vi "BIMS_Collector (2012_01).vi"() -> ()   [LabVIEW 2015]
doc: "This program is currently beta software. It is designed to address the data requirements defined primarily by the DHB Ballistic Test Report.\n\nThe general operation of this program is based on the Ballistics Version 2005 application developed internally by DuPont as a research tool for the Spruance Plant Ballistics Lab in Richmond, VA.\n\nPlease note that the original trigger control logic was modified and no longer depends on a safety interlock system to enable operation of a ballistic test.\n\nDuPont makes no warranties and assumes no liabilities in connection with any use of this program."
uses:
  <vilib>/addons/database/NI_Database_API.lvlib
  <vilib>/addons/database/Connection.llb/Conn Execute.vi
  <vilib>/addons/database/Recordset.llb/Rec Destroy - Connection.vi
  <vilib>/Utility/config.llb/NI_LVConfig.lvlib
  <vilib>/Utility/config.llb/Write Key (I32).vi
  Shot Record.ctl
  BIMS_Collector Globals.vi
  Collector State.ctl
  DataSource.ctl
  <vilib>/registry/registry.llb/Registry RtKey.ctl
  <vilib>/Utility/config.llb/Write Key (String).vi
  <vilib>/addons/database/Connection.llb/DB Tools Open Connec (Path).vi
panel:
  out "Loading":u16(ring)
  in  "runtimeMenusVisible":bool=TRUE
  in  "diagPageVisible":bool
  in  "RESET All":bool
  out "ConfigName":string
  out "TimeNow":string
  in  "EXIT":bool
  in  "mainTabCntrl":enum32{"Setup", "Measure", "History", "System"}(tab)=enum."System"
  in  "SampleEntryTabCntrl":enum32{"Environment", "Sample"}(tab)
  in  "ThreatDetails":u16(ring) caption="Detail"
  in  "ThreatGroups":u16(ring) caption="Group"
  in  "PowderTypes":u16(ring) caption="Type"
  in  "Ballisticians":u16(ring) caption="Ballistician"
  in  "Recorders":u16(ring) caption="Recorder"
  in  "Shooters":u16(ring) caption="Shooter"
  in  "Methods":u16(ring) caption="Method"
  in  "RoomT":sgl caption="Temperature (° F)" format="%.1f"
  in  "RoomHum":sgl caption="Humidity (%)" min=0 max=100 format="%.1f"
  in  "SampleBackings":u16(ring)=3 caption="Type"
  in  "clayCalArray":i16[](array[numeric])=[0, 0, 0, 0, 0] caption="Calibration (mm)" min=0 max=99 format="%02.0f"
  out "clayAverage":sgl caption="Clay Average (mm)" format="%#.1f"
  in  "clayTemp":sgl caption="Clay Temp (° F)" format="%.1f"
  out "threatDetails":T1 caption="Description"
  in  "SampleClamping":u16(ring) caption="Clamping"
  in  "Sample SubTabCntrl":T2(tab)
  in  "SampleID":string caption="Sample ID"
  in  "SampleDimensions":u16(ring) caption="Dimensions"
  in  "ModelMfrs":u16(ring) caption="Manufacturer" items=["DuPont Experimental"]
  in  "SampleTypes":u16(ring) caption="Sample Type"
  in  "Submitters":u16(ring) caption="Submitter"
  in  "ProjectID":string caption="Project ID"
  in  "BackLayers":i32 caption="# of Layers" min=0 max=99 step=5
  in  "FrontLayers":i32 caption="# of Layers" min=0 max=99 step=5
  in  "BackLayer":u16(ring) caption="Back Layer"
  in  "FrontLayer":u16(ring) caption="Front Layer"
  out "totalNumLayers":i32 caption="Total # of Layers" min=0 max=100 step=5
  out "totalBAW":sgl caption="Total BAW (psf)" format="%.2f"
  in  "LayerTabControl":enum32{"1", "2", "3", "4", "5", "6"}(tab) caption="Inner Layers"
  out "fab1_totalWt":sgl caption="Fab1 Wt" min=0 max=99 step=5 format="%.2f"
  out "SampleAttribs_1":T3 caption="fabricAttribs_1"
  in  "Layer_1":T4 caption="Fabric #1" {"plyNum" min=0 max=99 step=5}
  in  "SampleStyle_1":u16(ring)
  in  "Mfr_1":u16(ring) caption="vendor" items=["", "DuPont"]
  in  "layerStitch_1":u16(ring) caption="Stitch" items=["", "1-inch quilt", "2-inch quilt", "Corner Bartack", "Corners", "Custom (Panel)", "Custom (Vest)", "Diamond", "Edge", "n/a", "Normal"]
  out "fab2_totalWt":sgl caption="Fab2 Wt" min=0 max=99 step=5 format="%.2f"
  out "SampleAttribs_2":T3 caption="fabricAttribs_2"
  in  "Layer_2":T4 caption="Fabric #2" {"plyNum" min=0 max=99 step=5}
  in  "SampleStyle_2":u16(ring)
  in  "Mfr_2":u16(ring) caption="vendor" items=["", "DuPont"]
  in  "layerStitch_2":u16(ring) caption="Stitch" items=["", "1-inch quilt", "2-inch quilt", "Corner Bartack", "Corners", "Custom (Panel)", "Custom (Vest)", "Diamond", "Edge", "n/a", "Normal"]
  out "fab3_totalWt":sgl caption="Fab3 Wt" min=0 max=99 step=5 format="%.2f"
  out "SampleAttribs_3":T3 caption="fabricAttribs_3"
  in  "Layer_3":T4 caption="Fabric #3" {"plyNum" min=0 max=99 step=5}
  in  "SampleStyle_3":u16(ring)
  in  "Mfr_3":u16(ring) caption="vendor" items=["", "DuPont"]
  in  "layerStitch_3":u16(ring) caption="Stitch" items=["", "1-inch quilt", "2-inch quilt", "Corner Bartack", "Corners", "Custom (Panel)", "Custom (Vest)", "Diamond", "Edge", "n/a", "Normal"]
  out "fab4_totalWt":sgl caption="Fab4 Wt" min=0 max=99 step=5 format="%.2f"
  out "SampleAttribs_4":T3 caption="fabricAttribs_4"
  in  "Layer_4":T4 caption="Fabric #4" {"plyNum" min=0 max=99 step=5}
  in  "SampleStyle_4":u16(ring)
  in  "Mfr_4":u16(ring) caption="vendor" items=["", "DuPont"]
  in  "layerStitch_4":u16(ring) caption="Stitch" items=["", "1-inch quilt", "2-inch quilt", "Corner Bartack", "Corners", "Custom (Panel)", "Custom (Vest)", "Diamond", "Edge", "n/a", "Normal"]
  out "fab5_totalWt":sgl caption="Fab5 Wt" min=0 max=99 step=5 format="%.2f"
  out "SampleAttribs_5":T3 caption="fabricAttribs_5"
  in  "Layer_5":T4 caption="Fabric #5" {"plyNum" min=0 max=99 step=5}
  in  "SampleStyle_5":u16(ring)
  in  "Mfr_5":u16(ring) caption="vendor" items=["", "DuPont"]
  in  "layerStitch_5":u16(ring) caption="Stitch" items=["", "1-inch quilt", "2-inch quilt", "Corner Bartack", "Corners", "Custom (Panel)", "Custom (Vest)", "Diamond", "Edge", "n/a", "Normal"]
  out "fab6_totalWt":sgl caption="Fab6 Wt" min=0 max=99 step=5 format="%.2f"
  out "SampleAttribs_6":T3 caption="fabricAttribs_6"
  in  "Layer_6":T4 caption="Fabric #6" {"plyNum" min=0 max=99 step=5}
  in  "SampleStyle_6":u16(ring)
  in  "Mfr_6":u16(ring) caption="vendor" items=["", "DuPont"]
  in  "layerStitch_6":u16(ring) caption="Stitch" items=["", "1-inch quilt", "2-inch quilt", "Corner Bartack", "Corners", "Custom (Panel)", "Custom (Vest)", "Diamond", "Edge", "n/a", "Normal"]
  in  "SampleCoverings":u16(ring) caption="Sample Covering" items=["None", "RipStop", "Plastic bag", "Other"]
  in  "Assemblers":u16(ring) caption="Technician"
  in  "Thickness":dbl caption="Thickness (in)" format="%.3f"
  in  "totalSampleWt":sgl caption="Total Weight (lbs)" format="%.3f"
  in  "Comments":string caption="Remarks (optional):"
  in  "TestConditions":u16(ring) caption="Sample Condition"
  in  "shotsTabCntrl":T5(tab)
  in  "Frag Rod":sgl format="%.1f"
  in  "MeasSrc":T6=enum."Screens" caption="Source"
  in  "Drag Corrected":bool=TRUE
  in  "ARM":bool
  in  "readyClock":bool caption="Clock"
  out "Impact/speed":sgl caption="Chronograph 1" min=0 max=10000 step=0.1 format="%.1f"
  out "SHOT STATUS":u16(ring) caption="Penetration" items=["Partial", "Complete"]
  out "residual/speed":sgl caption="Residual" min=0 max=10000 step=0.1 format="%.1f"
  out "SUBMIT DATE/TIME":string
  out "BACKFACE DEPTH":sgl caption="Backface\nDepth" min=0 max=200 step=5
  in  "MeasVelScrnSet1":sgl caption="Set #1" min=0 max=10000 step=0.1 format="%.1f"
  in  "Current/sthotstatus":u16(ring) caption="Penetration" items=["Partial", "Complete"]
  in  "Current/residual/speed":sgl caption="Residual Set" min=0 max=10000 step=0.1 format="%.1f"
  in  "currentDateTime":string caption="Date/Time"
  in  "MeasVelScrnSet2":sgl caption="Set #2" min=0 max=1000000 step=0.1 format="%.1f"
  out "%_Difference":sgl caption="% Vel Diff" format="%.3f"
  in  "backdepth":sgl caption="BF Depth"
  out "Redundant/speed":sgl caption="Chronograph 2" min=0 max=10000 step=0.1 format="%.1f"
  out "Current/avg/speed":sgl caption="Average" min=0 max=1000000 step=0.1 format="%.1f"
  out "Avg/speed":sgl caption="Average" min=0 max=10000 step=0.1 format="%.1f"
  out "SafetyInterlock":cluster{"ARMED":bool}
  out "DC_ factor":sgl=1.0 caption="DC Factor" format="%.4f"
  in  "Barrel Temp":sgl format="%.1f"
  in  "Shot Description":string caption="Description (optional)"
  in  "Powder Loading":sgl caption="Powder Load" min=0 max=100 step=0.1 format="%.3f"
  in  "Shot Angle":u16 max=90 step=1
  out "Projectile Mass":sgl caption="Projectile Mass (grains)" min=0 step=1
  in  "N.I.J":u16(ring) items=["n/a", "PASS", "FAIL"]
  out "Device S/N":string
  in  "addShot":bool caption="RANGE SETUP must be selected before shots can be added."
  in  "loadingUnits":enum32{"grams", "grains"}(radio)
  out "instruct_addShot":string="RANGE SETUP and THREAT must be selected before shots can be added."
  out "Set#1 Separation":sgl=4.0 caption="Outer" format="%.2f"
  out "Set#2 Separation":sgl=4.0 caption="Inner" format="%.2f"
  out "saveReq":string="Number of layers in sample ply specification and number of shots in shots table must be greater than 0 to enable saving."
  in  "VsVr Report":bool caption="Report"
  out "Table of Shots":string[][](table) caption="Shot Table"
  in  "MC Listbox of Shots":i32(listbox)
  in  "saveShots":bool
  in  "clearShots":bool
  out "highPartial":i32 caption="High Partial" min=0 max=10000 step=1
  out "lowComplete":i32 caption="Low Complete" min=0 max=10000 step=1
  out "rangeOfResults":i32 caption="Range of Results" min=0 max=10000 step=1
  out "zmr 2":sgl caption="Low C minus High P" format="%.1f"
  out "computed_V50":sgl caption="V50" format="%.1f"
  out "Pairs":i16 min=0 max=100 step=1
  in  "reportV50":bool caption="Report"
  in  "maxDev":sgl=125.0 caption="Max Deviation" min=0 max=300 step=25
  in  "undoLastShot":bool
  in  "deleteShot":bool
  in  "nextShot":bool
  in  "SHOTS":T7[](array[typedef]) {"Frag Rod" format="%.1f"; "UncorrectedAvgVel_PB" format="%.1f"; "UncorrectedRed_PB" format="%.1f"; "strikeVel_PB" format="%.1f"; "velLoss_PB" format="%.1f"; "avgVel_PB" format="%.1f"; "Redundant_Velocity" format="%.1f"; "Energy Loss (J)" format="%.3e"; "Projectile Mass" min=0 step=1 format="%.4f"; "Corrected residual" format="%.2f"; "Uncorrected Residual" format="%.1f"; "Corrected Impact" format="%.2f"; "Uncorrected Impact" format="%.1f"; "Shot Angle" max=90 step=1; "SHOT STATUS" items=["Partial", "Complete"]; "IMPACT VELOCITY" min=0 max=10000 step=0.1 format="%.1f"; "Barrel Temperature" format="%.1f"; "Powder Loading" format="%.4f"; "RESIDUAL  VELOCITY" min=0 max=10000 step=0.1 format="%.1f"}
  out "velProfile":cluster{dbl, dbl}[](graph) caption="Shot Velocity Measurement Profile"
  out "velCompProf":cluster{"vStrike":dbl, "vA":dbl} caption="Velocity in fps\n(computed)"
  out "velMeasProf":T8 caption="Velocity in fps\n(measured)"
  out "relativeTime":cluster{"ts2":dbl, "ts3":dbl, "ts1":dbl} caption="Relative time\n(microsec)"
  out "displacement":T9={"ds_v2"=6.75, "ds2"=5.0833, "ds_vB"=4.9167, "ds3"=4.75, "ds_vAvg"=6.9167, "ds_v1"=7.0833, "ds1"=8.75, "ds_vA"=8.9167, "ds0"=9.0833} caption="Distance from\ntarget (ft)" {"ds0" format="%_4g"; "ds_vA" format="%_4g"; "ds1" format="%_4g"; "ds_v1" format="%_4g"; "ds_vAvg" format="%_4g"; "ds3" format="%_4g"; "ds_vB" format="%#_4g"; "ds2" format="%#_4g"; "ds_v2" format="%_4g"}
  out "arrIDC":dbl[](array[numeric]) caption="Instantaneous Drag Coefficient"
  in  "rangeSetup":u16(ring)=1 caption="Range Dimensions" items=["Short (small frag)", "Standard (handgun)", "Long (rifle)"]
  out "mid_to_targ_dist":sgl=5.0 caption="Mid To Target (ft)"
  in  "historyTabCntrl":enum32{"Powder Loading", "Panel Search"}(tab)=enum."Panel Search"
  in  "Threat.freeTxt":string caption="Threat"
  in  "Powder.freeTxt":string caption="Powder"
  in  "QueryLoad":bool
  in  "lkupEndDate":timestamp caption="End Date" format="%<%x>T"
  in  "lkupStartDate":timestamp caption="Begin Date" format="%<%x>T"
  out "Vel.vs.Loading":cluster{dbl[], dbl[]}(graph)
  out "v50_table":string[][](table)
  in  "maxRecs":u16=1001 caption="Max # of SHOT Records" min=1 max=10000 step=100
  out "ActualNumRecs":i32=1001 caption="Actual # Returned"
  in  "ThreatSize_0":u16(ring) caption="Threat Size" items=["", "2"]
  in  "panelSearch":bool
  in  "Mfr_0":u16(ring) caption="Manufacturer" items=["", "DuPont"]
  in  "SampleStyle_0":u16(ring) caption="Sample Style"
  in  "srchParams":T10={"maxPanels"=1001, "lkupPanelStartDate"=timestamp(0 s since 1904-01-01), "lkupPanelEndDate"=timestamp(3376658114.0909824 s since 1904-01-01)} {"lkupPanelEndDate" format="%<%x>T"; "lkupPanelStartDate" format="%<%x>T"; "maxPanels" min=1 max=10000 step=100}
  out "actualNumPanels":i32 caption="Actual # Returned"
  out "pastPanels":string[][](table)
  in  "Record #":i32=1 min=0 max=13
  in  "reportV50_History":bool
  out "SampleAttribs_0":T11 caption="fabricAttribs_1"
  in  "Requestors_0":u16(ring) caption="Submitter"
  in  "aboutTabCntrl":enum32{"About ", "Internal Use"}(tab)
  in  "RefreshMetadata":bool
  out "LastShot":i32 caption="Shot"
  out "LastSample":i32 caption="Sample"
  in  "PublishNewRecords":bool
  in  "Folder":string="esvrs11" caption="Publish Folder"
  in  "useBMC":bool caption="Use Message Center?"
  in  "Server":string="esvrs11"
  in  "Site":string="ICE1"
  in  "TestStandards":u16(ring)=2 caption="Standard" items=["n/a", "NIJ 0101.04", "MIL-STD-662F"]
  in  "WeaponTypes":u16(ring) caption="Weapon" items=["", "Universal Receiver", "Other"]
  in  "processShots":bool
  out "DIO":u32=21 format="%.0b"
  in  "line direction map":i32=1792 format="%.0b"
  out "Corrected Average":sgl=1527.9313 format="%.2f"
  out "CorrectedVelScrnSet2":sgl=1551.8816 caption="Corrected Redundant" format="%.2f"
  out "conversion factor":sgl=0.3048037 format="%.5f"
  out "#_completes":i32
  out "#_partials":i32
  in  "percent warning":sgl=1.0 format="%.2f"
  in  "SoftwareVersion":dbl caption="Version" format="%.2f"
  out "impact/ID":u32=83886081 format="%.0x"
  out "residual/ID":u32=83951617 format="%.0x"
  out "Red/ID":u32=84017153 format="%.0x"
  out "correction coefficient":sgl format="%.8f"
  out "Corrected Residual":sgl=751.9905 format="%.2f"
  out "CorrectedVelScrnSet1":sgl=1503.981 format="%.2f"
  out "Barrel to Screen":sgl=7.8333 format="%.2f"
  in  "Set#1_to_Target":sgl=7.083333 format="%.2f"
  out "Residual/Separation":sgl=4.0 format="%.2f"
  in  "Residual/Target Dist":sgl=7.083333 format="%.2f"
  out "Z.M.R.":sgl min=0 step=0.1 format="%.1f"
  in  "old threat":u16
  out "Complete":sgl[](array[numeric]) format="%.2f"
  out "factor array":sgl[](array[numeric]) format="%.4f"
  out "Partial":sgl[](array[numeric]) format="%.2f"
  in  "DAQ Card":i16=1
  in  "Impact Timer":i16 min=0 max=3 step=1
  in  "Redundant Timer":i16=1 min=0 max=3 step=1
  in  "Residual  Timer":i16=2 min=0 max=3 step=1
  out "Impact factor":sgl=1.0 caption="Impact" min=0 max=1 format="%.5f"
  out "Residual factor":sgl=1.0 caption="Residual" min=0 max=1 format="%.5f"
  in  "Areal Density":dbl format="%.2f"
  in  "Areal density text":string
  in  "Fabric Description":string caption="Fabric Desc"
  in  "clayCalib":string="##-##-##-##-##" caption="Calibration"
  in  "lookupRec":bool caption="lookup"
  out "STOP (Shots MC LB)":bool=TRUE
  out "configPath":path=path "P:/Private/My Projects/AFS/BIMS/2008/BIMS_Collector.ini" caption="Configuration Path (INI)"
  in  "minV50":i32=1500 caption="Minimum V50"
  in  "Type of work":string="QC"
  in  "Threat":u16(ring) caption="Threat (long description)"
  out "massUnits":string="GRAMS" caption="Weight Units"
  out "lengthUnits":string="FOOT" caption="Distance Units"
  in  "SampleDescrip":u16(ring) caption="Misc. Sample Description (legacy)"
  in  "serialNum":string caption="Serial #"
  in  "Models":u16(ring) caption="Model #" items=["n/a"]
  in  "InterlockExists":bool=TRUE caption="Safety Interlock Hardware Exist?"
  in  "ScreenSetAvgg":bool caption="Average Screen Sets?"
  in  "Sort by AVG":bool=TRUE caption="Sort shots by average velocity"
  in  "useBallisitican":bool=TRUE caption="Use Ballistician field in Setup?"
  in  "useRecorder":bool caption="Use Recorder field in Setup?"
  in  "useShooter":bool caption="Use Shooter field in Setup?"
  out "SMErr":errorcluster
  out "U/I EvErr":errorcluster
  out "booleanDump":bool
  out "GrainSize":u16 caption="Grain"
  in  "LayerStitchTypes":u16(ring) caption="Stitch" items=["", "Corners"]
  in  "clearErrors":bool
  # "Effectively restarts the application from scratch, as if the user pressed the EXIT button and then restarted the application."
  # "Configured for"
  # "Threat"
  # "*"
  # "*"
  # "Test"
  # "Powder"
  # "*"
  # "Personnel"
  # "Room"
  # "*"
  # "Backing"
  # "*"
  # "*"
  # "*"
  # "Body Side"
  # "Strike Face"
  # "Layer"
  # "Mfr"
  # "Style"
  # "# of Plies"
  # "Lot"
  # "Roll"
  # "Stitch"
  # "Internal ID"
  # "Fiber"
  # "Denier"
  # "Construction"
  # "Weave"
  # "Finish"
  # "Basis weight (oz/yd²)"
  # "Yarn Merge"
  # "Total Weight"
  # "*"
  # "*"
  # "*"
  # "1"
  # "2"
  # "3"
  # "4"
  # "5"
  # "6"
  # "Required"
  # "*"
  # "Timing System"
  # "Shot Parameters"
  # "cm"
  # "deg"
  # "degF"
  # "Velocity Measurements"
  # "Observations"
  # "Screens\nSeparation"
  # "Ft"
  # "Table Functions"
  # "Summary"
  # "Reports"
  # "Test Record"
  # "Edit Shot Records"
  # "Corrected"
  # "Shot #"
  # "t0"
  # "0"
  # "S Strike"
  # "0"
  # "Internal ID#"
  # "Fiber"
  # "Denier"
  # "Pick"
  # "Weave"
  # "Finish"
  # "oz/yd²"
  # "Asset"
  # "DuPont Ballistics Information Management System\n\nBIMS\nEnterprise Edition\n\n\nSample Performance\nData Collector\n\nJanuary 2012"
  # "DuET Measurement System Technologies\nDUCOM 8 695-2330 for technical support\n\nDuPont Company"
  # "Last Assigned\nRecord Numbers"
  # "Deployment Configuration"
  # "Data items support Point Blank requirements:"
  # "Correction Factors"
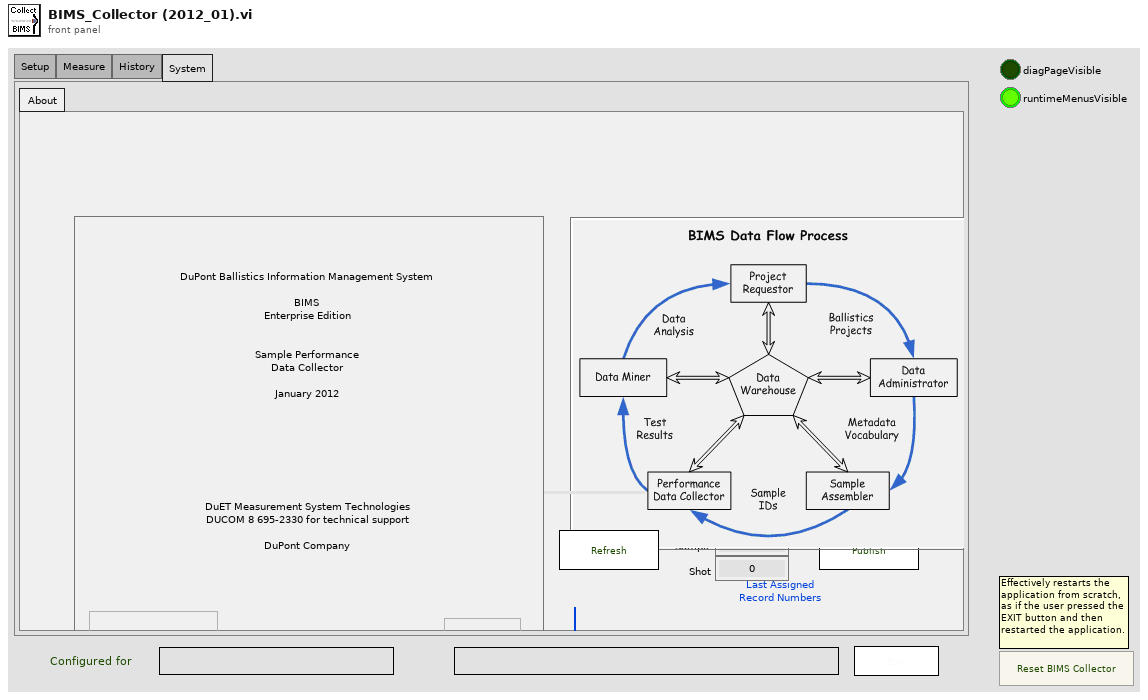
[diagram p1: front panel]
types:
  T1 = cluster{"barrelLength":string, "dragCorrection":string, "detailDescription":string, "barrelCaliber":string, "grainSize":string, "Make":string, "Model":string}
  T2 = enum32{"General Specification", "Ply Specification", "Preparation"}
  T3 = cluster{"Fabric.fiber":string, "Fabric.denier":string, "pick":string, "weave":string, "finish":string, "ozPerYd2":string, "fabricID_DHB":string, "yarnMerge":string}
  T4 = cluster{"plyNum":i32, "LotNum":string, "RollNum":string}
  T5 = enum32{"Ready-Aim-Fire", "Shots Table", "Edit", "Instantaneous DC"}
  T6 = typedef "DataSource.ctl" = enum16{"Simulated", "Radar", "Screens"}
  T7 = typedef "Shot Record.ctl" = cluster{"Uncorrected Impact":sgl, "Uncorrected Residual":sgl, "avgVel_PB":sgl, "IMPACT VELOCITY":sgl, "RESIDUAL  VELOCITY ":sgl, "Shot Description":string, "Powder Loading ":sgl, "Barrel Temperature":sgl, "TIME / DATE":string, "shot order":i32, "SHOT STATUS":u16, "Shot Angle":u16, "Corrected Impact":sgl, "Corrected residual":sgl, "Projectile Mass":sgl, "usedv50":bool, "Energy Loss (J)":sgl, "BackFace\nDepth":sgl, "BackFace\nDiameter":sgl, "Redundant_Velocity":sgl, "velLoss_PB":sgl, "strikeVel_PB":sgl, "UncorrectedRed_PB":sgl, "CorrectedRed_PB":sgl, "UncorrectedAvgVel_PB":sgl, "V50userExcl":bool, "Frag Rod":sgl}
  T8 = cluster{"v2":dbl, "vB":dbl, "vOuter":dbl, "v1":dbl, "vA":dbl, "vInner":dbl}
  T9 = cluster{"ds_v2":dbl, "ds2":dbl, "ds_vB":dbl, "ds3":dbl, "ds_vAvg":dbl, "ds_v1":dbl, "ds1":dbl, "ds_vA":dbl, "ds0":dbl}
  T10 = cluster{"maxPanels":u16, "lkupPanelStartDate":timestamp, "lkupPanelEndDate":timestamp}
  T11 = cluster{"Fabric.fiber":string, "Fabric.denier":string, "pick":string, "weave":string, "finish":string, "ozPerYd2":string, "fabricID_DHB":string, "asset":string}
  T12 = typedef "Collector State.ctl" = enum16{"POLL", "INITIALIZE", "V50 Report or GET Record", "VsVr Report", "SAVE SHOTS", "ADD SHOT", "CLEAR SHOTS", "NEXT SHOT", "DELETE SHOT", "READY CLOCK", "PROC SHOTS", "CHECK DAQ"}
  T13 = typedef "Collector State.ctl" = enum16{"POLL", "INITIALIZE", "V50 Report or GET Record", "VsVr Report", "SAVE SHOTS", "ADD SHOT", "CLEAR SHOTS", "NEXT SHOT", "DELETE SHOT", "PROCESS SHOTS", "READY CLOCK", "CHECK DAQ"}
  T14 = enum8{"Enabled", "Disabled", "Disabled and Grayed Out"}
  T15 = enum32{"Page Enabled", "Page Disabled", "Page Disabled & Grayed"}
  T16 = typedef "Registry RtKey.ctl" = enum32{"HKEY_CLASSES_ROOT", "HKEY_CURRENT_USER", "HKEY_LOCAL_MACHINE", "HKEY_USERS", "HKEY_PERFORMANCE_DATA", "HKEY_CURRENT_CONFIG", "HKEY_DYN_DATA"}
  T17 = cluster{"[0]":string, "[1]":string, "[2]":string, "[3]":string, "[4]":string, "[5]":string, "[6]":string, "[7]":string, "[8]":string, "[9]":string}[]
  T18 = cluster{"[0]":string, "[1]":string, "[2]":string, "[3]":string, "[4]":string, "[5]":string, "[6]":string, "[7]":string, "[8]":string}[]
  T19 = cluster{"Fabric.fiber":string, "Fabric.denier":string, "pick":string, "weave":string, "finish":string, "ozPerYd2":string, "fabricID_DHB":string, "yarnMerge":string}[]
  T20 = cluster{"Uncorrected Impact":bool, "Uncorrected Residual":bool, "avgVel_PB":bool, "IMPACT VELOCITY":bool, "RESIDUAL  VELOCITY ":bool, "Shot Description":bool, "Powder Loading ":bool, "Barrel Temperature":bool, "TIME / DATE":bool, "shot order":bool, "SHOT STATUS":bool, "Shot Angle":bool, "Corrected Impact":bool, "Corrected residual":bool, "Projectile Mass":bool, "usedv50":bool, "Energy Loss (J)":bool, "BackFace\nDepth":bool, "BackFace\nDiameter":bool, "Redundant_Velocity":bool, "velLoss_PB":bool, "strikeVel_PB":bool, "UncorrectedRed_PB":bool, "CorrectedRed_PB":bool, "UncorrectedAvgVel_PB":bool, "V50userExcl":bool, "Frag Rod":bool}
  T21 = cluster{"SampleTypes":refnum<vi>, "SampleDescrip":refnum<vi>}
  T22 = cluster{"max dev":sgl, "residual separation":sgl, "Set#1 Separation":sgl, "Set#2 Separation ":sgl, "impact target dist":sgl, "resid target dist":sgl, "barrel screen dist":sgl, "midpt_to_target_dist":sgl}
  T23 = cluster{"fiber":string, "denier":string, "pick":string, "weave":string, "finish":string, "ozPerYd2":string, "internal_ID":string, "asset":string}[]
  T24 = cluster{"numOfPlies":i32, "LotNum":string, "RollNum":string}[]
  T25 = cluster{string, string, string, string, string, string, string, string, "clayCalib":string, string}
  T26 = cluster{string, string, string, string, string, string, string}
  T27 = cluster{"SampleID":string, "element":string, "Type of work":string, "serialNum":string, "element":string, string, string, string, "element":string, string}
  T28 = cluster{"SampleID":string, "element":string, string, string, string, "element":string}
  T29 = cluster{"[0]":string, "[1]":string, "[2]":string, "[3]":string, "[4]":string, "[5]":string, "[6]":string, "[7]":string, "[8]":string, "[9]":string}
  T30 = cluster{"[0]":string, "[1]":string, "[2]":string, "[3]":string, "[4]":string, "[5]":string, "[6]":string, "[7]":string, "[8]":string}
  T31 = cluster{"element":string, "element":string, "grainSize":string, "element":string, "barrelLength":string, string, "element":string, "element":string, "element":string}
  T32 = cluster{"element":string, "grainSize":string, "element":string, "barrelLength":string, string, "element":string}
  T33 = typedef "NI_Database_API.lvlib/Conn ObjectReference.ctl" = refnum<k1>
  T34 = typedef "NI_Database_API.lvlib/Rec ObjectReference.ctl" = refnum<k1>
  T35 = typedef "NI_LVConfig.lvlib/Config Data RefNum.ctl" = refnum<k1>
  T36 = cluster{"task ID out":u32, "task ID out":u32, "task ID out":u32}
  T37 = enum32{"invalid app kind", "Development System", "Run Time System", "Student Edition", "Embedded LabVIEW", "Evaluation", "Custom"}
  T38 = typedef "LVRowAndColumnTypeDef.ctl" = cluster{"Row":i32, "Column":i32}
  T39 = cluster{"barrelLength":string, "dragCoefficient":string, "detailDescription":string, "barrelCaliber":string, "grainSize":string, "Make":string, "Model":string}
  T40 = cluster{"fiber":string, "denier":string, "construction":string, "weave":string, "finish":string, "ozPerYd2":string, "fabricStyle_DHB":string, "yarnMerge":string}
  T41 = cluster{"plyNum":i32, "LotNum":string, "RollNum":string}[]
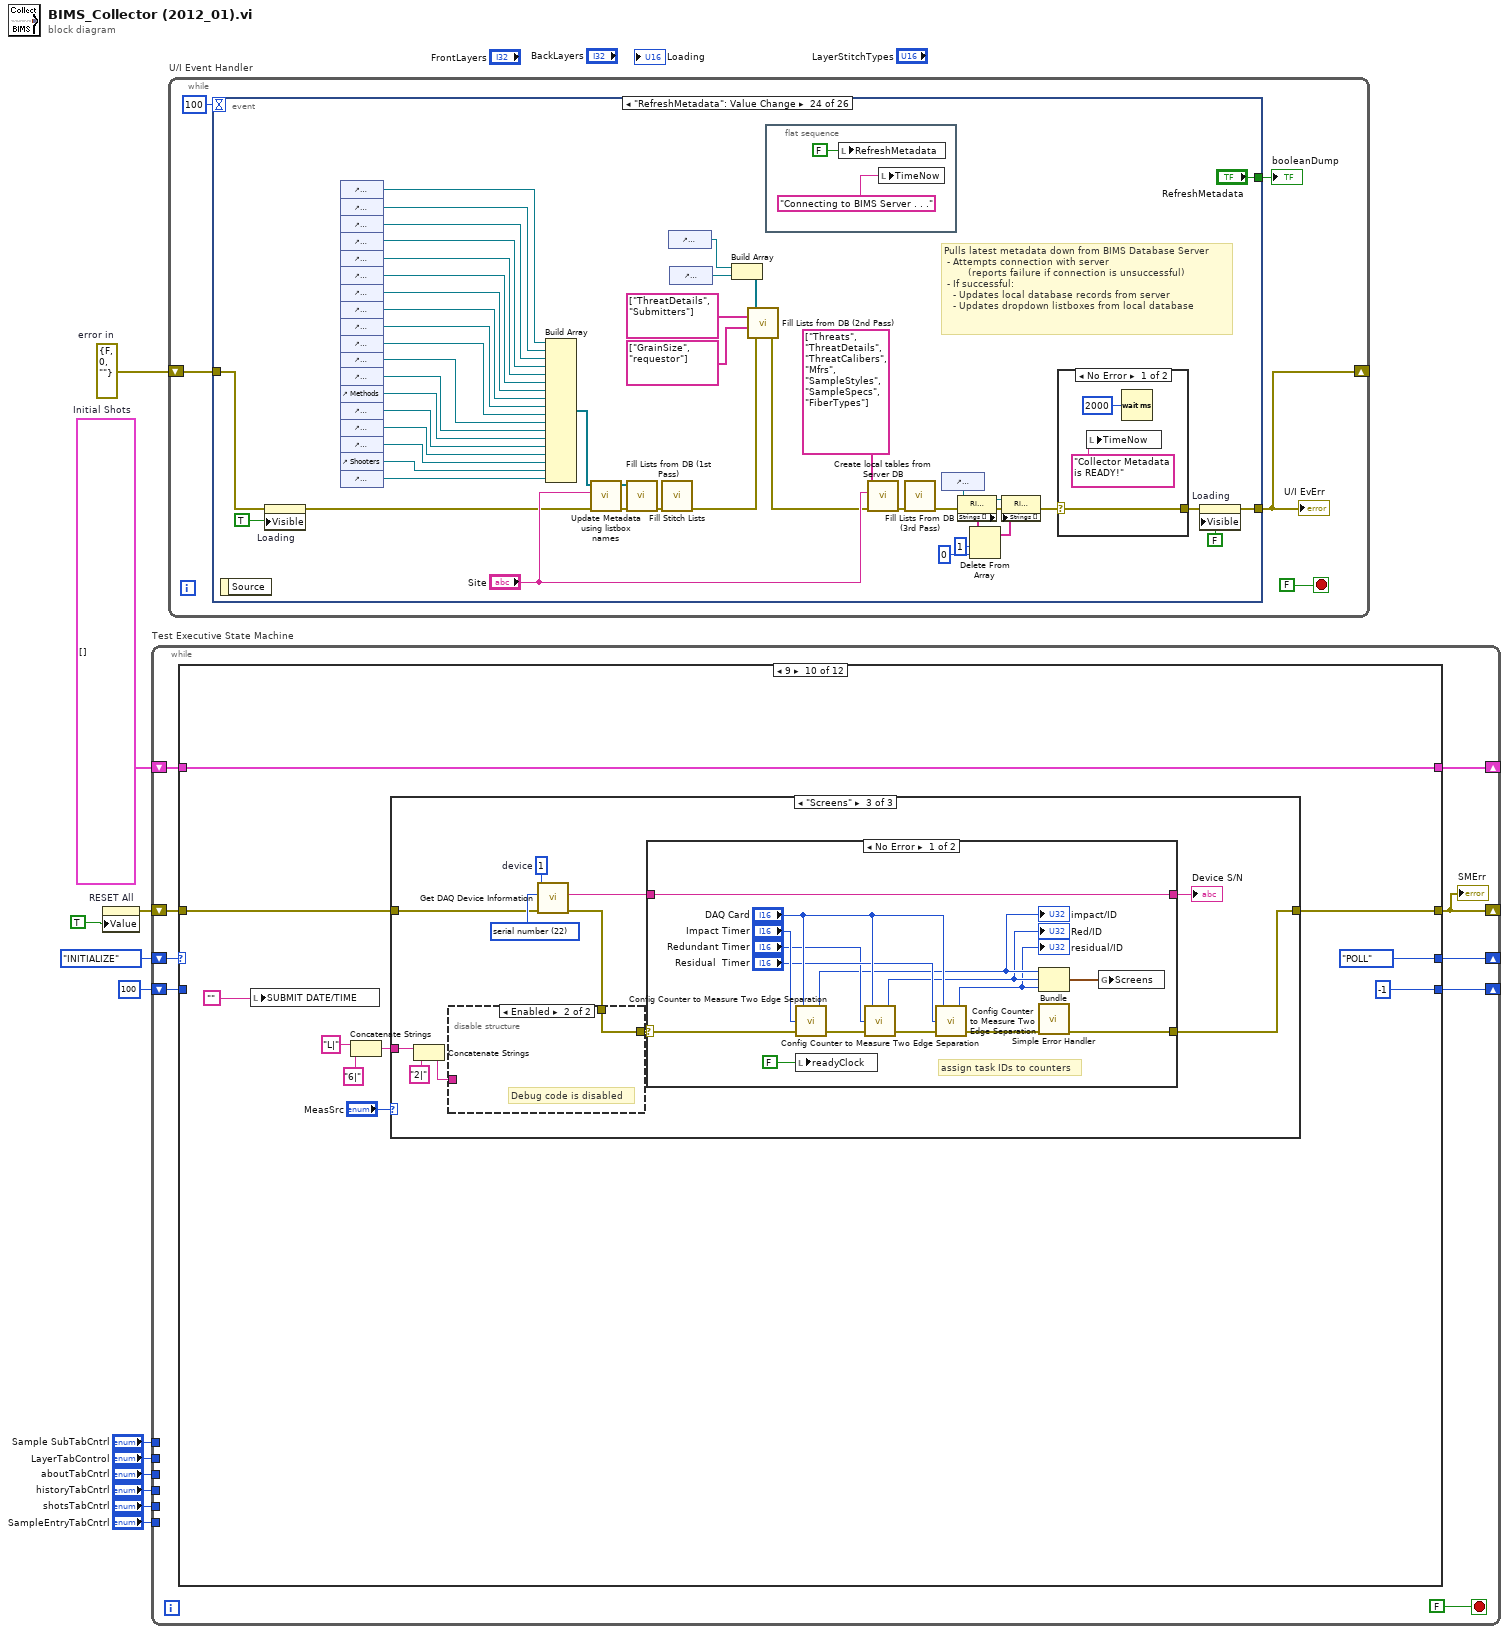
[diagram p0: block diagram]
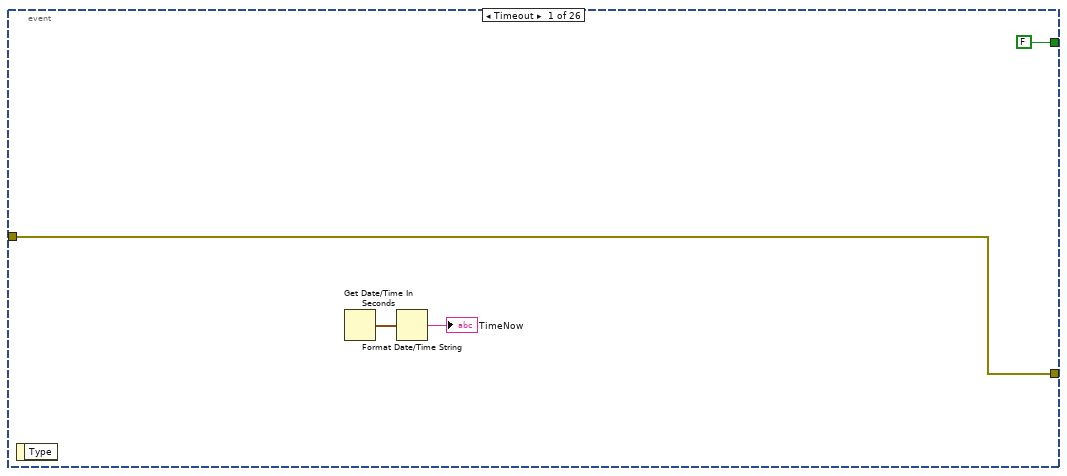
[diagram p2: hidden frame]
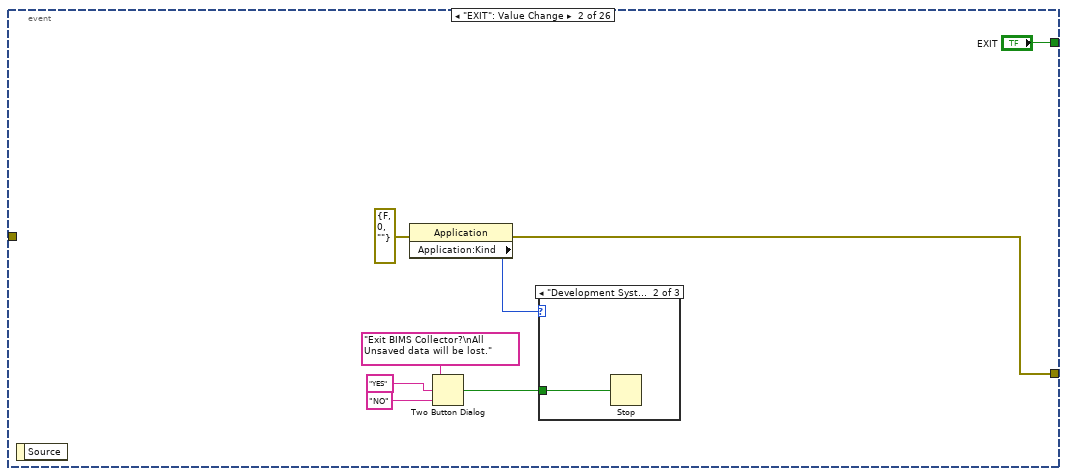
[diagram p3: hidden frame]
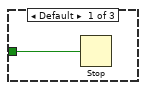
[diagram p4: hidden frame]
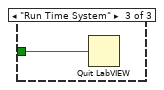
[diagram p5: hidden frame]
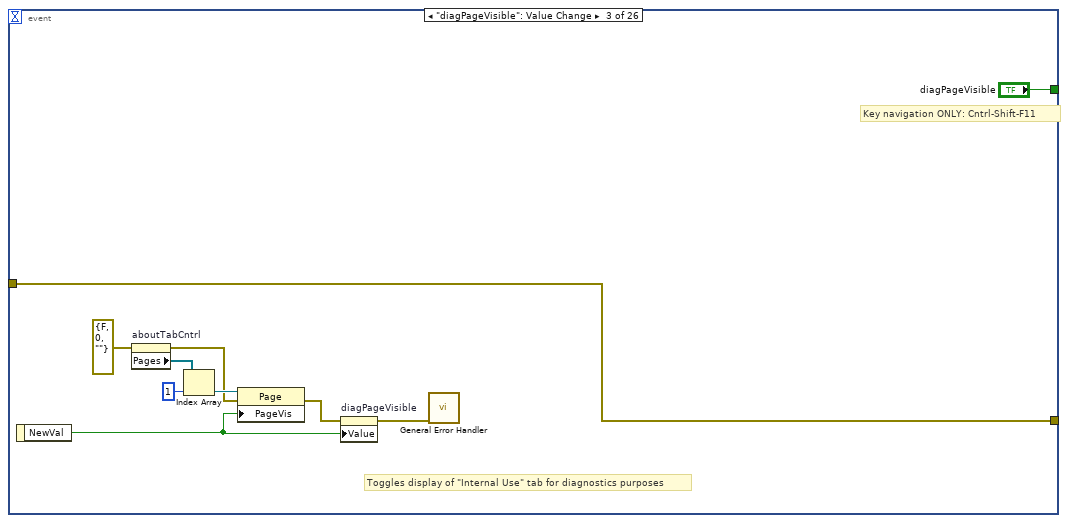
[diagram p6: hidden frame]
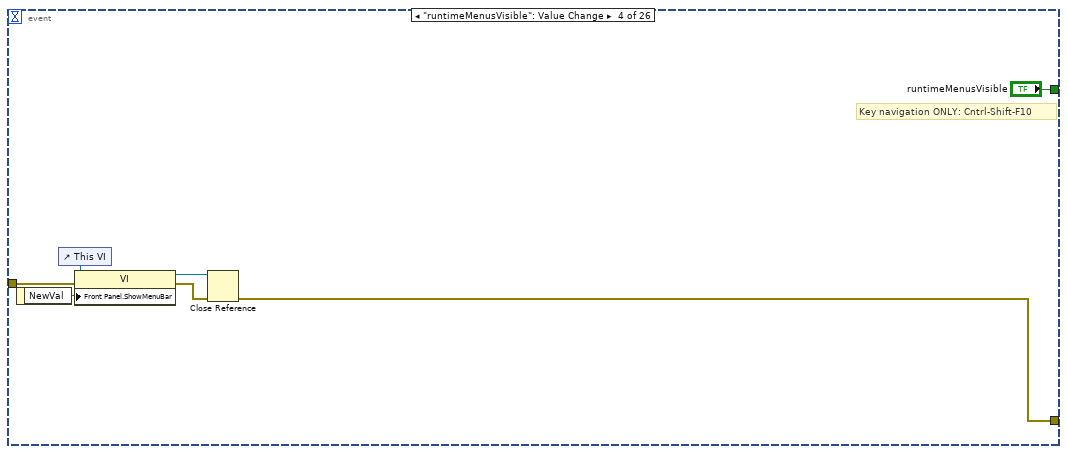
[diagram p7: hidden frame]
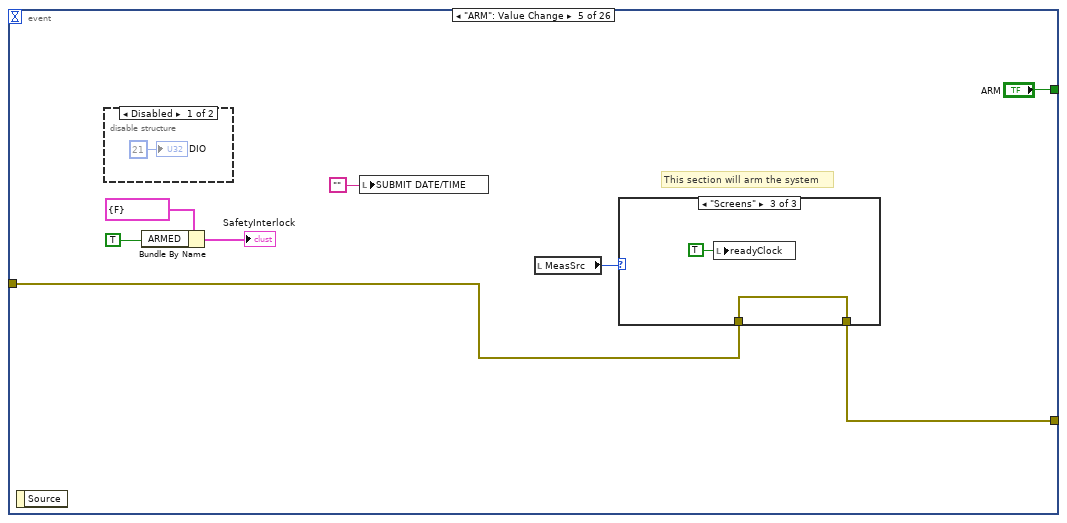
[diagram p8: hidden frame]
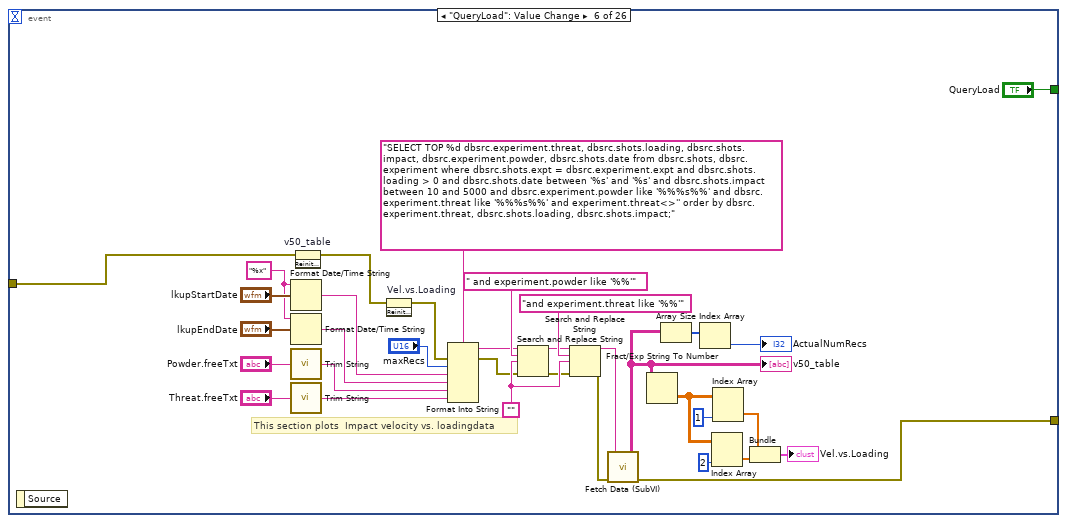
[diagram p12: hidden frame]
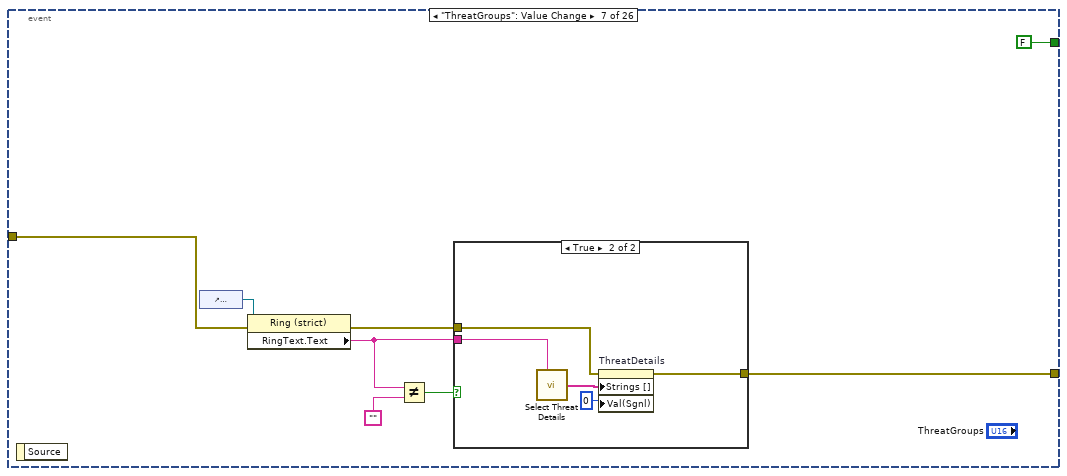
[diagram p13: hidden frame]
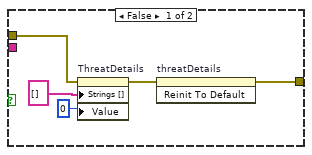
[diagram p14: hidden frame]
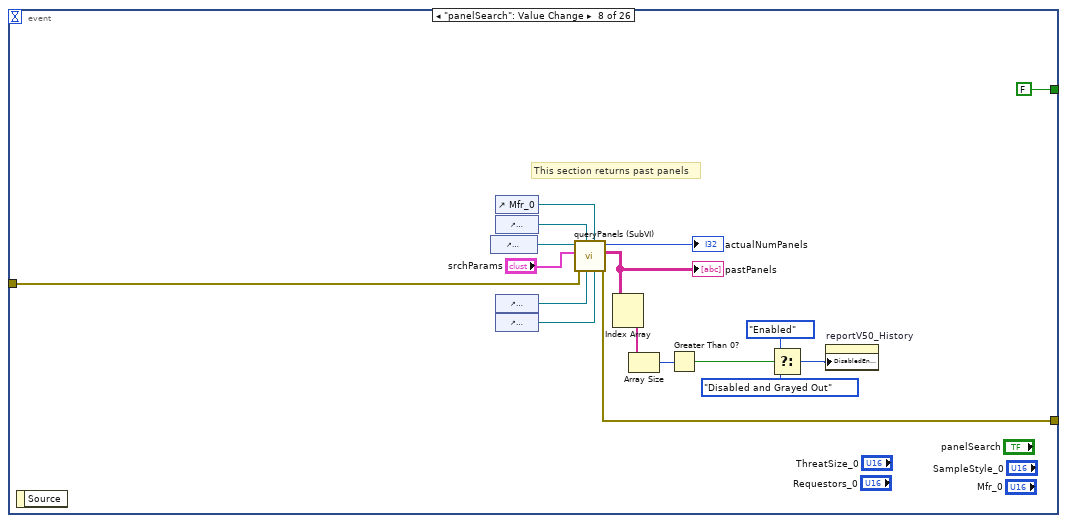
[diagram p15: hidden frame]
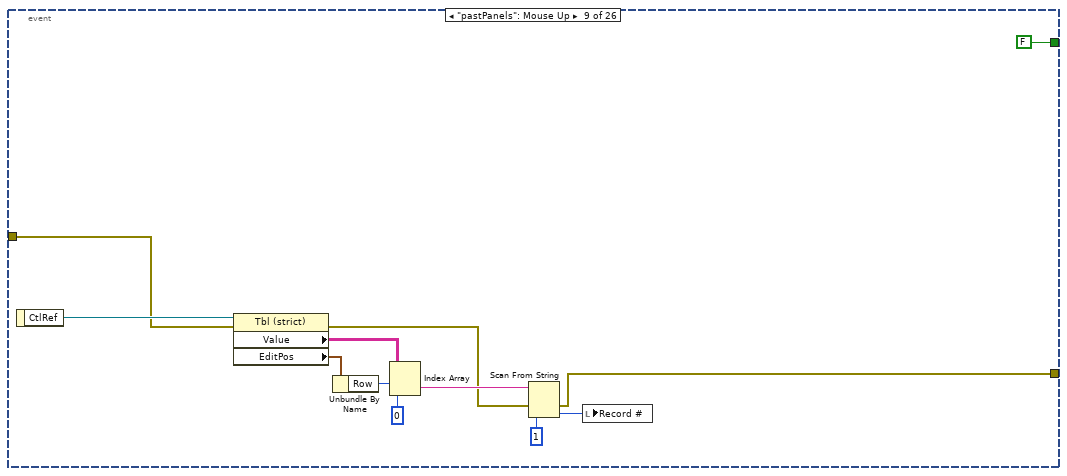
[diagram p16: hidden frame]
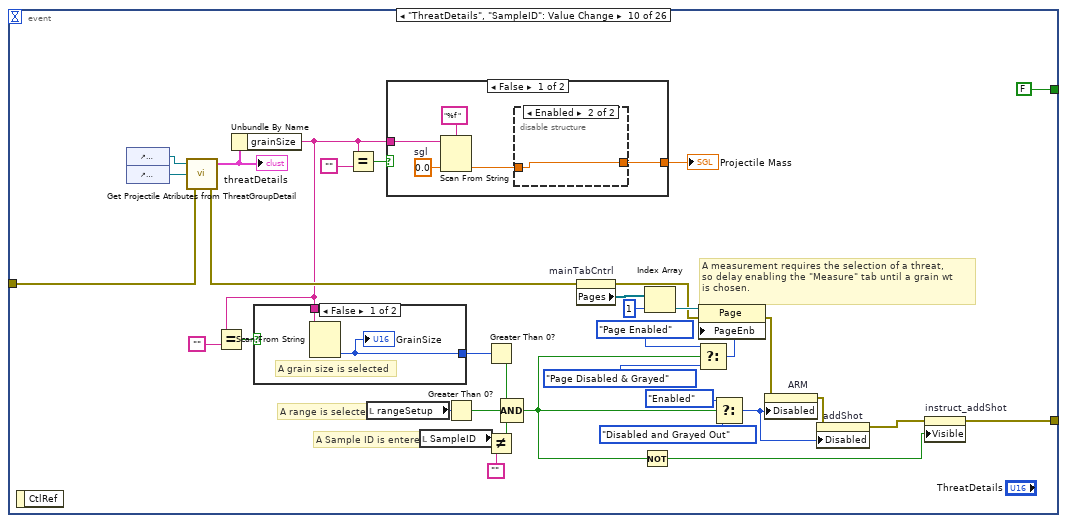
[diagram p17: hidden frame]
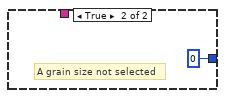
[diagram p18: hidden frame]
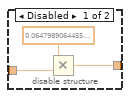
[diagram p19: hidden frame]
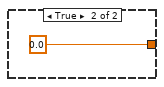
[diagram p20: hidden frame]
diagram:
  w7 = errorcluster {"status"=FALSE, "code"=0, "source"=""}  # error in
  w8 = T7[] []  # Initial Shots
  n1 = property on="RESET All" class="Bool (strict)"("Value"=TRUE ("RESET")) -> (error out=w10:errorcluster)  [unwired: 2 in, 1 out]
  n2 = while "Test Executive State Machine" {
    shift-left: 100 -> [w18]
    shift-right: [w19] -> _
    shift-left: Collector_State."INITIALIZE" ("progState") -> [w15]
    shift-right: [w20] -> _
    shift-right: [w16] -> _
    shift-left: w8 -> [w17]
    shift-right: [w13] -> _
    shift-left: w10 -> [w14]
    tunnel: "LayerTabControl" -> [_]
    tunnel: "aboutTabCntrl" -> [_]
    tunnel: "historyTabCntrl" -> [_]
    tunnel: "SampleEntryTabCntrl" -> [_]
    tunnel: "Sample SubTabCntrl" -> [_]
    tunnel: "shotsTabCntrl" -> [_]
    stop <- FALSE stop-if-true
    n3 = case shown="9" w15 {
      tunnel: [w24 w144 Collector_State."POLL" ("progState") Collector_State."POLL" ("progState") w1089 Collector_State."PROCESS SHOTS" ("progState") Collector_State."POLL" ("progState") Collector_State."PROCESS SHOTS" ("progState") Collector_State."PROCESS SHOTS" ("progState") Collector_State."POLL" ("progState") Collector_State."POLL" ("progState") w1752] -> w20
      tunnel: [-1 -1 ("index of element") -1 ("index of element") -1 ("index of element") w1088 -1 ("index of element") -1 -1 ("index of element") -1 ("index of element") -1 -1 ("index of element") w1751] -> w19
      tunnel: w18 -> [_ w145 _ _ _ _ _ _ _ _ _ _]
      tunnel: w17 -> [w28 w143 w295 w836 w1082 w1345 w1390 w1413 w1419 w1472 w1524 w1755]
      tunnel: [w27 w142 w295 w836 w1081 w1332 w1394 w1412 w1418 w1472 w1528 w1755] -> w16
      tunnel: w14 -> [_ w138 w292 w834 w1084 w1340 w1386 w1402 w1414 w1468 w1523 w1746]
      tunnel: [w36 w139 w291 w833 w1083 w1338 w1386 w1400 w1415 w1467 w1522 w1747] -> w13
      frame 0, Default {
        w29 = Collector_State."POLL"  # progStateType
        w49 = TRUE  # element
        w52 = 4  # SAVE
        # "This section checks for any buttons, maintains routine check of the paramters"
        n4 = case shown="\"Measure\"" "mainTabCntrl" {
          tunnel: w28 -> [_ w108 _ _]
          frame "Setup", Default {
            n5 = control-ref of="layerStitch_1"() -> (w76:refnum<vi>)
            n6 = control-ref of="layerStitch_2"() -> (w75:refnum<vi>)
            n7 = control-ref of="layerStitch_3"() -> (w74:refnum<vi>)
            n8 = control-ref of="layerStitch_4"() -> (w73:refnum<vi>)
            n9 = control-ref of="layerStitch_5"() -> (w72:refnum<vi>)
            n10 = control-ref of="layerStitch_6"() -> (w71:refnum<vi>)
            n11 = control-ref of="SampleStyle_0"() -> (w69:refnum<vi>)
            n12 = control-ref of="SampleStyle_1"() -> (w90:refnum<vi>)
            n13 = control-ref of="SampleStyle_2"() -> (w91:refnum<vi>)
            n14 = control-ref of="SampleStyle_3"() -> (w92:refnum<vi>)
            n15 = control-ref of="SampleStyle_4"() -> (w93:refnum<vi>)
            n16 = control-ref of="SampleStyle_5"() -> (w94:refnum<vi>)
            n17 = control-ref of="SampleStyle_6"() -> (w95:refnum<vi>)
            n18 = Build Array(w69, w90, w91, w92, w93, w94, w95) -> (w88:refnum<vi>[])
            n19 = global write "BIMS_Collector Globals.vi" "SampleStyles"(w88) -> ()
            n20 = Build Array(w76, w75, w74, w73, w72, w71) -> (w77:refnum<vi>[])
            n21 = global write "BIMS_Collector Globals.vi" "LayerStitchTypeRefs"(w77) -> ()
            n22 = local read "SampleAttribs_1"() -> (w82:T3)
            n23 = local read "SampleAttribs_2"() -> (w84:T3)
            n24 = local read "SampleAttribs_3"() -> (w85:T3)
            n25 = local read "SampleAttribs_4"() -> (w86:T3)
            n26 = local read "SampleAttribs_5"() -> (w87:T3)
            n27 = local read "SampleAttribs_6"() -> (w83:T3)
            n28 = Build Array(w82, w84, w85, w86, w87, w83) -> (w81:T19)
            n29 = global write "BIMS_Collector Globals.vi" "SampleAttribs"(w81) -> ()
            n30 = local read "Fabric Description"() -> (w80:string)
            n31 = control-ref of="Mfr_0"() -> (w70:refnum<vi>)
            n32 = control-ref of="Mfr_1"() -> (w101:refnum<vi>)
            n33 = control-ref of="Mfr_2"() -> (w100:refnum<vi>)
            n34 = control-ref of="Mfr_3"() -> (w99:refnum<vi>)
            n35 = control-ref of="Mfr_4"() -> (w98:refnum<vi>)
            n36 = control-ref of="Mfr_5"() -> (w97:refnum<vi>)
            n37 = control-ref of="Mfr_6"() -> (w96:refnum<vi>)
            n38 = String Subset(string=w80, length (rest)=75 ("length (rest)")) -> (substring=w79:string)  [unwired: 1 out]
            n39 = Build Array(w70, w101, w100, w99, w98, w97, w96) -> (w89:refnum<vi>[])
            n40 = local write "Fabric Description"(w79) -> ()
            n41 = global write "BIMS_Collector Globals.vi" "Mfrs"(w89) -> ()
          }
          frame "Measure" {
            # "Disable and gray out the \"Save\" button\nIF the shot table has no shots, \nOR if there are no plies; otherwise, enable it."
            # "Disable and gray out the \"Clear Shots\" button\nIF the shot table has no shots; otherwise, enable it."
            n42 = Array Size(array=w108) -> (size(s)=w115:i32)
            n43 = Equal To 0?(x=w115) -> (x = 0?=w102:bool)
            n44 = property on="saveReq" class="Str"("Visible"=w102) -> ()  [unwired: 2 in, 2 out]
            n45 = Select(t=T14."Disabled and Grayed Out" ("Disabled"), s=w102, f=T14."Enabled" ("Disabled")) -> (s? t:f=w114:T14)
            n46 = Select(t=T14."Disabled and Grayed Out" ("Disabled"), s=w102, f=T14."Enabled" ("Disabled")) -> (s? t:f=w103:T14)
            n47 = property on="reportV50" class="Bool"("Disabled"=w103) -> ()  [unwired: 2 in, 2 out]
            n48 = property on="saveShots" class="Bool"("Disabled"=w103) -> ()  [unwired: 2 in, 2 out]
            n49 = property on="clearShots" class="Bool"("Disabled"=w114) -> ()  [unwired: 2 in, 2 out]
            n50 = local read "Shot Description"() -> (w111:string)
            n51 = String Subset(string=w111, length (rest)=30 ("length (rest)")) -> (substring=w109:string)  [unwired: 1 out]
            n52 = local write "Shot Description"(w109) -> ()
            "SHOT STATUS" <- "Current/sthotstatus"
            "BACKFACE DEPTH" <- "backdepth"
          }
          frame "History" {
          }
          frame "System" {
          }
        }
        n53 = Get Date/Time String(want seconds? (F)=TRUE) -> (date string=w34:string, time string=w35:string)  [unwired: 2 in]
        n54 = call <vilib>:"Space Constant.vi"() -> ("String"=w32:string)
        n55 = Concatenate Strings(w34, w32, w35) -> (w33:string)
        n56 = local write "currentDateTime"(w33) -> ()
        n57 = Or(x="undoLastShot", y="deleteShot") -> (x .or. y?=w47:bool)
        n58 = Or(x="reportV50", y="reportV50_History") -> (x .or. y?=w55:bool)
        n59 = flat-sequence {
          tunnel: [w68] -> w30
          frame #0 {
            n60 = Wait (ms)(milliseconds to wait=u32 200 ("millisecond timer value")) -> ()  [unwired: 1 out]
          }
          frame #1 {
            n61 = local read "SMErr"() -> (w68:errorcluster)
          }
        }
        n62 = Build Array("RESET All", w55, "VsVr Report", "saveShots", "addShot", "clearShots", "nextShot", w47, "processShots", "readyClock") -> (w50:bool[])
        n63 = Search 1D Array(1D array=w50, element=w49) -> (index of element=w60:i32)  [unwired: 1 out]
        n64 = Increment(x=w60) -> (x+1=w61:i32)
        n65 = Equal?(x=w61, y=w52) -> (x = y?=w53:bool)
        n66 = case shown="False" w53 {
          tunnel: w61 -> [w117 w129]
          tunnel: [w118 w134] -> w59
          tunnel: w30 -> [w116 w125]
          tunnel: [w116 w123] -> w36
          frame False {
            w120 = 0  # Not Found
            n67 = Equal?(x=w117, y=w120) -> (x = y?=w119:bool)
            n68 = case shown="True" w119 {
              tunnel: w117 -> [w121 _]
              tunnel: [w121 w122] -> w118
              frame False {
              }
              frame True {
                w122 = 11  # CheckDAQ
                # "USUAL SCENARIO"
              }
            }
          }
          frame True {
            # "Before allowing data record to be saved,\nprompt user to validate."
            n69 = call "Get Last Record (SubVI).vi"("error in"=w125) -> ("error out"=w124:errorcluster, "experiment record"=w126:i32, "shot record"=w127:i32)  [unwired: 2 out]
            n70 = local write "LastShot"(w127) -> ()
            n71 = local write "LastSample"(w126) -> ()
            n72 = To Double Precision Float(number=w126) -> (double precision float=w128:dbl)
            n73 = Two Button Dialog(message="Are ALL Data Valid?", 1:"NO" ("F button name (\"Cancel\")"), 2:"YES" ("T button name (\"OK\")")) -> (T button?=w133:bool)
            n74 = property on="Record #" class="DigNum (strict)"(error in=w124, "Maximum"=w128) -> (error out=w123:errorcluster)  [unwired: 1 in, 1 out]
            n75 = case shown="False" w133 {
              tunnel: [0 ("index of element") w136] -> w134
              tunnel: w129 -> [_ w136]
              frame False {
                # "POLL"
              }
              frame True {
              }
            }
          }
        }
        n76 = local read "SHOTS"() -> (w27:T7[])
        n77 = To Variant(anything=w59) -> (Variant=w58:variant)
        n78 = for {
          tunnel: w28 -> [w65] mode=indexing
          tunnel: w27 -> [w66] mode=indexing
          tunnel: [w62] -> w26 mode=indexing
          n79 = Not Equal?(x=w66, y=w65) -> (x != y?=w64:T20)
          n80 = Cluster To Array(cluster=w64) -> (array=w63:bool[])
          n81 = Or Array Elements(Boolean array=w63) -> (logical OR=w62:bool)
        }
        n82 = Variant To Data(type=w29, Variant=w58) -> (data=w25:T12)  [unwired: 1 in, 1 out]
        n83 = Or Array Elements(Boolean array=w26) -> (logical OR=w22:bool)
        n84 = Select(t=Collector_State."PROCESS SHOTS" ("progStateType"), s=w22, f=w25) -> (s? t:f=w24:u16)
        "STOP (Shots MC LB)" <- TRUE ("STOP (Shots MC LB)")
      }
      frame 1 {
        # "This section reads the ini file"
        n85 = case shown="100" w145 {
          tunnel: [w151 w170] -> w146
          tunnel: [w149 w170] -> w141
          tunnel: w138 -> [w148 w162]
          tunnel: [w147 w162] -> w137
          frame 0, Default {
            n86 = local read "RESET All"() -> (w150:bool)
            n87 = case shown="True" w150 {
              tunnel: [TRUE w158] -> w151
              tunnel: [FALSE w158] -> w149
              tunnel: w148 -> [w152 w155]
              tunnel: [w152 w155] -> w147
              frame False {
                # "Refresh"
              }
              frame True {
                n88 = Two Button Dialog(message="Resetting will remove all unsaved data.\n\nDo you really  want to reset? ", 1:"NO" ("F button name (\"Cancel\")"), 2:"YES" ("T button name (\"OK\")")) -> (T button?=w158:bool)
              }
            }
          }
          frame 100 {
            w170 = TRUE  # Reset ALL
            n89 = property on="Loading" class="Ring (strict)"("Visible"=FALSE) -> ()  [unwired: 2 in, 2 out]
            n90 = control-ref of="Mfr_0"() -> (w160:refnum<vi>)
            n91 = control-ref of="Mfr_1"() -> (w169:refnum<vi>)
            n92 = control-ref of="Mfr_2"() -> (w168:refnum<vi>)
            n93 = control-ref of="Mfr_3"() -> (w167:refnum<vi>)
            n94 = control-ref of="Mfr_4"() -> (w166:refnum<vi>)
            n95 = control-ref of="Mfr_5"() -> (w165:refnum<vi>)
            n96 = control-ref of="Mfr_6"() -> (w164:refnum<vi>)
            n97 = Build Array(w160, w169, w168, w167, w166, w165, w164) -> (w163:refnum<vi>[])
            n98 = global write "BIMS_Collector Globals.vi" "Mfrs"(w163) -> ()
          }
        }
        n99 = case shown="True" w146 {
          tunnel: [Collector_State."POLL" ("progState") w207] -> w144
          tunnel: w143 -> [w173 _]
          tunnel: [w173 "SHOTS"] -> w142
          tunnel: w141 -> [_ w208]
          tunnel: [w171 w187] -> w139
          tunnel: w137 -> [w171 w206]
          frame False {
            n100 = local write "RESET All"(FALSE ("RESET")) -> ()
          }
          frame True {
            n101 = case shown="True" w208 {
              selector: w208 -> [_ w235]
              tunnel: [w218 w235] -> w188
              tunnel: [w217 w250] -> w189
              tunnel: w206 -> [w217 w237]
              tunnel: [w216 w234] -> w186
              frame False {
                w218 = FALSE  # Reset All
                # "Refresh"
                n102 = local read "configPath"() -> (w216:path)
              }
              frame True {
                # "This section resets\nentire program"
                # "Reset ALL"
                n103 = control-ref of="This VI"() -> (w227:refnum<vi>)
                n104 = invoke on="Invoke Node" class="VI" method="Default Vals.Reinit All"(reference=w227, error in=w237) -> (reference out=w226:refnum<vi>, error out=w225:errorcluster)  [unwired: 1 in, 1 out]
                n105 = property class="VI"(reference=w226, error in=w225, "Front Panel.ShowMenuBar"=FALSE ("Front Panel Window:Show Menu Bar")) -> (reference out=w223:refnum<vi>, error out=w221:errorcluster)
                n106 = property on="mainTabCntrl" class="TabCtl (strict)"() -> (error out=w229:errorcluster, "Pages"=w231:refnum<vi>[])  [unwired: 2 in, 1 out]
                n107 = control-ref of="ScreenSetAvgg"() -> (w245:refnum<vi>)
                n108 = control-ref of="InterlockExists"() -> (w246:refnum<vi>)
                n109 = control-ref of="useBallisitican"() -> (w247:refnum<vi>)
                n110 = control-ref of="useRecorder"() -> (w248:refnum<vi>)
                n111 = control-ref of="useShooter"() -> (w249:refnum<vi>)
                n112 = control-ref of="useBMC"() -> (w220:refnum<vi>)
                n113 = Close Reference(reference=w223, error in (no error)=w221) -> (error out=w222:errorcluster)
                n114 = Index Array(array=w231, index=1) -> (element=w233:refnum<vi>)
                n115 = call "RegReadParams.vi"("ScreenSetAveraging_Ref"=w245, "useBMC_Ref"=w220, "InterlockExist_Ref"=w246, "errorIN"=w222, "useShooter_Ref"=w249, "useRecorder_Ref"=w248, "useBallistician_Ref"=w247) -> ("error out"=w244:errorcluster)  [unwired: 4 out]
                n116 = control-ref of="Server"() -> (w236:refnum<vi>)
                n117 = control-ref of="ConfigName"() -> (w240:refnum<vi>)
                n118 = control-ref of="Site"() -> (w238:refnum<vi>)
                n119 = control-ref of="Folder"() -> (w219:refnum<vi>)
                n120 = property on="Property Node" class="Page"(reference=w233, error in=w229, "PageEnb"=T15."Page Disabled & Grayed" ("Page Enabled State")) -> (error out=w228:errorcluster)  [unwired: 1 out]
                n121 = Build Array(w240, w238, w236, w219) -> (w241:refnum<vi>[])
                n122 = call "InitStringValuesFromRegistry(SubVI).vi"("error in"=w244, "String References"=w241, "subkey"="SOFTWARE\\DuPont\\BIMS-08\\Collector", "root key (HKEY_LOCAL_MACHINE)"=Registry_RtKey."HKEY_LOCAL_MACHINE") -> ("error out"=w243:errorcluster)  [unwired: 3 out]
                n123 = property on="minV50" class="DigNum (strict)"(error in=w228, "Visible"=w235) -> ()  [unwired: 1 in, 2 out]
                n124 = Current VI's Path() -> (path=w253:path)
                n125 = call "Initialize (SubVI).vi"("path"=w253, "error IN"=w243) -> ("pathConfigOUT"=w234:path, "lengthUnits"=→"lengthUnits":string, "massUnits"=→"massUnits":string, "error out"=w250:errorcluster)  [unwired: 1 out]
                "configPath" <- w234
              }
            }
            n126 = control-ref of="Threat"() -> (w192:refnum<vi>)
            n127 = control-ref of="SampleTypes"() -> (w194:refnum<vi>)
            n128 = control-ref of="SampleDescrip"() -> (w201:refnum<vi>)
            n129 = call "Get Threats (SubVI).vi"("pathConfigIN"=w186, "refThreat"=w192, "error in"=w189) -> ("pathConfigOUT"=w196:path, "factorOut"=→"factor array":sgl[], "error out"=w199:errorcluster)  [unwired: 4 out]
            n130 = Bundle("SampleTypes"=w194, "SampleDescrip"=w201) -> (w200:T21)  [unwired: 1 out]
            n131 = call "Fill Lists from INI (SubVI).vi"("clusterListboxes"=w200, "error in"=w199, "pathConfigIN"=w196) -> ("error out"=w198:errorcluster, "pathConfigOUT"=w197:path)  [unwired: 4 out]
            n132 = call "Read Parameters.vi"("error in (no error)"=w198, "appended path"=w197) -> ("error out"=w191:errorcluster, "rangeParams"=w193:T22)  [unwired: 4 out]
            n133 = Unbundle(w193) -> ("max dev"=w175:sgl, "residual separation"=→"Residual/Separation":sgl, "Set#1 Separation"=→"Set#1 Separation":sgl, "Set#2 Separation"=→"Set#2 Separation":sgl, "impact target dist"=w179:sgl, "resid target dist"=w180:sgl, "barrel screen dist"=→"Barrel to Screen":sgl, "midpt_to_target_dist"=→"mid_to_targ_dist":sgl)
            n134 = property on="Ballisticians" class="Ring (strict)"("Visible"="useBallisitican") -> ()  [unwired: 2 in, 2 out]
            n135 = property on="Shooters" class="Ring (strict)"("Visible"="useShooter") -> ()  [unwired: 2 in, 2 out]
            n136 = property on="Recorders" class="Ring (strict)"("Visible"="useRecorder") -> ()  [unwired: 2 in, 2 out]
            n137 = property on="RefreshMetadata" class="Bool (strict)"(error in=w191, "Val(Sgnl)"=TRUE) -> (error out=w183:errorcluster)  [unwired: 1 in, 1 out]
            n138 = local write "Residual/Target Dist"(w180) -> ()
            n139 = local write "maxDev"(w175) -> ()
            n140 = local write "Set#1_to_Target"(w179) -> ()
            n141 = case shown="True" w188 {
              tunnel: [Collector_State."POLL" ("progState") w279] -> w207
              tunnel: [w254 w264] -> w205
              tunnel: w183 -> [w254 w273]
              tunnel: w186 -> [_ w263]
              tunnel: "useBMC" -> [_ w262]
              frame False {
                # "Refresh"
              }
              frame True {
                w256 = T14."Disabled and Grayed Out" ("Disabled")
                # "Reset ALL"
                n142 = global read "BIMS_Collector Globals.vi" "SampleStyles"() -> (w266:refnum<vi>[])
                n143 = case shown="False" w262 {
                  tunnel: w263 -> [_ w281]
                  frame False {
                  }
                  frame True {
                    n144 = Path To String(path=w281) -> (string=w282:string)
                    n145 = call "Ballistics Message Center.vi"("INI File Name"=w282) -> ()
                  }
                }
                n146 = call "Get Last Record (SubVI).vi"("error in"=w273) -> ("error out"=w265:errorcluster, "experiment record"=w271:i32, "shot record"=→"LastShot":i32)  [unwired: 2 out]
                "LastSample" <- w271
                n147 = local read "MeasSrc"() -> (w280:T6)
                n148 = local read "InterlockExists"() -> (w278:bool)
                n149 = control-ref of="ThreatDetails"() -> (w261:refnum<vi>)
                n150 = control-ref of="SampleStyle_0"() -> (w268:refnum<vi>)
                n151 = control-ref of="ThreatGroups"() -> (w267:refnum<vi>)
                n152 = local read "SafetyInterlock"() -> (w276:cluster{"ARMED":bool})
                n153 = Bundle By Name(cluster=w276, "ARMED"=FALSE) -> (w275:cluster{"ARMED":bool})
                n154 = To Double Precision Float(number=w271) -> (double precision float=w270:dbl)
                n155 = property on="Record #" class="DigNum (strict)"(error in=w265, "Maximum"=w270) -> (error out=w264:errorcluster)  [unwired: 1 in, 1 out]
                n156 = case shown="\"Simulated\", Default" w280 {
                  tunnel: [Collector_State."POLL" ("progState") Collector_State."POLL" ("progState") Collector_State."READY CLOCK" ("progState")] -> w279
                  frame "Simulated", Default {
                  }
                  frame "Radar" {
                  }
                  frame "Screens" {
                    # "check for PCI 6602"
                  }
                }
                n157 = Build Array (concatenate)(w261, w268, w267, w266) -> (w269:refnum<vi>[])
                n158 = local write "SafetyInterlock"(w275) -> ()
                n159 = Select(t=T14."Enabled" ("Disabled"), s=w278, f=T14."Disabled and Grayed Out" ("Disabled")) -> (s? t:f=w277:T14)
                n160 = for {
                  tunnel: w269 -> [w283] mode=indexing
                  n161 = property on="Property Node" class="Ring (strict)"(reference=w283, "Strings []"=string[] []) -> ()  [unwired: 1 in, 2 out]
                }
                n162 = property on="addShot" class="Bool"("Disabled"=T14."Enabled") -> ()  [unwired: 2 in, 2 out]
                n163 = property on="undoLastShot" class="Bool"("Disabled"=w256) -> ()  [unwired: 2 in, 2 out]
                n164 = property on="saveShots" class="Bool"("Disabled"=w256) -> ()  [unwired: 2 in, 2 out]
                n165 = property on="clearShots" class="Bool"("Disabled"=w256) -> ()  [unwired: 2 in, 2 out]
                n166 = property on="ARM" class="Bool"("Disabled"=w277) -> ()  [unwired: 2 in, 2 out]
                n167 = property on="SafetyInterlock" class="Clust (strict)"("Disabled"=w277) -> ()  [unwired: 2 in, 2 out]
                n168 = property on="saveReq" class="Str"("Visible"=TRUE) -> ()  [unwired: 2 in, 2 out]
              }
            }
            n169 = call <vilib>:"General Error Handler.vi"("error in (no error)"=w205) -> ("error out"=w187:errorcluster)  [unwired: 2 in, 12 out]
            n170 = flat-sequence {
              tunnel: w187 -> [w210]
              frame #0 {
                n171 = local read "ConfigName"() -> (w211:string)
                n172 = case shown="No Error" w210 {
                  tunnel: [w214 "NOT READY!" ("ConfigName")] -> w212
                  tunnel: w211 -> [w214 _]
                  frame No Error {
                    n173 = Wait (ms)(milliseconds to wait=u32 1000) -> ()  [unwired: 1 out]
                  }
                  frame Error {
                  }
                }
                "ConfigName" <- w212
              }
            }
            "saveReq" <- "Number of layers in sample ply specification and number of shots in shots table must be greater than 0 to enable saving." ("saveReq")
          }
        }
      }
      frame 2 {
        # "The custom Excel template file is \nexpected in the C:\\Ballistics folder."
        n174 = case shown="False" "lookupRec" {
          selector: "lookupRec" -> [_ w815]
          tunnel: [w338 w805] -> w319
          tunnel: [w337 w791] -> w318
          tunnel: [w336 w808] -> w317
          tunnel: [w335 w748] -> w316
          tunnel: [w334 w806] -> w315
          tunnel: [w333 w768] -> w314
          tunnel: [w332 w755] -> w301
          tunnel: [w331 w757] -> w300
          tunnel: [w330 w758] -> w299
          tunnel: [w329 "Record #"] -> w298
          tunnel: [w328 w807] -> w297
          tunnel: [w327 w757] -> w290
          tunnel: w295 -> [w326 _]
          tunnel: [w325 w780] -> w293
          tunnel: w292 -> [w325 w781]
          tunnel: [w324 w753] -> w288
          frame False {
            n175 = stacked-sequence {
              tunnel: [_ _ _ _ _ w668] -> w333
              tunnel: [_ w407 _ _ _ _] -> w337
              tunnel: [_ _ _ _ w512 _] -> w334
              tunnel: [_ _ _ w458 _ _] -> w335
              tunnel: [_ _ w429 _ _ _] -> w336
              tunnel: [w350 _ _ _ _ _] -> w338
              tunnel: [_ _ _ _ _ w674] -> w332
              tunnel: [_ _ _ _ _ w670] -> w331
              tunnel: [_ _ _ _ _ w669] -> w330
              tunnel: [_ _ _ _ _ w673] -> w329
              tunnel: [_ _ _ _ _ w672] -> w328
              tunnel: [_ _ _ _ _ w671] -> w327
              tunnel: w326 -> [_ _ w428 _ w511 _]
              frame #0 {
                # "Need to remove first element\nsince it's associated with the \nhistory page."
                # "FABRIC"
                n176 = local read "fab1_totalWt"() -> (w353:sgl)
                n177 = local read "fab3_totalWt"() -> (w355:sgl)
                n178 = local read "fab5_totalWt"() -> (w357:sgl)
                n179 = global read "BIMS_Collector Globals.vi" "SampleStyles"() -> (w341:refnum<vi>[])
                n180 = global read "BIMS_Collector Globals.vi" "Mfrs"() -> (w346:refnum<vi>[])
                n181 = local read "fab2_totalWt"() -> (w354:sgl)
                n182 = local read "fab4_totalWt"() -> (w356:sgl)
                n183 = local read "fab6_totalWt"() -> (w358:sgl)
                n184 = global read "BIMS_Collector Globals.vi" "LayerStitchTypeRefs"() -> (w348:refnum<vi>[])
                n185 = global read "BIMS_Collector Globals.vi" "SampleAttribs"() -> (w339:T23)
                n186 = global read "BIMS_Collector Globals.vi" "LayerSpecs"() -> (w349:T24)
                n187 = Delete From Array(array=w341, length=1, index=0) -> (array with subset deleted=w340:refnum<vi>[])  [unwired: 1 out]
                n188 = Delete From Array(array=w346, length=1, index=0) -> (array with subset deleted=w347:refnum<vi>[])  [unwired: 1 out]
                n189 = Build Array(w353, w354, w355, w356, w357, w358) -> (w352:sgl[])
                n190 = for {
                  tunnel: w352 -> [w362] mode=indexing
                  tunnel: [w370] -> w351 mode=indexing
                  tunnel: w339 -> [w369] mode=indexing
                  tunnel: w349 -> [w368] mode=indexing
                  tunnel: w347 -> [w367] mode=indexing
                  tunnel: w340 -> [w366] mode=indexing
                  tunnel: w348 -> [w365] mode=indexing
                  n191 = call "Dropdown Selection (SubVI).vi"("reference"=w367) -> ("element"=w360:string)
                  n192 = call "Dropdown Selection (SubVI).vi"("reference"=w366) -> ("element"=w364:string)
                  n193 = Equal?(x="", y=w360) -> (x = y?=w359:bool)
                  n194 = call "Dropdown Selection (SubVI).vi"("reference"=w365) -> ("element"=w363:string)
                  n195 = case shown="False" w359 {
                    tunnel: [w389 w391] -> w370
                    tunnel: w369 -> [w388 _]
                    tunnel: w368 -> [w387 _]
                    tunnel: w364 -> [w381 _]
                    tunnel: w363 -> [w376 _]
                    tunnel: w362 -> [w374 _]
                    tunnel: w360 -> [w373 _]
                    frame False {
                      n196 = Unbundle By Name(w387) -> ("numOfPlies"=w375:i32, "LotNum"=w384:string, "RollNum"=w385:string)
                      n197 = Unbundle By Name(w388) -> ("internal_ID"=w379:string, "fiber"=w380:string, "denier"=w383:string, "pick"=w382:string, "weave"=w377:string, "finish"=w378:string, "ozPerYd2"=w386:string)
                      n198 = Format Into String(w375) -> (resulting string=w372:string)  [unwired: 3 in, 1 out]
                      n199 = Format Into String(w374) -> (resulting string=w371:string)  [unwired: 3 in, 1 out]
                      n200 = Build Array(w372, w373, w381, w379, w380, w383, w382, w377, w378, w384, w385, w386, w371, w376) -> (w389:string[])
                    }
                    frame True {
                      n201 = Initialize Array("", 14 ("dimension size")) -> (w391:string[])
                    }
                  }
                }
                n202 = Transpose 2D Array(2D array=w351) -> (transposed array=w350:string[][])
              }
              frame #1 {
                w393 = "%.1f" ("format string")
                # "muzzel / midpoint"
                # "muzzle / scr#1"
                # "muzzle / target"
                # "scr#2 / target"
                # "RANGE"
                n203 = local read "Set#1 Separation"() -> (w400:sgl)
                n204 = local read "mid_to_targ_dist"() -> (w397:sgl)
                n205 = local read "Barrel to Screen"() -> (w394:sgl)
                n206 = local read "clayAverage"() -> (w415:sgl)
                n207 = Divide(x=w400, y=sgl 2.0) -> (x/y=w395:sgl)
                n208 = local read "RoomHum"() -> (w410:sgl)
                n209 = local read "clayTemp"() -> (w413:sgl)
                n210 = local read "clayCalib"() -> (w416:string)
                n211 = local read "RoomT"() -> (w411:sgl)
                n212 = Add(x=w394, y=w397) -> (x+y=w401:sgl)
                n213 = Subtract(x=w394, y=w395) -> (x-y=w396:sgl)
                n214 = Subtract(x=w397, y=w395) -> (x-y=w398:sgl)
                n215 = Format Into String(w401) -> (resulting string=w402:string)  [unwired: 3 in, 1 out]
                n216 = Format Into String(w396) -> (resulting string=w403:string)  [unwired: 3 in, 1 out]
                n217 = Format Into String(w400) -> (resulting string=w404:string)  [unwired: 3 in, 1 out]
                n218 = Format Into String(w398) -> (resulting string=w405:string)  [unwired: 3 in, 1 out]
                n219 = Format Into String(w397) -> (resulting string=w406:string)  [unwired: 3 in, 1 out]
                n220 = Format Into String(w410) -> (resulting string=w408:string)  [unwired: 3 in, 1 out]
                n221 = Format Into String(format string=w393, w411) -> (resulting string=w409:string)  [unwired: 2 in, 1 out]
                n222 = Format Into String(format string=w393, w413) -> (resulting string=w412:string)  [unwired: 2 in, 1 out]
                n223 = Format Into String(format string=w393, w415) -> (resulting string=w414:string)  [unwired: 2 in, 1 out]
                n224 = Bundle(w402, w403, w404, w405, w406, w408, w409, w412, "clayCalib"=w416, w414) -> (w417:T25)  [unwired: 1 out]
                n225 = Cluster To Array(cluster=w417) -> (array=w407:string[])
              }
              frame #2 {
                # "RESULTS"
                n226 = control-ref of="Methods"() -> (w418:refnum<vi>)
                n227 = call "Dropdown Selection (SubVI).vi"("reference"=w418) -> ("element"=w419:string)
                n228 = for {
                  tunnel: w428 -> [w456] mode=indexing
                  tunnel: [w455] -> w427 mode=indexing
                  tunnel: [w454] -> w426
                  i -> [w454]
                  n229 = Unbundle By Name(w456) -> ("BackFace\nDepth"=w455:sgl)
                }
                n230 = Increment(x=w426) -> (x+1=w424:i32)
                n231 = Add Array Elements(numeric array=w427) -> (sum=w425:sgl)
                n232 = To Single Precision Float(number=w424) -> (single precision float=w423:sgl)
                n233 = Divide(x=w425, y=w423) -> (x/y=w422:sgl)
                n234 = Format Into String(format string="%1.1f", w422) -> (resulting string=w421:string)  [unwired: 2 in, 1 out]
                n235 = case shown="\"V50\"" w419 {
                  tunnel: [w444 w453] -> w431
                  tunnel: w421 -> [w432 w452]
                  frame "V50" {
                    w438 = "%1d" ("format string")
                    n236 = local read "Z.M.R."() -> (w436:sgl)
                    n237 = Less Than 0?(x=w436) -> (x < 0?=w437:bool)
                    n238 = local read "rangeOfResults"() -> (w440:i32)
                    n239 = local read "computed_V50"() -> (w443:sgl)
                    n240 = local read "lowComplete"() -> (w441:i32)
                    n241 = local read "highPartial"() -> (w442:i32)
                    n242 = case shown="True" w437 {
                      tunnel: w436 -> [w449 _]
                      tunnel: [w449 sgl 0.0 ("Z.M.R.")] -> w435
                      frame False {
                      }
                      frame True {
                      }
                    }
                    n243 = Format Into String(format string="%1.1f", w443) -> (resulting string=w447:string)  [unwired: 2 in, 1 out]
                    n244 = Format Into String(format string=w438, w442) -> (resulting string=w446:string)  [unwired: 2 in, 1 out]
                    n245 = Format Into String(format string=w438, w441) -> (resulting string=w445:string)  [unwired: 2 in, 1 out]
                    n246 = Format Into String(format string=w438, w440) -> (resulting string=w448:string)  [unwired: 2 in, 1 out]
                    n247 = Format Into String(format string="%1.1f", w435) -> (resulting string=w434:string)  [unwired: 2 in, 1 out]
                    n248 = Bundle(w447, w446, w445, w448, w434, w432, w432) -> (w444:T26)  [unwired: 1 out]
                  }
                  frame Default {
                    w451 = "" ("Empty String Constant")
                    n249 = Bundle(w451, w451, w451, w451, w451, w452, w452) -> (w453:T26)  [unwired: 1 out]
                  }
                }
                n250 = Cluster To Array(cluster=w431) -> (array=w430:string[])
                n251 = Build Array(w430) -> (w429:string[][])
              }
              frame #3 {
                # "SAMPLE"
                n252 = local read "Site"() -> (w457:string)
                n253 = case shown="\"SPR1\"" w457 {
                  tunnel: [w460 w484 w497] -> w458
                  frame "ICE1", Default {
                    # "PB Req"
                    n254 = control-ref of="Methods"() -> (w461:refnum<vi>)
                    n255 = call "Dropdown Selection (SubVI).vi"("reference"=w461) -> ("element"=w463:string)
                    n256 = Equal?(x=w463, y="V50") -> (x = y?=w462:bool)
                    n257 = local read "totalSampleWt"() -> (w473:sgl)
                    n258 = case shown="True" w462 {
                      tunnel: ["n/a" w483] -> w467
                      frame False {
                      }
                      frame True {
                        n259 = local read "minV50"() -> (w482:i32)
                        n260 = Format Into String(w482) -> (resulting string=w483:string)  [unwired: 3 in, 1 out]
                      }
                    }
                    n261 = control-ref of="SampleDimensions"() -> (w479:refnum<vi>)
                    n262 = control-ref of="SampleCoverings"() -> (w480:refnum<vi>)
                    n263 = control-ref of="Models"() -> (w466:refnum<vi>)
                    n264 = local read "serialNum"() -> (w475:string)
                    n265 = local read "SampleID"() -> (w477:string)
                    n266 = local read "Thickness"() -> (w470:dbl)
                    n267 = local read "totalBAW"() -> (w469:sgl)
                    n268 = call "Dropdown Selection (SubVI).vi"("reference"=w479) -> ("element"=w476:string)
                    n269 = call "Dropdown Selection (SubVI).vi"("reference"=w466) -> ("element"=w465:string)
                    n270 = call "Dropdown Selection (SubVI).vi"("reference"=w480) -> ("element"=w474:string)
                    n271 = Format Into String(w473) -> (resulting string=w472:string)  [unwired: 3 in, 1 out]
                    n272 = Format Into String(w470) -> (resulting string=w471:string)  [unwired: 3 in, 1 out]
                    n273 = Format Into String(w469) -> (resulting string=w468:string)  [unwired: 3 in, 1 out]
                    n274 = Bundle("SampleID"=w477, "element"=w476, "Type of work"="Type of work", "serialNum"=w475, "element"=w465, w472, w471, w468, "element"=w474, w467) -> (w478:T27)  [unwired: 1 out]
                    n275 = Cluster To Array(cluster=w478) -> (array=w460:string[])
                  }
                  frame "SPR0" {
                    n276 = local read "totalSampleWt"() -> (w490:sgl)
                    n277 = control-ref of="SampleDimensions"() -> (w495:refnum<vi>)
                    n278 = control-ref of="SampleCoverings"() -> (w496:refnum<vi>)
                    n279 = local read "SampleID"() -> (w493:string)
                    n280 = local read "Thickness"() -> (w487:dbl)
                    n281 = local read "totalBAW"() -> (w486:sgl)
                    n282 = call "Dropdown Selection (SubVI).vi"("reference"=w495) -> ("element"=w492:string)
                    n283 = call "Dropdown Selection (SubVI).vi"("reference"=w496) -> ("element"=w491:string)
                    n284 = Format Into String(w490) -> (resulting string=w489:string)  [unwired: 3 in, 1 out]
                    n285 = Format Into String(w487) -> (resulting string=w488:string)  [unwired: 3 in, 1 out]
                    n286 = Format Into String(w486) -> (resulting string=w485:string)  [unwired: 3 in, 1 out]
                    n287 = Bundle("SampleID"=w493, "element"=w492, w489, w488, w485, "element"=w491) -> (w494:T28)  [unwired: 1 out]
                    n288 = Cluster To Array(cluster=w494) -> (array=w484:string[])
                  }
                  frame "SPR1" {
                    n289 = local read "totalSampleWt"() -> (w503:sgl)
                    n290 = control-ref of="SampleDimensions"() -> (w508:refnum<vi>)
                    n291 = control-ref of="SampleCoverings"() -> (w509:refnum<vi>)
                    n292 = local read "SampleID"() -> (w506:string)
                    n293 = local read "Thickness"() -> (w500:dbl)
                    n294 = local read "totalBAW"() -> (w499:sgl)
                    n295 = call "Dropdown Selection (SubVI).vi"("reference"=w508) -> ("element"=w505:string)
                    n296 = call "Dropdown Selection (SubVI).vi"("reference"=w509) -> ("element"=w504:string)
                    n297 = Format Into String(w503) -> (resulting string=w502:string)  [unwired: 3 in, 1 out]
                    n298 = Format Into String(w500) -> (resulting string=w501:string)  [unwired: 3 in, 1 out]
                    n299 = Format Into String(w499) -> (resulting string=w498:string)  [unwired: 3 in, 1 out]
                    n300 = Bundle("SampleID"=w506, "element"=w505, w502, w501, w498, "element"=w504) -> (w507:T28)  [unwired: 1 out]
                    n301 = Cluster To Array(cluster=w507) -> (array=w497:string[])
                  }
                }
              }
              frame #4 {
                n302 = local read "Site"() -> (w510:string)
                n303 = case shown="\"SPR1\"" w510 {
                  tunnel: [w522 w572 w624] -> w512
                  tunnel: w511 -> [w515 w565 w617]
                  frame "ICE1", Default {
                    # "SHOT TABLE"
                    n304 = control-ref of="Methods"() -> (w514:refnum<vi>)
                    n305 = call "Dropdown Selection (SubVI).vi"("reference"=w514) -> ("element"=w513:string)
                    n306 = for {
                      tunnel: w515 -> [w554] mode=indexing
                      shift-right: [w531] -> _
                      shift-left: T17 [] -> [w533]
                      tunnel: [w531] -> w518
                      tunnel: w513 -> [w527]
                      n307 = Unbundle By Name(w554) -> ("shot order"=w553:i32, "Powder Loading"=w552:sgl, "Uncorrected Impact"=w551:sgl, "UncorrectedRed_PB"=w550:sgl, "UncorrectedAvgVel_PB"=w549:sgl, "velLoss_PB"=w548:sgl, "strikeVel_PB"=w547:sgl, "SHOT STATUS"=w536:u16, "usedv50"=w546:bool, "Shot Angle"=w528:u16, "BackFace\nDepth"=w529:sgl)
                      n308 = case shown="\"V50\"" w527 {
                        tunnel: w546 -> [w556 _]
                        tunnel: [w555 w560] -> w545
                        tunnel: w528 -> [_ w559]
                        frame "V50" {
                          n309 = case shown="True" w556 {
                            tunnel: ["" ("Empty String Constant") "*"] -> w555
                            frame False {
                            }
                            frame True {
                            }
                          }
                        }
                        frame Default {
                          n310 = Format Into String(w559) -> (resulting string=w560:string)  [unwired: 3 in, 1 out]
                        }
                      }
                      n311 = case shown="1" w536 {
                        tunnel: ["P" "C"] -> w535
                        frame 0, Default {
                        }
                        frame 1 {
                        }
                      }
                      n312 = Format Into String(format string="%2d", w553) -> (resulting string=w538:string)  [unwired: 2 in, 1 out]
                      n313 = Format Into String(w552) -> (resulting string=w539:string)  [unwired: 3 in, 1 out]
                      n314 = Format Into String(w551) -> (resulting string=w540:string)  [unwired: 3 in, 1 out]
                      n315 = Format Into String(w550) -> (resulting string=w541:string)  [unwired: 3 in, 1 out]
                      n316 = Format Into String(w549) -> (resulting string=w542:string)  [unwired: 3 in, 1 out]
                      n317 = Format Into String(w548) -> (resulting string=w543:string)  [unwired: 3 in, 1 out]
                      n318 = Format Into String(w547) -> (resulting string=w544:string)  [unwired: 3 in, 1 out]
                      n319 = Format Into String(w529) -> (resulting string=w537:string)  [unwired: 3 in, 1 out]
                      n320 = Build Array(w538, w539, w540, w541, w542, w543, w544, w535, w545, w537) -> (w532:string[])
                      n321 = Array To Cluster(array=w532) -> (cluster=w534:T29)
                      n322 = Build Array (concatenate)(w533, w534) -> (w531:T17)
                    }
                    n323 = Array Size(array=w518) -> (size(s)=w520:i32)
                    n324 = Equal To 0?(x=w520) -> (x = 0?=w516:bool)
                    n325 = case shown="True" w516 {
                      tunnel: [w523 T17 [{"[0]"="", "[1]"="", "[2]"="", "[3]"="", "[4]"="", "[5]"="", "[6]"="", "[7]"="", "[8]"="", "[9]"=""}]] -> w517
                      tunnel: w518 -> [w523 _]
                      frame False {
                      }
                      frame True {
                      }
                    }
                    n326 = Sort 1D Array(array=w517) -> (sorted array=w519:T17)
                    n327 = for {
                      tunnel: w519 -> [w526] mode=indexing
                      tunnel: [w525] -> w522 mode=indexing
                      n328 = Cluster To Array(cluster=w526) -> (array=w525:string[])
                    }
                  }
                  frame "SPR0" {
                    # "SHOT TABLE"
                    n329 = control-ref of="Methods"() -> (w564:refnum<vi>)
                    n330 = call "Dropdown Selection (SubVI).vi"("reference"=w564) -> ("element"=w563:string)
                    n331 = for {
                      tunnel: w565 -> [w602] mode=indexing
                      shift-right: [w583] -> _
                      shift-left: T18 [] -> [w585]
                      tunnel: [w583] -> w568
                      tunnel: w563 -> [w579]
                      n332 = Unbundle By Name(w602) -> ("shot order"=w601:i32, "Powder Loading"=w600:sgl, "Uncorrected Impact"=w599:sgl, "UncorrectedRed_PB"=w598:sgl, "strikeVel_PB"=w597:sgl, "SHOT STATUS"=w588:u16, "usedv50"=w596:bool, "Shot Angle"=w580:u16, "BackFace\nDepth"=w581:sgl, "V50userExcl"=w578:bool, "Shot Description"=w577:string)
                      n333 = case shown="\"V50\"" w579 {
                        tunnel: w596 -> [w605 _]
                        tunnel: [w604 w612] -> w595
                        tunnel: w580 -> [_ w611]
                        tunnel: w578 -> [w603 _]
                        frame "V50" {
                          n334 = case shown="True" w603 {
                            tunnel: w605 -> [w607 _]
                            tunnel: [w606 "!"] -> w604
                            frame False {
                              n335 = case shown="False" w607 {
                                tunnel: ["" ("Empty String Constant") "*"] -> w606
                                frame False {
                                }
                                frame True {
                                }
                              }
                            }
                            frame True {
                            }
                          }
                        }
                        frame Default {
                          n336 = Format Into String(w611) -> (resulting string=w612:string)  [unwired: 3 in, 1 out]
                        }
                      }
                      n337 = case shown="1" w588 {
                        tunnel: ["P" "C"] -> w587
                        frame 0, Default {
                        }
                        frame 1 {
                        }
                      }
                      n338 = Format Into String(format string="%2d", w601) -> (resulting string=w590:string)  [unwired: 2 in, 1 out]
                      n339 = Format Into String(w600) -> (resulting string=w591:string)  [unwired: 3 in, 1 out]
                      n340 = Format Into String(w599) -> (resulting string=w592:string)  [unwired: 3 in, 1 out]
                      n341 = Format Into String(w598) -> (resulting string=w593:string)  [unwired: 3 in, 1 out]
                      n342 = Format Into String(w597) -> (resulting string=w594:string)  [unwired: 3 in, 1 out]
                      n343 = Format Into String(w581) -> (resulting string=w589:string)  [unwired: 3 in, 1 out]
                      n344 = Build Array(w590, w591, w592, w593, w594, w587, w595, w589, w577) -> (w584:string[])
                      n345 = Array To Cluster(array=w584) -> (cluster=w586:T30)
                      n346 = Build Array (concatenate)(w585, w586) -> (w583:T18)
                    }
                    n347 = Array Size(array=w568) -> (size(s)=w570:i32)
                    n348 = Equal To 0?(x=w570) -> (x = 0?=w566:bool)
                    n349 = case shown="True" w566 {
                      tunnel: [w573 T18 [{"[0]"="", "[1]"="", "[2]"="", "[3]"="", "[4]"="", "[5]"="", "[6]"="", "[7]"="", "[8]"=""}]] -> w567
                      tunnel: w568 -> [w573 _]
                      frame False {
                      }
                      frame True {
                      }
                    }
                    n350 = Sort 1D Array(array=w567) -> (sorted array=w569:T18)
                    n351 = for {
                      tunnel: w569 -> [w576] mode=indexing
                      tunnel: [w575] -> w572 mode=indexing
                      n352 = Cluster To Array(cluster=w576) -> (array=w575:string[])
                    }
                  }
                  frame "SPR1" {
                    # "SHOT TABLE"
                    n353 = control-ref of="Methods"() -> (w616:refnum<vi>)
                    n354 = call "Dropdown Selection (SubVI).vi"("reference"=w616) -> ("element"=w615:string)
                    n355 = for {
                      tunnel: w617 -> [w654] mode=indexing
                      shift-right: [w635] -> _
                      shift-left: T18 [] -> [w637]
                      tunnel: [w635] -> w620
                      tunnel: w615 -> [w631]
                      n356 = Unbundle By Name(w654) -> ("shot order"=w653:i32, "Powder Loading"=w652:sgl, "Uncorrected Impact"=w651:sgl, "UncorrectedRed_PB"=w650:sgl, "strikeVel_PB"=w649:sgl, "SHOT STATUS"=w640:u16, "usedv50"=w648:bool, "Shot Angle"=w632:u16, "BackFace\nDepth"=w633:sgl, "V50userExcl"=w630:bool, "Shot Description"=w629:string)
                      n357 = case shown="\"V50\"" w631 {
                        tunnel: w648 -> [w657 _]
                        tunnel: [w656 w664] -> w647
                        tunnel: w632 -> [_ w663]
                        tunnel: w630 -> [w655 _]
                        frame "V50" {
                          n358 = case shown="True" w655 {
                            tunnel: w657 -> [w659 _]
                            tunnel: [w658 "!"] -> w656
                            frame False {
                              n359 = case shown="False" w659 {
                                tunnel: ["" ("Empty String Constant") "*"] -> w658
                                frame False {
                                }
                                frame True {
                                }
                              }
                            }
                            frame True {
                            }
                          }
                        }
                        frame Default {
                          n360 = Format Into String(w663) -> (resulting string=w664:string)  [unwired: 3 in, 1 out]
                        }
                      }
                      n361 = case shown="1" w640 {
                        tunnel: ["P" "C"] -> w639
                        frame 0, Default {
                        }
                        frame 1 {
                        }
                      }
                      n362 = Format Into String(format string="%2d", w653) -> (resulting string=w642:string)  [unwired: 2 in, 1 out]
                      n363 = Format Into String(w652) -> (resulting string=w643:string)  [unwired: 3 in, 1 out]
                      n364 = Format Into String(w651) -> (resulting string=w644:string)  [unwired: 3 in, 1 out]
                      n365 = Format Into String(w650) -> (resulting string=w645:string)  [unwired: 3 in, 1 out]
                      n366 = Format Into String(w649) -> (resulting string=w646:string)  [unwired: 3 in, 1 out]
                      n367 = Format Into String(w633) -> (resulting string=w641:string)  [unwired: 3 in, 1 out]
                      n368 = Build Array(w642, w643, w644, w645, w646, w639, w647, w641, w629) -> (w636:string[])
                      n369 = Array To Cluster(array=w636) -> (cluster=w638:T30)
                      n370 = Build Array (concatenate)(w637, w638) -> (w635:T18)
                    }
                    n371 = Array Size(array=w620) -> (size(s)=w622:i32)
                    n372 = Equal To 0?(x=w622) -> (x = 0?=w618:bool)
                    n373 = case shown="True" w618 {
                      tunnel: [w625 T18 [{"[0]"="", "[1]"="", "[2]"="", "[3]"="", "[4]"="", "[5]"="", "[6]"="", "[7]"="", "[8]"=""}]] -> w619
                      tunnel: w620 -> [w625 _]
                      frame False {
                      }
                      frame True {
                      }
                    }
                    n374 = Sort 1D Array(array=w619) -> (sorted array=w621:T18)
                    n375 = for {
                      tunnel: w621 -> [w628] mode=indexing
                      tunnel: [w627] -> w624 mode=indexing
                      n376 = Cluster To Array(cluster=w628) -> (array=w627:string[])
                    }
                  }
                }
              }
              frame #5 {
                n377 = local read "Site"() -> (w667:string)
                n378 = case shown="\"ICE1\", Default" w667 {
                  tunnel: [w698 w719 w739] -> w674
                  tunnel: [w697 w718 w738] -> w673
                  tunnel: [w696 w717 w737] -> w672
                  tunnel: [w695 w702 w722] -> w671
                  tunnel: ["" ("projNum") w702 w722] -> w670
                  tunnel: [w693 w716 w736] -> w669
                  tunnel: [w677 w705 w725] -> w668
                  frame "ICE1", Default {
                    # "THREAT"
                    # "Range # (supports a PB reporting requirement)"
                    # "Project Name goes here.\nSupports a PB reporting requirement."
                    # "GENERAL"
                    n379 = local read "threatDetails"() -> (w676:T1)
                    n380 = Unbundle By Name(w676) -> ("barrelLength"=w680:string)
                    n381 = Unbundle By Name(w676) -> ("grainSize"=w675:string)
                    n382 = local read "Shot Angle"() -> (w681:u16)
                    n383 = control-ref of="WeaponTypes"() -> (w690:refnum<vi>)
                    n384 = control-ref of="ThreatGroups"() -> (w689:refnum<vi>)
                    n385 = control-ref of="PowderTypes"() -> (w688:refnum<vi>)
                    n386 = control-ref of="Recorders"() -> (w691:refnum<vi>)
                    n387 = control-ref of="Shooters"() -> (w692:refnum<vi>)
                    n388 = Format Into String(w681) -> (resulting string=w682:string)  [unwired: 3 in, 1 out]
                    n389 = call "Dropdown Selection (SubVI).vi"("reference"=w690) -> ("element"=w686:string)
                    n390 = call "Dropdown Selection (SubVI).vi"("reference"=w689) -> ("element"=w685:string)
                    n391 = call "Dropdown Selection (SubVI).vi"("reference"=w688) -> ("element"=w684:string)
                    n392 = call "Dropdown Selection (SubVI).vi"("reference"=w691) -> ("element"=w683:string)
                    n393 = call "Dropdown Selection (SubVI).vi"("reference"=w692) -> ("element"=w679:string)
                    n394 = local read "Comments"() -> (w696:string)
                    n395 = local read "ProjectID"() -> (w693:string)
                    n396 = local read "LastSample"() -> (w701:i32)
                    n397 = Bundle("element"=w686, "element"=w685, "grainSize"=w675, "element"=w684, "barrelLength"=w680, w682, "element"="1", "element"=w679, "element"=w683) -> (w687:T31)  [unwired: 1 out]
                    n398 = control-ref of="TestStandards"() -> (w700:refnum<vi>)
                    n399 = control-ref of="Methods"() -> (w699:refnum<vi>)
                    n400 = Cluster To Array(cluster=w687) -> (array=w677:string[])
                    n401 = call "Dropdown Selection (SubVI).vi"("reference"=w700) -> ("element"=w695:string)
                    n402 = call "Dropdown Selection (SubVI).vi"("reference"=w699) -> ("element"=w698:string)
                    n403 = Increment(x=w701) -> (x+1=w697:i32)
                  }
                  frame "SPR0" {
                    w702 = "" ("projNum")
                    # "THREAT"
                    # "Project Name goes here.\nSupports a PB reporting requirement."
                    # "GENERAL"
                    n404 = local read "threatDetails"() -> (w704:T1)
                    n405 = Unbundle By Name(w704) -> ("barrelLength"=w707:string)
                    n406 = Unbundle By Name(w704) -> ("grainSize"=w703:string)
                    n407 = local read "Shot Angle"() -> (w708:u16)
                    n408 = control-ref of="ThreatGroups"() -> (w714:refnum<vi>)
                    n409 = control-ref of="PowderTypes"() -> (w713:refnum<vi>)
                    n410 = control-ref of="Ballisticians"() -> (w715:refnum<vi>)
                    n411 = Format Into String(w708) -> (resulting string=w709:string)  [unwired: 3 in, 1 out]
                    n412 = call "Dropdown Selection (SubVI).vi"("reference"=w714) -> ("element"=w711:string)
                    n413 = call "Dropdown Selection (SubVI).vi"("reference"=w713) -> ("element"=w710:string)
                    n414 = call "Dropdown Selection (SubVI).vi"("reference"=w715) -> ("element"=w706:string)
                    n415 = local read "Comments"() -> (w717:string)
                    n416 = local read "ProjectID"() -> (w716:string)
                    n417 = local read "LastSample"() -> (w721:i32)
                    n418 = Bundle("element"=w711, "grainSize"=w703, "element"=w710, "barrelLength"=w707, w709, "element"=w706) -> (w712:T32)  [unwired: 1 out]
                    n419 = control-ref of="Methods"() -> (w720:refnum<vi>)
                    n420 = Cluster To Array(cluster=w712) -> (array=w705:string[])
                    n421 = call "Dropdown Selection (SubVI).vi"("reference"=w720) -> ("element"=w719:string)
                    n422 = Increment(x=w721) -> (x+1=w718:i32)
                  }
                  frame "SPR1" {
                    w722 = "" ("projNum")
                    # "THREAT"
                    # "Project Name goes here.\nSupports a PB reporting requirement."
                    # "GENERAL"
                    n423 = local read "threatDetails"() -> (w724:T1)
                    n424 = Unbundle By Name(w724) -> ("barrelLength"=w727:string)
                    n425 = Unbundle By Name(w724) -> ("grainSize"=w723:string)
                    n426 = local read "Shot Angle"() -> (w728:u16)
                    n427 = control-ref of="Ballisticians"() -> (w735:refnum<vi>)
                    n428 = control-ref of="ThreatGroups"() -> (w734:refnum<vi>)
                    n429 = control-ref of="PowderTypes"() -> (w733:refnum<vi>)
                    n430 = call "Dropdown Selection (SubVI).vi"("reference"=w735) -> ("element"=w726:string)
                    n431 = call "Dropdown Selection (SubVI).vi"("reference"=w734) -> ("element"=w731:string)
                    n432 = call "Dropdown Selection (SubVI).vi"("reference"=w733) -> ("element"=w730:string)
                    n433 = Format Into String(w728) -> (resulting string=w729:string)  [unwired: 3 in, 1 out]
                    n434 = control-ref of="Methods"() -> (w740:refnum<vi>)
                    n435 = local read "LastSample"() -> (w741:i32)
                    n436 = local read "Comments"() -> (w737:string)
                    n437 = local read "ProjectID"() -> (w736:string)
                    n438 = Bundle("element"=w731, "grainSize"=w723, "element"=w730, "barrelLength"=w727, w729, "element"=w726) -> (w732:T32)  [unwired: 1 out]
                    n439 = call "Dropdown Selection (SubVI).vi"("reference"=w740) -> ("element"=w739:string)
                    n440 = Cluster To Array(cluster=w732) -> (array=w725:string[])
                    n441 = Increment(x=w741) -> (x+1=w738:i32)
                  }
                }
              }
            }
            n442 = Get Date/Time String() -> (date string=w324:string)  [unwired: 3 in, 1 out]
          }
          frame True {
            w757 = ""
            w749 = 16  # dimensions
            w752 = 5  # SampleID
            # "date"
            # "method"
            # "general"
            # "remark"
            # "threat"
            # "shots"
            # "sample"
            # "results"
            # "range"
            # "fabric"
            # "query db with the entered record number and use result to populate the xlt"
            n443 = Not(x=w815) -> (.not. x?=w814:bool)
            n444 = local write "lookupRec"(w814) -> ()
            n445 = Format Into String(format string="SELECT * FROM Experiments\nWHERE expt=%d;" ("query string"), error in=w781, "Record #") -> (resulting string=w811:string, error out=w782:errorcluster)  [unwired: 1 in]
            n446 = call "Fetch Data (SubVI).vi"("error IN"=w782, "query string"=w811) -> ("error OUT"=w780:errorcluster, "recordset data"=w813:string[][])  [unwired: 4 out]
            n447 = Index Array(array=w813) -> (element=w751:string[])  [unwired: 2 in]
            n448 = Index Array(array=w751, index=111) -> (element=w784:string)
            n449 = local read "Set#1 Separation"() -> (w798:sgl)
            n450 = call "Load Shots (SubVI).vi"("Record #"="Record #", "Method"=w784) -> ("Shot Array"=w806:string[][], "AvgDef"=w789:dbl)  [unwired: 1 in]
            n451 = local read "mid_to_targ_dist"() -> (w801:sgl)
            n452 = local read "Barrel to Screen"() -> (w804:sgl)
            n453 = Format Into String(w789) -> (resulting string=w787:string)  [unwired: 3 in, 1 out]
            n454 = Match Pattern(string=w784, regular expression="N.I.J.") -> (offset past match=w786:i32)  [unwired: 4 out]
            n455 = Greater Or Equal To 0?(x=w786) -> (x >= 0?=w783:bool)
            n456 = case shown="False" w783 {
              tunnel: [w826 w827] -> w788
              tunnel: w787 -> [w823 w829]
              tunnel: w751 -> [w825 _]
              frame False {
                n457 = Index Array(array=w825, index #1=124 ("index"), index #2=149 ("index"), index #5=145 ("index")) -> (element #1=w824:string, element #2=w822:string, element #3=w821:string, element #4=w817:string, element #5=w818:string)  [unwired: 2 in]
                n458 = Build Array(w824, w822, w821, w817, w818, w823) -> (w826:string[])
              }
              frame True {
                w828 = "" ("Empty String Constant")
                n459 = Build Array(w828, w828, w828, w828, w828, w829, w829) -> (w827:string[])
              }
            }
            n460 = Divide(x=w798, y=sgl 2.0) -> (x/y=w803:sgl)
            n461 = Add(x=w804, y=w801) -> (x+y=w797:sgl)
            n462 = Subtract(x=w804, y=w803) -> (x-y=w802:sgl)
            n463 = Subtract(x=w801, y=w803) -> (x-y=w800:sgl)
            n464 = Index Array(array=w751, index #1=120 ("index"), index #2=119 ("index"), index #3=127 ("index"), index #4=12 ("index"), index #5=7 ("index")) -> (element #1=w769:string, element #2=w767:string, element #3=w766:string, element #4=w763:string, element #5=w762:string)
            n465 = Index Array(array=w751, index #1=113 ("index"), index #2=112 ("index"), index #3=103 ("index")) -> (element #1=w778:string, element #2=w777:string, element #3=w776:string, element #4=w775:string, element #5=w771:string)  [unwired: 2 in]
            n466 = Format Into String(w797) -> (resulting string=w796:string)  [unwired: 3 in, 1 out]
            n467 = Format Into String(w802) -> (resulting string=w795:string)  [unwired: 3 in, 1 out]
            n468 = Format Into String(w798) -> (resulting string=w794:string)  [unwired: 3 in, 1 out]
            n469 = Format Into String(w800) -> (resulting string=w793:string)  [unwired: 3 in, 1 out]
            n470 = Format Into String(w801) -> (resulting string=w792:string)  [unwired: 3 in, 1 out]
            n471 = Index Array(array=w751, index #1=w752, index #2=w749, index #3=147 ("index"), index #5=148 ("index")) -> (element #1=w750:string, element #2=w747:string, element #3=w746:string, element #5=w743:string)  [unwired: 1 in, 1 out]
            n472 = Build Array(w769, w767, w766, "", w763, w762) -> (w768:string[])
            n473 = Build Array(w796, w795, w794, w793, w792, w778, w777, w776, w775, w771) -> (w791:string[])
            n474 = Index Array(array=w751, index #1=4 ("index"), index #2=111 ("index")) -> (element #1=w758:string, element #2=w755:string)
            n475 = Index Array(array=w751, index=107) -> (element=w807:string)
            n476 = Build Array(w750, w747, w746, "", w743) -> (w748:string[])
            n477 = Index Array(array=w751, index=2) -> (element=w753:string)
            n478 = call "Get Model Construction.vi"("panel record"=w751) -> ("Fabric Array"=w805:string[][])
            n479 = Build Array(w788) -> (w808:string[][])
          }
        }
        n480 = To Variant(anything=w319) -> (Variant=w313:variant)
        n481 = To Variant(anything=w318) -> (Variant=w312:variant)
        n482 = To Variant(anything=w317) -> (Variant=w311:variant)
        n483 = To Variant(anything=w316) -> (Variant=w310:variant)
        n484 = To Variant(anything=w315) -> (Variant=w309:variant)
        n485 = To Variant(anything=w314) -> (Variant=w308:variant)
        n486 = To Variant(anything=w301) -> (Variant=w307:variant)
        n487 = To Variant(anything=w300) -> (Variant=w306:variant)
        n488 = To Variant(anything=w299) -> (Variant=w305:variant)
        n489 = To Variant(anything=w298) -> (Variant=w302:variant)
        n490 = To Variant(anything=w297) -> (Variant=w303:variant)
        n491 = To Variant(anything=w290) -> (Variant=w304:variant)
        n492 = To Variant(anything=w288) -> (Variant=w289:variant)
        n493 = call "TestReport_XL.vi"("Enable"=TRUE, "blockFabric"=w313, "blockRange"=w312, "blockResults"=w311, "blockSample"=w310, "blockShotTbl"=w309, "error in (no error)"=w293, "blockThreat"=w308, "testDate"=w289, "method"=w307, "projName"=w306, "projNum"=w305, "recNum"=w302, "remark"=w303, "standard"=w304) -> ("error out"=w320:errorcluster)  [unwired: 4 in, 8 out]
        n494 = call <vilib>:"Simple Error Handler.vi"("error in (no error)"=w320) -> ("error out"=w322:errorcluster)  [unwired: 1 in, 7 out]
        n495 = case shown="No Error" w322 {
          selector: w322 -> [w830 w832]
          tunnel: [w830 w832] -> w291
          frame No Error {
            n496 = One Button Dialog(message=" V50 Ballistic Test Report is ready") -> ()  [unwired: 2 out]
          }
          frame Error {
          }
        }
      }
      frame 3 {
        w862 = TRUE  # Enable
        # "The custom Excel template file is \nexpected in the C:\\Ballistics folder."
        n497 = stacked-sequence {
          tunnel: [_ _ _ _ _ w1053] -> w855
          tunnel: [_ w926 _ _ _ _] -> w859
          tunnel: [_ _ _ _ w1010 _] -> w856
          tunnel: [_ _ _ w977 _ _] -> w857
          tunnel: [_ _ w948 _ _ _] -> w858
          tunnel: [w870 _ _ _ _ _] -> w860
          tunnel: [_ _ _ _ _ w1074] -> w842
          tunnel: [_ _ _ _ _ "" ("projNum")] -> w841
          tunnel: [_ _ _ _ _ w1069] -> w840
          tunnel: [_ _ _ _ _ w1073] -> w839
          tunnel: [_ _ _ _ _ w1072] -> w838
          tunnel: [_ _ _ _ _ w1071] -> w837
          tunnel: w836 -> [_ _ w947 _ w1003 _]
          frame #0 {
            # "FABRIC"
            n498 = local read "fab1_totalWt"() -> (w873:sgl)
            n499 = local read "fab3_totalWt"() -> (w875:sgl)
            n500 = local read "fab5_totalWt"() -> (w877:sgl)
            n501 = global read "BIMS_Collector Globals.vi" "LayerStitchTypeRefs"() -> (w865:refnum<vi>[])
            n502 = global read "BIMS_Collector Globals.vi" "SampleAttribs"() -> (w866:T23)
            n503 = global read "BIMS_Collector Globals.vi" "SampleStyles"() -> (w868:refnum<vi>[])
            n504 = local read "fab2_totalWt"() -> (w874:sgl)
            n505 = local read "fab4_totalWt"() -> (w876:sgl)
            n506 = local read "fab6_totalWt"() -> (w878:sgl)
            n507 = global read "BIMS_Collector Globals.vi" "LayerSpecs"() -> (w867:T24)
            n508 = global read "BIMS_Collector Globals.vi" "Mfrs"() -> (w869:refnum<vi>[])
            n509 = Build Array(w873, w874, w875, w876, w877, w878) -> (w872:sgl[])
            n510 = for {
              tunnel: w872 -> [w880] mode=indexing
              tunnel: [w886] -> w871 mode=indexing
              tunnel: w866 -> [w884] mode=indexing
              tunnel: w867 -> [w883] mode=indexing
              tunnel: w869 -> [w882] mode=indexing
              tunnel: w868 -> [w881] mode=indexing
              tunnel: w865 -> [w879] mode=indexing
              n511 = Less Or Equal To 0?(x=w880) -> (x <= 0?=w885:bool)
              n512 = case shown="False" w885 {
                tunnel: [w908 w910] -> w886
                tunnel: w884 -> [w907 _]
                tunnel: w883 -> [w892 _]
                tunnel: w882 -> [w901 _]
                tunnel: w881 -> [w898 _]
                tunnel: w880 -> [w891 _]
                tunnel: w879 -> [w887 _]
                frame False {
                  n513 = Unbundle By Name(w892) -> ("numOfPlies"=w890:i32, "LotNum"=w904:string, "RollNum"=w905:string)
                  n514 = Unbundle By Name(w907) -> ("internal_ID"=w895:string, "fiber"=w896:string, "denier"=w903:string, "pick"=w902:string, "weave"=w893:string, "finish"=w894:string, "ozPerYd2"=w906:string)
                  n515 = Format Into String(w890) -> (resulting string=w900:string)  [unwired: 3 in, 1 out]
                  n516 = call "Dropdown Selection (SubVI).vi"("reference"=w901) -> ("element"=w899:string)
                  n517 = call "Dropdown Selection (SubVI).vi"("reference"=w898) -> ("element"=w897:string)
                  n518 = call "Dropdown Selection (SubVI).vi"("reference"=w887) -> ("element"=w888:string)
                  n519 = Format Into String(w891) -> (resulting string=w889:string)  [unwired: 3 in, 1 out]
                  n520 = Build Array(w900, w899, w897, w895, w896, w903, w902, w893, w894, w904, w905, w906, w889, w888) -> (w908:string[])
                }
                frame True {
                  n521 = call <vilib>:"Space Constant.vi"() -> ("String"=w911:string)
                  n522 = Initialize Array(w911, 12 ("dimension size")) -> (w910:string[])
                }
              }
            }
            n523 = Transpose 2D Array(2D array=w871) -> (transposed array=w870:string[][])
          }
          frame #1 {
            w912 = "%.1f" ("format string")
            # "muzzel / midpoint"
            # "muzzle / scr#1"
            # "muzzle / target"
            # "scr#2 / target"
            # "RANGE"
            n524 = local read "Set#1 Separation"() -> (w919:sgl)
            n525 = local read "mid_to_targ_dist"() -> (w916:sgl)
            n526 = local read "Barrel to Screen"() -> (w913:sgl)
            n527 = local read "clayAverage"() -> (w934:sgl)
            n528 = Divide(x=w919, y=sgl 2.0) -> (x/y=w914:sgl)
            n529 = local read "RoomHum"() -> (w929:sgl)
            n530 = local read "clayTemp"() -> (w932:sgl)
            n531 = local read "clayCalib"() -> (w935:string)
            n532 = local read "RoomT"() -> (w930:sgl)
            n533 = Add(x=w913, y=w916) -> (x+y=w920:sgl)
            n534 = Subtract(x=w913, y=w914) -> (x-y=w915:sgl)
            n535 = Subtract(x=w916, y=w914) -> (x-y=w917:sgl)
            n536 = Format Into String(w920) -> (resulting string=w921:string)  [unwired: 3 in, 1 out]
            n537 = Format Into String(w915) -> (resulting string=w922:string)  [unwired: 3 in, 1 out]
            n538 = Format Into String(w919) -> (resulting string=w923:string)  [unwired: 3 in, 1 out]
            n539 = Format Into String(w917) -> (resulting string=w924:string)  [unwired: 3 in, 1 out]
            n540 = Format Into String(w916) -> (resulting string=w925:string)  [unwired: 3 in, 1 out]
            n541 = Format Into String(w929) -> (resulting string=w927:string)  [unwired: 3 in, 1 out]
            n542 = Format Into String(format string=w912, w930) -> (resulting string=w928:string)  [unwired: 2 in, 1 out]
            n543 = Format Into String(format string=w912, w932) -> (resulting string=w931:string)  [unwired: 2 in, 1 out]
            n544 = Format Into String(format string=w912, w934) -> (resulting string=w933:string)  [unwired: 2 in, 1 out]
            n545 = Bundle(w921, w922, w923, w924, w925, w927, w928, w931, "clayCalib"=w935, w933) -> (w936:T25)  [unwired: 1 out]
            n546 = Cluster To Array(cluster=w936) -> (array=w926:string[])
          }
          frame #2 {
            # "RESULTS"
            n547 = control-ref of="Methods"() -> (w937:refnum<vi>)
            n548 = call "Dropdown Selection (SubVI).vi"("reference"=w937) -> ("element"=w938:string)
            n549 = for {
              tunnel: w947 -> [w975] mode=indexing
              tunnel: [w974] -> w946 mode=indexing
              tunnel: [w973] -> w945
              i -> [w973]
              n550 = Unbundle By Name(w975) -> ("BackFace\nDepth"=w974:sgl)
            }
            n551 = Increment(x=w945) -> (x+1=w943:i32)
            n552 = Add Array Elements(numeric array=w946) -> (sum=w944:sgl)
            n553 = To Single Precision Float(number=w943) -> (single precision float=w942:sgl)
            n554 = Divide(x=w944, y=w942) -> (x/y=w941:sgl)
            n555 = Format Into String(format string="%1.1f", w941) -> (resulting string=w940:string)  [unwired: 2 in, 1 out]
            n556 = case shown="\"V50\"" w938 {
              tunnel: [w963 w972] -> w950
              tunnel: w940 -> [w951 w971]
              frame "V50" {
                w957 = "%1d" ("format string")
                n557 = local read "Z.M.R."() -> (w955:sgl)
                n558 = Less Than 0?(x=w955) -> (x < 0?=w956:bool)
                n559 = local read "rangeOfResults"() -> (w959:i32)
                n560 = local read "computed_V50"() -> (w962:sgl)
                n561 = local read "lowComplete"() -> (w960:i32)
                n562 = local read "highPartial"() -> (w961:i32)
                n563 = case shown="True" w956 {
                  tunnel: w955 -> [w968 _]
                  tunnel: [w968 sgl 0.0 ("Z.M.R.")] -> w954
                  frame False {
                  }
                  frame True {
                  }
                }
                n564 = Format Into String(format string="%1.1f", w962) -> (resulting string=w966:string)  [unwired: 2 in, 1 out]
                n565 = Format Into String(format string=w957, w961) -> (resulting string=w965:string)  [unwired: 2 in, 1 out]
                n566 = Format Into String(format string=w957, w960) -> (resulting string=w964:string)  [unwired: 2 in, 1 out]
                n567 = Format Into String(format string=w957, w959) -> (resulting string=w967:string)  [unwired: 2 in, 1 out]
                n568 = Format Into String(format string="%1.1f", w954) -> (resulting string=w953:string)  [unwired: 2 in, 1 out]
                n569 = Bundle(w966, w965, w964, w967, w953, w951, w951) -> (w963:T26)  [unwired: 1 out]
              }
              frame Default {
                w970 = "" ("Empty String Constant")
                n570 = Bundle(w970, w970, w970, w970, w970, w971, w971) -> (w972:T26)  [unwired: 1 out]
              }
            }
            n571 = Cluster To Array(cluster=w950) -> (array=w949:string[])
            n572 = Build Array(w949) -> (w948:string[][])
          }
          frame #3 {
            # "PB Req"
            # "SAMPLE"
            n573 = control-ref of="Methods"() -> (w978:refnum<vi>)
            n574 = call "Dropdown Selection (SubVI).vi"("reference"=w978) -> ("element"=w980:string)
            n575 = Equal?(x=w980, y="V50") -> (x = y?=w979:bool)
            n576 = local read "totalSampleWt"() -> (w990:sgl)
            n577 = case shown="True" w979 {
              tunnel: ["n/a" w1000] -> w984
              frame False {
              }
              frame True {
                n578 = local read "minV50"() -> (w999:i32)
                n579 = Format Into String(w999) -> (resulting string=w1000:string)  [unwired: 3 in, 1 out]
              }
            }
            n580 = local read "Type of work"() -> (w976:string)
            n581 = control-ref of="SampleDimensions"() -> (w996:refnum<vi>)
            n582 = control-ref of="SampleCoverings"() -> (w997:refnum<vi>)
            n583 = control-ref of="Models"() -> (w983:refnum<vi>)
            n584 = local read "serialNum"() -> (w992:string)
            n585 = local read "SampleID"() -> (w994:string)
            n586 = local read "Thickness"() -> (w987:dbl)
            n587 = local read "totalBAW"() -> (w986:sgl)
            n588 = call "Dropdown Selection (SubVI).vi"("reference"=w996) -> ("element"=w993:string)
            n589 = call "Dropdown Selection (SubVI).vi"("reference"=w983) -> ("element"=w982:string)
            n590 = call "Dropdown Selection (SubVI).vi"("reference"=w997) -> ("element"=w991:string)
            n591 = Format Into String(w990) -> (resulting string=w989:string)  [unwired: 3 in, 1 out]
            n592 = Format Into String(w987) -> (resulting string=w988:string)  [unwired: 3 in, 1 out]
            n593 = Format Into String(w986) -> (resulting string=w985:string)  [unwired: 3 in, 1 out]
            n594 = Bundle("SampleID"=w994, "element"=w993, "Type of work"=w976, "serialNum"=w992, "element"=w982, w989, w988, w985, "element"=w991, w984) -> (w995:T27)  [unwired: 1 out]
            n595 = Cluster To Array(cluster=w995) -> (array=w977:string[])
          }
          frame #4 {
            # "SHOT TABLE"
            n596 = control-ref of="Methods"() -> (w1002:refnum<vi>)
            n597 = call "Dropdown Selection (SubVI).vi"("reference"=w1002) -> ("element"=w1001:string)
            n598 = for {
              tunnel: w1003 -> [w1042] mode=indexing
              shift-right: [w1019] -> _
              shift-left: T17 [] -> [w1021]
              tunnel: [w1019] -> w1006
              tunnel: w1001 -> [w1015]
              n599 = Unbundle By Name(w1042) -> ("shot order"=w1041:i32, "Powder Loading"=w1040:sgl, "Uncorrected Impact"=w1039:sgl, "UncorrectedRed_PB"=w1038:sgl, "UncorrectedAvgVel_PB"=w1037:sgl, "velLoss_PB"=w1036:sgl, "strikeVel_PB"=w1035:sgl, "SHOT STATUS"=w1024:u16, "usedv50"=w1034:bool, "Shot Angle"=w1016:u16, "BackFace\nDepth"=w1017:sgl)
              n600 = case shown="\"V50\"" w1015 {
                tunnel: w1034 -> [w1044 _]
                tunnel: [w1043 w1048] -> w1033
                tunnel: w1016 -> [_ w1047]
                frame "V50" {
                  n601 = case shown="True" w1044 {
                    tunnel: ["" ("Empty String Constant") "*"] -> w1043
                    frame False {
                    }
                    frame True {
                    }
                  }
                }
                frame Default {
                  n602 = Format Into String(w1047) -> (resulting string=w1048:string)  [unwired: 3 in, 1 out]
                }
              }
              n603 = case shown="1" w1024 {
                tunnel: ["P" "C"] -> w1023
                frame 0, Default {
                }
                frame 1 {
                }
              }
              n604 = Format Into String(format string="%2d", w1041) -> (resulting string=w1026:string)  [unwired: 2 in, 1 out]
              n605 = Format Into String(w1040) -> (resulting string=w1027:string)  [unwired: 3 in, 1 out]
              n606 = Format Into String(w1039) -> (resulting string=w1028:string)  [unwired: 3 in, 1 out]
              n607 = Format Into String(w1038) -> (resulting string=w1029:string)  [unwired: 3 in, 1 out]
              n608 = Format Into String(w1037) -> (resulting string=w1030:string)  [unwired: 3 in, 1 out]
              n609 = Format Into String(w1036) -> (resulting string=w1031:string)  [unwired: 3 in, 1 out]
              n610 = Format Into String(w1035) -> (resulting string=w1032:string)  [unwired: 3 in, 1 out]
              n611 = Format Into String(w1017) -> (resulting string=w1025:string)  [unwired: 3 in, 1 out]
              n612 = Build Array(w1026, w1027, w1028, w1029, w1030, w1031, w1032, w1023, w1033, w1025) -> (w1020:string[])
              n613 = Array To Cluster(array=w1020) -> (cluster=w1022:T29)
              n614 = Build Array (concatenate)(w1021, w1022) -> (w1019:T17)
            }
            n615 = Array Size(array=w1006) -> (size(s)=w1008:i32)
            n616 = Equal To 0?(x=w1008) -> (x = 0?=w1004:bool)
            n617 = case shown="True" w1004 {
              tunnel: [w1011 T17 [{"[0]"="", "[1]"="", "[2]"="", "[3]"="", "[4]"="", "[5]"="", "[6]"="", "[7]"="", "[8]"="", "[9]"=""}]] -> w1005
              tunnel: w1006 -> [w1011 _]
              frame False {
              }
              frame True {
              }
            }
            n618 = Sort 1D Array(array=w1005) -> (sorted array=w1007:T17)
            n619 = for {
              tunnel: w1007 -> [w1014] mode=indexing
              tunnel: [w1013] -> w1010 mode=indexing
              n620 = Cluster To Array(cluster=w1014) -> (array=w1013:string[])
            }
          }
          frame #5 {
            # "THREAT"
            # "Range # (supports a PB reporting requirement)"
            # "Project Name goes here.\nSupports a PB reporting requirement."
            # "GENERAL"
            n621 = local read "threatDetails"() -> (w1052:T1)
            n622 = Unbundle By Name(w1052) -> ("barrelLength"=w1056:string)
            n623 = Unbundle By Name(w1052) -> ("grainSize"=w1051:string)
            n624 = local read "Shot Angle"() -> (w1057:u16)
            n625 = control-ref of="WeaponTypes"() -> (w1066:refnum<vi>)
            n626 = control-ref of="ThreatGroups"() -> (w1065:refnum<vi>)
            n627 = control-ref of="PowderTypes"() -> (w1064:refnum<vi>)
            n628 = control-ref of="Recorders"() -> (w1067:refnum<vi>)
            n629 = control-ref of="Shooters"() -> (w1068:refnum<vi>)
            n630 = Format Into String(w1057) -> (resulting string=w1058:string)  [unwired: 3 in, 1 out]
            n631 = call "Dropdown Selection (SubVI).vi"("reference"=w1066) -> ("element"=w1062:string)
            n632 = call "Dropdown Selection (SubVI).vi"("reference"=w1065) -> ("element"=w1061:string)
            n633 = call "Dropdown Selection (SubVI).vi"("reference"=w1064) -> ("element"=w1060:string)
            n634 = call "Dropdown Selection (SubVI).vi"("reference"=w1067) -> ("element"=w1059:string)
            n635 = call "Dropdown Selection (SubVI).vi"("reference"=w1068) -> ("element"=w1055:string)
            n636 = Bundle("element"=w1062, "element"=w1061, "grainSize"=w1051, "element"=w1060, "barrelLength"=w1056, w1058, "element"="1", "element"=w1055, "element"=w1059) -> (w1063:T31)  [unwired: 1 out]
            n637 = Cluster To Array(cluster=w1063) -> (array=w1053:string[])
            n638 = local read "Comments"() -> (w1072:string)
            n639 = local read "ProjectID"() -> (w1069:string)
            n640 = local read "LastSample"() -> (w1077:i32)
            n641 = control-ref of="TestStandards"() -> (w1076:refnum<vi>)
            n642 = control-ref of="Methods"() -> (w1075:refnum<vi>)
            n643 = call "Dropdown Selection (SubVI).vi"("reference"=w1076) -> ("element"=w1071:string)
            n644 = call "Dropdown Selection (SubVI).vi"("reference"=w1075) -> ("element"=w1074:string)
            n645 = Increment(x=w1077) -> (x+1=w1073:i32)
          }
        }
        n646 = To Variant(anything=w860) -> (Variant=w854:variant)
        n647 = To Variant(anything=w859) -> (Variant=w853:variant)
        n648 = To Variant(anything=w858) -> (Variant=w852:variant)
        n649 = To Variant(anything=w857) -> (Variant=w851:variant)
        n650 = To Variant(anything=w856) -> (Variant=w850:variant)
        n651 = To Variant(anything=w855) -> (Variant=w849:variant)
        n652 = To Variant(anything=w842) -> (Variant=w848:variant)
        n653 = To Variant(anything=w841) -> (Variant=w847:variant)
        n654 = To Variant(anything=w840) -> (Variant=w846:variant)
        n655 = To Variant(anything=w839) -> (Variant=w843:variant)
        n656 = To Variant(anything=w838) -> (Variant=w844:variant)
        n657 = To Variant(anything=w837) -> (Variant=w845:variant)
        n658 = call "TestReport_XL.vi"("Enable"=w862, "blockFabric"=w854, "blockRange"=w853, "blockResults"=w852, "blockSample"=w851, "blockShotTbl"=w850, "error in (no error)"=w834, "blockThreat"=w849, "method"=w848, "projName"=w847, "projNum"=w846, "recNum"=w843, "remark"=w844, "standard"=w845) -> ("error out"=w861:errorcluster)  [unwired: 5 in, 8 out]
        n659 = call <vilib>:"Simple Error Handler.vi"("error in (no error)"=w861) -> ("error out"=w863:errorcluster)  [unwired: 1 in, 7 out]
        n660 = case shown="No Error" w863 {
          selector: w863 -> [w1078 w1080]
          tunnel: [w1078 w1080] -> w833
          frame No Error {
            n661 = One Button Dialog(message=" VsVr Ballistic Test Report is ready") -> ()  [unwired: 2 out]
          }
          frame Error {
          }
        }
      }
      frame 4 {
        # "This section saves the shots to the data base"
        n662 = stacked-sequence {
          seq-local: [w1146 _ _] -> [_ w1232 _]
          seq-local: [w1148 _ _] -> [_ w1229 _]
          seq-local: [_ w1217 _] -> [_ _ w1246]
          seq-local: [_ w1219 _] -> [_ _ w1245]
          seq-local: [w1144 _ _] -> [_ _ w1238]
          seq-local: [w1118 _ _] -> [_ w1175 _]
          tunnel: [_ _ w1240] -> w1086
          tunnel: [_ _ w1243] -> w1087
          tunnel: w1082 -> [_ w1184 w1237]
          tunnel: w1084 -> [w1120 _ _]
          tunnel: ["SampleDescrip" _ _] -> _
          tunnel: ["Areal Density" _ _] -> _
          tunnel: ["Areal density text" _ _] -> _
          tunnel: ["SoftwareVersion" _ _] -> _
          tunnel: ["Fabric Description" _ _] -> _
          tunnel: ["Threat" _ _] -> _
          tunnel: ["old threat" _ _] -> _
          tunnel: ["line direction map" _ _] -> _
          tunnel: ["Methods" _ _] -> _
          tunnel: ["SampleCoverings" _ _] -> _
          tunnel: ["Ballisticians" _ _] -> _
          tunnel: ["Submitters" _ _] -> _
          tunnel: ["SampleDimensions" _ _] -> _
          tunnel: ["PowderTypes" _ _] -> _
          tunnel: ["SampleTypes" _ _] -> _
          tunnel: ["TestConditions" _ _] -> _
          tunnel: ["ModelMfrs" _ _] -> _
          tunnel: ["Assemblers" _ _] -> _
          tunnel: ["N.I.J" _ _] -> _
          tunnel: ["SampleClamping" _ _] -> _
          tunnel: ["FrontLayer" _ _] -> _
          tunnel: ["BackLayer" _ _] -> _
          frame #0 {
            # "Legacy requirements:"
            # "Shared requirements:"
            n663 = local read "fab1_totalWt"() -> (w1156:sgl)
            n664 = local read "fab2_totalWt"() -> (w1155:sgl)
            n665 = local read "fab3_totalWt"() -> (w1154:sgl)
            n666 = local read "fab4_totalWt"() -> (w1153:sgl)
            n667 = local read "fab5_totalWt"() -> (w1152:sgl)
            n668 = local read "fab6_totalWt"() -> (w1151:sgl)
            n669 = flat-sequence {
              tunnel: ["TestStandards"] -> _
              tunnel: ["Shooters"] -> _
              tunnel: ["Recorders"] -> _
              tunnel: ["WeaponTypes"] -> _
              tunnel: ["Models"] -> _
              tunnel: ["serialNum"] -> _
              tunnel: ["layerStitch_1"] -> _
              tunnel: ["layerStitch_2"] -> _
              tunnel: ["layerStitch_3"] -> _
              tunnel: ["layerStitch_4"] -> _
              tunnel: ["layerStitch_5"] -> _
              tunnel: ["layerStitch_6"] -> _
              tunnel: ["minV50"] -> _
              frame #0 {
                # "PB-only requirements:"
              }
            }
            n670 = Build Array(w1156, w1155, w1154, w1153, w1152, w1151) -> (w1150:sgl[])
            n671 = call "SQL Statement for Sample Descritpion.vi"("error IN"=w1120, "Layer Weight Array"=w1150, "VALUES clause IN"=" VALUES (%d " ("SQL statement IN"), "INSERT clause IN"="INSERT INTO Experiments " ("SQL statement IN")) -> ("error OUT"=w1119:errorcluster, "VALUES clause OUT"=w1149:string, "INSERT clause OUT"=w1147:string)  [unwired: 1 out]
            n672 = local read "LastSample"() -> (w1145:i32)
            n673 = Increment(x=w1145) -> (x+1=w1144:i32)
            n674 = local read "rangeOfResults"() -> (w1122:i32)
            n675 = local read "lowComplete"() -> (w1123:i32)
            n676 = local read "clayAverage"() -> (w1125:sgl)
            n677 = local read "highPartial"() -> (w1124:i32)
            n678 = control-ref of="SampleClamping"() -> (w1117:refnum<vi>)
            n679 = control-ref of="BackLayer"() -> (w1093:refnum<vi>)
            n680 = control-ref of="FrontLayer"() -> (w1092:refnum<vi>)
            n681 = control-ref of="Ballisticians"() -> (w1139:refnum<vi>)
            n682 = control-ref of="Shooters"() -> (w1135:refnum<vi>)
            n683 = control-ref of="Recorders"() -> (w1134:refnum<vi>)
            n684 = control-ref of="Submitters"() -> (w1138:refnum<vi>)
            n685 = control-ref of="SampleCoverings"() -> (w1131:refnum<vi>)
            n686 = control-ref of="ThreatGroups"() -> (w1130:refnum<vi>)
            n687 = call "Dropdown Selection (SubVI).vi"("reference"=w1139) -> ("element"=w1137:string)
            n688 = call "Dropdown Selection (SubVI).vi"("reference"=w1135) -> ("element"=w1133:string)
            n689 = call "Dropdown Selection (SubVI).vi"("reference"=w1134) -> ("element"=w1132:string)
            n690 = call "Dropdown Selection (SubVI).vi"("reference"=w1138) -> ("element"=w1136:string)
            n691 = call "Dropdown Selection (SubVI).vi"("reference"=w1131) -> ("element"=w1129:string)
            n692 = call "Dropdown Selection (SubVI).vi"("reference"=w1130) -> ("element"=w1128:string)
            n693 = call "Dropdown Selection (SubVI).vi"("reference"=w1117) -> ("element"=w1116:string)
            n694 = call "Dropdown Selection (SubVI).vi"("reference"=w1093) -> ("element"=w1091:string)
            n695 = call "Dropdown Selection (SubVI).vi"("reference"=w1092) -> ("element"=w1090:string)
            n696 = Concatenate Strings(w1147, ", expt, [date], Ballistician1, Ballistician2, Ballistician3, Submitter1, SampleCovering, ProjectileType, ClayTemp, ClayCalibration, ClayAvgThickness, highPartial, lowComplete, rangeOfResults, clamping, FrontPly, BackPly," ("Substring")) -> (w1146:string)
            n697 = Format Into String(format string=", %d, #%s#, '%s', '%s', '%s', '%s', '%s', '%s', %.1f, '%s', %.1f, %d, %d, %d, '%s', '%s', '%s'" ("Format String"), initial string=w1149, error in=w1119, w1144, "currentDateTime", w1137, w1133, w1132, w1136, w1129, w1128, "clayTemp", "clayCalib", w1125, w1124, w1123, w1122, w1116, w1091, w1090) -> (resulting string=w1148:string, error out=w1118:errorcluster)
          }
          frame #1 {
            w1231 = " Angle, Conditions, SampleType, ThreatGrain, ThreatDetail, V50dc, V50, maker, thickness, powder, numshots, backing, totalnumberplys, testcomments, NIJ1, method, temperature, humidity, Dimensions, zmr, ProjectID, SampleID, panelmaker, panelWeight, totalBAW)"  # INSERT clause continued
            # "Although shot angle is defined for the overall\nexperiment, it is also recorded for each shot."
            n698 = local read "computed_V50"() -> (w1227:sgl)
            n699 = local read "Drag Corrected"() -> (w1222:bool)
            n700 = local read "Impact factor"() -> (w1224:sgl)
            n701 = Array Size(array=w1184) -> (size(s)=w1215:i32)
            n702 = Select(t=w1224, s=w1222, f=sgl 1.0) -> (s? t:f=w1223:sgl)
            n703 = Divide(x=w1227, y=w1223) -> (x/y=w1226:sgl)
            n704 = control-ref of="ModelMfrs"() -> (w1210:refnum<vi>)
            n705 = control-ref of="PowderTypes"() -> (w1208:refnum<vi>)
            n706 = call "Dropdown Selection (SubVI).vi"("reference"=w1210) -> ("element"=w1209:string)
            n707 = call "Dropdown Selection (SubVI).vi"("reference"=w1208) -> ("element"=w1192:string)
            n708 = local read "GrainSize"() -> (w1173:u16)
            n709 = local read "Z.M.R."() -> (w1198:sgl)
            n710 = local read "Shot Angle"() -> (w1186:u16)
            n711 = Less Than 0?(x=w1198) -> (x < 0?=w1197:bool)
            n712 = local read "totalNumLayers"() -> (w1214:i32)
            n713 = control-ref of="ThreatDetails"() -> (w1170:refnum<vi>)
            n714 = control-ref of="SampleTypes"() -> (w1180:refnum<vi>)
            n715 = control-ref of="TestConditions"() -> (w1199:refnum<vi>)
            n716 = control-ref of="SampleBackings"() -> (w1207:refnum<vi>)
            n717 = Format Into String(w1173) -> (resulting string=w1172:string)  [unwired: 3 in, 1 out]
            n718 = local read "totalBAW"() -> (w1200:sgl)
            n719 = case shown="True" w1197 {
              tunnel: w1198 -> [w1235 _]
              tunnel: [w1235 sgl 0.0 ("Z.M.R.")] -> w1196
              frame False {
              }
              frame True {
              }
            }
            n720 = control-ref of="SampleDimensions"() -> (w1203:refnum<vi>)
            n721 = control-ref of="N.I.J"() -> (w1205:refnum<vi>)
            n722 = control-ref of="Methods"() -> (w1190:refnum<vi>)
            n723 = control-ref of="Assemblers"() -> (w1201:refnum<vi>)
            n724 = call "Dropdown Selection (SubVI).vi"("reference"=w1170) -> ("element"=w1171:string)
            n725 = call "Dropdown Selection (SubVI).vi"("reference"=w1180) -> ("element"=w1179:string)
            n726 = call "Dropdown Selection (SubVI).vi"("reference"=w1199) -> ("element"=w1185:string)
            n727 = call "Dropdown Selection (SubVI).vi"("reference"=w1207) -> ("element"=w1206:string)
            n728 = Equal?(x=w1172, y="") -> (x = y?=w1194:bool)
            n729 = call "Dropdown Selection (SubVI).vi"("reference"=w1205) -> ("element"=w1204:string)
            n730 = call "Dropdown Selection (SubVI).vi"("reference"=w1190) -> ("element"=w1189:string)
            n731 = call "Dropdown Selection (SubVI).vi"("reference"=w1203) -> ("element"=w1202:string)
            n732 = call "Dropdown Selection (SubVI).vi"("reference"=w1201) -> ("element"=w1191:string)
            n733 = case shown="False" w1194 {
              tunnel: [w1233 "0" ("element")] -> w1193
              tunnel: w1172 -> [w1233 _]
              frame False {
              }
              frame True {
              }
            }
            n734 = call "Prepare DB Connect Path (SubVI).vi"("connectString"=path "BIMS_Collector.udl", "error in"=w1175) -> ("appended path"=w1174:path, "error out"=w1176:errorcluster)  [unwired: 1 out]
            n735 = Format Into String(format string=", %d, '%s', '%s', '%s', '%s', %.4f, %.1f, '%s', %.4f, '%s', %d, '%s', %d, '%s', '%s', '%s', %.1f, %.1f, '%s', %.1f, '%s', '%s', '%s', %.1f, %.1f);" ("Format String"), initial string=w1229, error in=w1176, w1186, w1185, w1179, w1193, w1171, w1227, w1226, w1209, "Thickness", w1192, w1215, w1206, w1214, "Comments", w1204, w1189, "RoomT", "RoomHum", w1202, w1196, "ProjectID", "SampleID", w1191, "totalSampleWt", w1200) -> (resulting string=w1228:string, error out=w1178:errorcluster)
            n736 = call-poly <vilib>:"DB Tools Open Connection.vi"("error in (no error)"=w1178, "connection information"=w1174) -> ("error out"=w1187:errorcluster, "connection reference"=w1188:T33)  [unwired: 3 in, 3 out]
            n737 = Concatenate Strings(w1232, w1231, w1228) -> (w1221:string)
            n738 = call-poly <vilib>:"DB Tools Execute Query.vi"("error in (no error)"=w1187, "SQL query"=w1221, "connection reference"=w1188) -> ("error out"=w1220:errorcluster, "recordset reference"=w1218:T34)  [unwired: 1 in, 4 out]
            n739 = call-poly <vilib>:"DB Tools Free Object.vi"("error in (no error)"=w1220, "recordset reference"=w1218) -> ("error out"=w1219:errorcluster, "connection reference"=w1217:T33)  [unwired: 8 out]
          }
          frame #2 {
            # "Experiment.expt"
            n740 = local read "LastShot"() -> (w1244:i32)
            n741 = Increment(x=w1244) -> (x+1=w1242:i32)
            n742 = for {
              tunnel: w1237 -> [w1290] mode=indexing
              tunnel: w1246 -> [w1265]
              tunnel: w1245 -> [w1249]
              tunnel: [w1263] -> w1239
              tunnel: [w1264] -> w1241
              tunnel: w1242 -> [w1270]
              tunnel: [w1262] -> w1243
              tunnel: w1238 -> [w1258]
              i -> [w1262]
              w1250 = sgl 1.0 ("f")
              # "Shot.id"
              n743 = Add(x=w1270, y=w1262) -> (x+y=w1269:i32)
              n744 = Unbundle By Name(w1290) -> ("IMPACT VELOCITY"=w1276:sgl, "Redundant_Velocity"=w1255:sgl, "RESIDUAL  VELOCITY"=w1254:sgl, "Shot Description"=w1256:string, "Powder Loading"=w1280:sgl, "Barrel Temperature"=w1281:sgl, "TIME / DATE"=w1282:string, "shot order"=w1283:i32, "Shot Angle"=w1284:u16, "BackFace\nDepth"=w1285:sgl, "BackFace\nDiameter"=w1286:sgl, "SHOT STATUS"=w1288:u16, "Projectile Mass"=w1279:sgl, "usedv50"=w1278:bool, "Energy Loss (J)"=w1277:sgl, "avgVel_PB"=w1261:sgl, "velLoss_PB"=w1260:sgl, "strikeVel_PB"=w1259:sgl, "Frag Rod"=w1247:sgl)
              n745 = local read "Drag Corrected"() -> (w1252:bool)
              n746 = local read "Residual factor"() -> (w1274:sgl)
              n747 = local read "Impact factor"() -> (w1251:sgl)
              n748 = Greater Than 0?(x=w1288) -> (x > 0?=w1287:bool)
              n749 = Select(t=w1251, s=w1252, f=w1250) -> (s? t:f=w1272:sgl)
              n750 = Select(t=w1251, s=w1252, f=w1250) -> (s? t:f=w1257:sgl)
              n751 = Select(t=w1274, s=w1252, f=w1250) -> (s? t:f=w1273:sgl)
              n752 = Divide(x=w1276, y=w1272) -> (x/y=w1271:sgl)
              n753 = Divide(x=w1255, y=w1257) -> (x/y=w1253:sgl)
              n754 = Divide(x=w1254, y=w1273) -> (x/y=w1275:sgl)
              n755 = Format Into String(format string="INSERT INTO shots (impactdc, redundantdc, residualdc,  comment, loading, barreltemp, [date], [order], shotangle, bfdepth, bfdiameter, [complete], expt, id, weight,usedv50, loss, residual, impact, redundant, avgVel_PB, velLoss_PB, strikeVel_PB, fragRod)  VALUES (%.1f, %.1f, %.1f, '%s', %.4f, %.1f, #%s#, %d, %d, %.3f, %.3f, %d, %d, %d, %.4f, %d, %.4f, %.1f, %.1f, %.1f, %.1f, %.1f, %.1f, %.1f)" ("Substring"), error in=w1249, w1276, w1255, w1254, w1256, w1280, w1281, w1282, w1283, w1284, w1285, w1286, w1287, w1258, w1269, w1279, w1278, w1277, w1275, w1271, w1253, w1261, w1260, w1259, w1247) -> (resulting string=w1266:string, error out=w1248:errorcluster)  [unwired: 1 in]
              n756 = call-poly <vilib>:"DB Tools Execute Query.vi"("error in (no error)"=w1248, "SQL query"=w1266, "connection reference"=w1265) -> ("error out"=w1268:errorcluster, "recordset reference"=w1267:T34)  [unwired: 1 in, 4 out]
              n757 = call-poly <vilib>:"DB Tools Free Object.vi"("error in (no error)"=w1268, "recordset reference"=w1267) -> ("error out"=w1263:errorcluster, "connection reference"=w1264:T33)  [unwired: 8 out]
            }
            n758 = call <vilib>:"DB Tools Close Connection.vi"("error in (no error)"=w1239, "connection reference"=w1241) -> ("error out"=w1240:errorcluster)  [unwired: 5 out]
          }
        }
        n759 = local read "configPath"() -> (w1085:path)
        n760 = case shown="No Error" w1086 {
          selector: w1086 -> [w1302 w1329]
          tunnel: [-1 -1] -> w1088
          tunnel: [Collector_State."POLL" ("progState") Collector_State."POLL" ("progState")] -> w1089
          tunnel: w1087 -> [w1313 _]
          tunnel: w1085 -> [w1297 _]
          tunnel: [w1296 w1327] -> w1083
          tunnel: w1082 -> [w1294 w1326]
          tunnel: [w1292 w1326] -> w1081
          frame No Error {
            w1303 = "Data Base Parameters" ("section")
            n761 = local read "LastShot"() -> (w1314:i32)
            n762 = Array Size(array=w1294) -> (size(s)=w1293:i32)
            n763 = flat-sequence {
              tunnel: w1296 -> [_]
              tunnel: w1291 -> [w1324]
              tunnel: [w1324] -> w1292
              frame #0 {
                w1317 = T14."Disabled and Grayed Out" ("Disabled")
                n764 = property on="saveReq" class="Str"("Visible"=TRUE) -> ()  [unwired: 2 in, 2 out]
                n765 = local write "SampleID"("") -> ()
                n766 = property on="clearShots" class="Bool"("Disabled"=T14."Enabled") -> ()  [unwired: 2 in, 2 out]
                n767 = property on="addShot" class="Bool"("Disabled"=w1317) -> ()  [unwired: 2 in, 2 out]
                n768 = property on="undoLastShot" class="Bool"("Disabled"=w1317) -> ()  [unwired: 2 in, 2 out]
                n769 = property on="saveShots" class="Bool"("Disabled"=w1317) -> ()  [unwired: 2 in, 2 out]
                n770 = One Button Dialog(message="Data Saved. Enter new Sample ID.") -> ()  [unwired: 1 in, 1 out]
                n771 = property on="mainTabCntrl" class="TabCtl (strict)"("Value"=enum32{"Setup", "Measure", "History", "System"}."Setup" ("mainTabCntrl")) -> ()  [unwired: 2 in, 2 out]
                n772 = property on="SampleEntryTabCntrl" class="TabCtl (strict)"("Value"=enum32{"Environment", "Sample"}."Sample" ("SampleEntryTabCntrl")) -> ()  [unwired: 2 in, 2 out]
                n773 = property on="Sample SubTabCntrl" class="TabCtl (strict)"("Value"=T2."General Specification" ("Sample SubTabCntrl")) -> ()  [unwired: 2 in, 2 out]
              }
            }
            n774 = Increment(x=w1314) -> (x+1=w1308:i32)
            n775 = call <vilib>:"Open Config Data (compatibility).vi"("error in (no error)"=w1302, "configuration file path"=w1297) -> ("error out"=w1307:errorcluster, "refnum"=w1306:T35)  [unwired: 7 in, 1 out]
            n776 = Add(x=w1308, y=w1313) -> (x+y=w1309:i32)
            n777 = local read "LastSample"() -> (w1310:i32)
            n778 = for {
              N: w1293 -> [_]
              shift-right: [w1315] -> w1291
              shift-left: w1294 -> [w1316]
              n779 = Delete From Array(array=w1316) -> (array with subset deleted=w1315:T7[])  [unwired: 2 in, 1 out]
            }
            n780 = local write "LastShot"(w1309) -> ()
            n781 = call-poly <vilib>:"Write Key.vi"("section"=w1303, "error in (no error)"=w1307, "value"=w1309, "key"="Last Shot Saved ", "refnum"=w1306) -> ("error out"=w1305:errorcluster, "refnum out"=w1304:T35)  [unwired: 5 out]
            n782 = Increment(x=w1310) -> (x+1=w1298:i32)
            n783 = local write "LastSample"(w1298) -> ()
            n784 = call-poly <vilib>:"Write Key.vi"("section"=w1303, "error in (no error)"=w1305, "value"=w1298, "key"="Last Panel Saved ", "refnum"=w1304) -> ("error out"=w1295:errorcluster)  [unwired: 6 out]
            n785 = To Double Precision Float(number=w1298) -> (double precision float=w1301:dbl)
            n786 = call <vilib>:"Close Config Data.vi"("error in (no error)"=w1295, "refnum"=w1304) -> ("error out"=w1296:errorcluster)  [unwired: 1 in, 8 out]
            n787 = property on="Record #" class="DigNum (strict)"("Maximum"=w1301) -> ()  [unwired: 2 in, 2 out]
            n788 = property on="SHOTS" class="Arr (strict)"("Val(Sgnl)"=w1291) -> ()  [unwired: 2 in, 2 out]
          }
          frame Error {
            n789 = One Button Dialog(message="Error saving Data. ") -> ()  [unwired: 2 out]
            n790 = call <vilib>:"General Error Handler.vi"("error in (no error)"=w1329) -> ("error out"=w1327:errorcluster)  [unwired: 2 in, 12 out]
          }
        }
      }
      frame 5 {
        # "Shot Order"
        # "This section accepts new data to the shot table."
        n791 = property on="undoLastShot" class="Bool"(error in=w1340, "Disabled"=u8 0) -> (error out=w1339:errorcluster)  [unwired: 1 in, 1 out]
        n792 = local read "residual/speed"() -> (w1365:sgl)
        n793 = local read "Impact/speed"() -> (w1369:sgl)
        n794 = Array Size(array=w1345) -> (size(s)=w1350:i32)
        n795 = Increment(x=w1350) -> (x+1=w1370:i32)
        n796 = case shown="\"grains\"" "loadingUnits" {
          tunnel: [w1377 w1378] -> w1335
          tunnel: "Powder Loading" -> [w1377 w1379]
          frame "grams", Default {
            # "Always save in grams."
          }
          frame "grains" {
            # "Always save in grams."
            n797 = Multiply(x=w1379, y=sgl 0.06479891) -> (x*y=w1378:sgl)
          }
        }
        n798 = local read "Current/residual/speed"() -> (w1353:sgl)
        n799 = local read "CorrectedVelScrnSet2"() -> (w1374:sgl)
        n800 = local read "MeasVelScrnSet2"() -> (w1371:sgl)
        n801 = local read "CorrectedVelScrnSet1"() -> (w1354:sgl)
        n802 = local read "MeasVelScrnSet1"() -> (w1372:sgl)
        n803 = local read "Current/avg/speed"() -> (w1376:sgl)
        n804 = local read "Corrected Residual"() -> (w1352:sgl)
        n805 = local read "BACKFACE DEPTH"() -> (w1356:sgl)
        n806 = local read "Redundant/speed"() -> (w1373:sgl)
        n807 = local read "conversion factor"() -> (w1363:sgl)
        n808 = local read "Projectile Mass"() -> (w1342:sgl)
        n809 = local read "SHOT STATUS"() -> (w1349:u16)
        n810 = local read "Avg/speed"() -> (w1375:sgl)
        n811 = Multiply(x=w1369, y=w1363) -> (x*y=w1361:sgl)
        n812 = Multiply(x=w1363, y=w1365) -> (x*y=w1362:sgl)
        n813 = Multiply(x=w1361, y=w1361) -> (x*y=w1357:sgl)
        n814 = Multiply(x=w1362, y=w1362) -> (x*y=w1358:sgl)
        n815 = Subtract(x=w1357, y=w1358) -> (x-y=w1359:sgl)
        n816 = Format Date/Time String(time format string (%c)="%x   %H:%M:%S") -> (date/time string=w1366:string)  [unwired: 2 out]
        "SUBMIT DATE/TIME" <- w1366
        n817 = Compound Arithmetic op=MULTIPLY(w1342, w1359, sgl 0.0005 ("Input")) -> (w1364:sgl)
        n818 = Index Array(array=w1345) -> (element=w1348:T7)  [unwired: 1 in]
        n819 = Bundle By Name(cluster=w1348, "TIME / DATE"=w1366, "shot order"=w1370, "IMPACT VELOCITY"=w1369, "RESIDUAL  VELOCITY"=w1365, "Shot Description"="Shot Description", "Powder Loading"=w1335, "Barrel Temperature"="Barrel Temp", "SHOT STATUS"=w1349, "BackFace\nDepth"=w1356, "Shot Angle"="Shot Angle", "Uncorrected Impact"=w1372, "Corrected Impact"=w1354, "Uncorrected Residual"=w1353, "Corrected residual"=w1352, "Projectile Mass"=w1342, "Energy Loss (J)"=w1364, "UncorrectedRed_PB"=w1371, "Redundant_Velocity"=w1373, "CorrectedRed_PB"=w1374, "UncorrectedAvgVel_PB"=w1376, "avgVel_PB"=w1375, "Frag Rod"="Frag Rod", "V50userExcl"=FALSE) -> (w1351:T7)
        n820 = Build Array (concatenate)(w1345, w1351) -> (w1341:T7[])
        n821 = stacked-sequence {
          tunnel: w1341 -> [w1384]
          tunnel: [w1384] -> w1332
          tunnel: w1339 -> [w1383]
          tunnel: [w1382] -> w1338
          frame #0 {
            n822 = property on="shotsTabCntrl" class="TabCtl (strict)"(error in=w1383, "Value"=T5."Shots Table" ("shotsTabCntrl")) -> (error out=w1382:errorcluster)  [unwired: 1 in, 1 out]
            n823 = local write "backdepth"(sgl 0.0 ("BACKFACE DEPTH")) -> ()
          }
        }
      }
      frame 6 {
        # "This section will clear the shot table and re-enable the \"ADD SHOT\" button to get ready for a new test panel."
        n824 = Two Button Dialog(message="Shot table cleared even if not saved. Are you sure?", 1:"NO" ("F button name (\"Cancel\")"), 2:"YES" ("T button name (\"OK\")")) -> (T button?=w1389:bool)
        n825 = case shown="True" w1389 {
          tunnel: [w1395 T7[] [] ("SHOTS")] -> w1394
          tunnel: w1390 -> [w1395 _]
          frame False {
          }
          frame True {
            w1396 = T14."Disabled and Grayed Out" ("Disabled")
            n826 = invoke on="Table of Shots" class="Tbl (strict)" method="Reinit To Default"() -> ()  [unwired: 3 in, 3 out]
            n827 = property on="addShot" class="Bool"("Disabled"=T14."Enabled") -> ()  [unwired: 2 in, 2 out]
            n828 = invoke on="SHOTS" class="Arr (strict)" method="Reinit To Default"() -> ()  [unwired: 3 in, 3 out]
            n829 = property on="saveReq" class="Str"("Visible"=TRUE) -> ()  [unwired: 2 in, 2 out]
            n830 = property on="clearShots" class="Bool"("Disabled"=w1396) -> ()  [unwired: 2 in, 2 out]
            n831 = property on="undoLastShot" class="Bool"("Disabled"=w1396) -> ()  [unwired: 2 in, 2 out]
            n832 = property on="saveShots" class="Bool"("Disabled"=w1396) -> ()  [unwired: 2 in, 2 out]
          }
        }
      }
      frame 7 {
        n833 = property on="SHOTS" class="Arr (strict)"(error in=w1402) -> (error out=w1401:errorcluster, "Index Values"=w1406:u32[])  [unwired: 1 in, 1 out]
        n834 = Array Size(array=w1413) -> (size(s)=w1409:i32)
        n835 = Index Array "Index Array"(array=w1406) -> (element=w1411:u32)  [unwired: 1 in]
        n836 = To Unsigned Long Integer(number=w1409) -> (unsigned 32bit integer=w1405:u32)
        n837 = Increment(x=w1411) -> (x+1=w1410:u32)
        n838 = Quotient & Remainder(x=w1410, y=w1405) -> (x-y*floor(x/y)=w1408:u32)  [unwired: 1 out]
        n839 = Replace Array Subset "Replace Array Subset"(array=w1406, new element=w1408) -> (w1407:u32[])  [unwired: 1 in]
        n840 = property on="SHOTS" class="Arr (strict)"(error in=w1401, "Index Values"=w1407) -> (error out=w1400:errorcluster, "Value"=w1412:T7[])  [unwired: 1 in, 1 out]
      }
      frame 8 {
        # "This section undoes new shot data OR deletes the currently accessed previous shot"
        n841 = local read "deleteShot"() -> (w1420:bool)
        n842 = case shown="True" w1420 {
          tunnel: w1419 -> [w1423 w1436]
          tunnel: [w1424 w1437] -> w1418
          frame False {
            n843 = Array Size(array=w1423) -> (size(s)=w1421:i32)
            n844 = while {
              tunnel: [w1427] -> w1422
              tunnel: w1421 -> [w1429]
              tunnel: w1423 -> [w1431] mode=indexing
              i -> [w1427]
              stop <- w1430 stop-if-true
              n845 = Unbundle By Name(w1431) -> ("shot order"=w1428:i32)
              n846 = Equal?(x=w1428, y=w1429) -> (x = y?=w1430:bool)
            }
            n847 = Delete From Array "Delete From Array"(array=w1423, index=w1422) -> (array with subset deleted=w1424:T7[])  [unwired: 1 in, 1 out]
            n848 = local write "SUBMIT DATE/TIME"("" ("Empty String Constant")) -> ()
            n849 = property on="undoLastShot" class="Bool"("Disabled"=u8 2) -> ()  [unwired: 2 in, 2 out]
          }
          frame True {
            n850 = property on="SHOTS" class="Arr (strict)"() -> ("Index Values"=w1445:u32[])  [unwired: 2 in, 2 out]
            n851 = local write "deleteShot"(FALSE) -> ()
            n852 = Index Array(array=w1445, index=0 ("Index")) -> (element=w1435:u32)
            n853 = To Long Integer(number=w1435) -> (32bit integer=w1432:i32)
            n854 = Index Array(array=w1436, index=w1432) -> (element=w1434:T7)
            n855 = Unbundle By Name(w1434) -> ("shot order"=w1433:i32)
            n856 = Format Into String(format string="The currently displayed Shot, #%d", w1433) -> (resulting string=w1442:string)  [unwired: 2 in, 1 out]
            n857 = Concatenate Strings(w1442, ", will be deleted.  IT CANNOT RECOVERED!  Do you want to DELETE the shot?" ("message")) -> (w1441:string)
            n858 = Two Button Dialog(message=w1441, 1:"NO I do NOT want to delete.  Cancel Request" ("F button name (\"Cancel\")"), 2:"YES I want to delete the shot" ("T button name (\"OK\")")) -> (T button?=w1448:bool)
            n859 = case shown="True" w1448 {
              tunnel: w1436 -> [w1461 w1464]
              tunnel: [w1461 w1466] -> w1439
              tunnel: w1432 -> [_ w1463]
              tunnel: [10000 ("shot order") w1465] -> w1438
              frame False {
              }
              frame True {
                n860 = Index Array(array=w1464, index=w1463) -> (element=w1462:T7)
                n861 = Unbundle By Name(w1462) -> ("shot order"=w1465:i32)
                n862 = Delete From Array(array=w1464, index=w1463) -> (array with subset deleted=w1466:T7[])  [unwired: 1 in, 1 out]
              }
            }
            n863 = for {
              tunnel: [w1455] -> w1437 mode=indexing
              tunnel: w1439 -> [w1450] mode=indexing
              tunnel: w1438 -> [w1454]
              n864 = Unbundle By Name(w1450) -> ("shot order"=w1452:i32)
              n865 = Decrement(x=w1452) -> (x-1=w1451:i32)
              n866 = Greater?(x=w1452, y=w1454) -> (0:w1453:bool)
              n867 = case shown="True" w1453 {
                tunnel: w1451 -> [_ w1458]
                tunnel: w1450 -> [w1456 w1459]
                tunnel: [w1456 w1457] -> w1455
                frame False {
                }
                frame True {
                  n868 = Bundle By Name(cluster=w1459, "shot order"=w1458) -> (w1457:T7)
                }
              }
            }
          }
        }
        n869 = property on="SHOTS" class="Arr (strict)"(error in=w1414, "Val(Sgnl)"=w1418) -> (error out=w1415:errorcluster)  [unwired: 1 in, 1 out]
      }
      frame 9 {
        n870 = local write "SUBMIT DATE/TIME"("" ("Empty String Constant")) -> ()
        n871 = Concatenate Strings("L|", "6|") -> (w1473:string)
        n872 = case shown="\"Screens\"" "MeasSrc" {
          tunnel: w1473 -> [_ _ w1489]
          tunnel: w1468 -> [w1479 w1484 w1488]
          tunnel: [w1477 w1484 w1485] -> w1467
          frame "Simulated", Default {
            n873 = flat-sequence {
              tunnel: w1479 -> [w1480]
              tunnel: [w1480] -> w1478
              tunnel: [w1482] -> w1477
              tunnel: w1478 -> [w1482]
              frame #0 {
                n874 = local write "readyClock"(FALSE ("RANGE RESET")) -> ()
              }
              frame #1 {
                n875 = Wait (ms)(milliseconds to wait=u32 100) -> ()  [unwired: 1 out]
              }
            }
          }
          frame "Radar" {
          }
          frame "Screens" {
            w1495 = u32 22 items=["NI-DAQ version", "device name", "base address", "data transfer mode for analog input", "data transfer mode for analog output group 1", "data transfer mode for analog output group 2", "data transfer mode for GPCTR 0", "data transfer mode for GPCTR 1", "data transfer mode for digital I/O group 1", "data transfer mode for digital I/O group 2", "device type code", "DMA A level", "DMA B level", "DMA C level", "interrupt A level", "interrupt B level", "reserved", "lpt device mode", "DAQCard-700 counter 1 source", "interrupt generation mode", "device state during suspend mode", "computer name", "serial number", "counter type", "Scarab A Memory Size", "Scarab B Memory Size"] ("information type")
            w1494 = u32 1  # device
            n876 = Concatenate Strings(w1489, "2|") -> (w1490:string)
            n877 = call <vilib>:"Get DAQ Device Information.vi"("error in (no error)"=w1488, "information type"=w1495, "task ID or device"=w1494) -> ("error out"=w1487:errorcluster, "information string"=w1493:string)  [unwired: 7 out]
            n878 = disable-structure "Diagram Disable Structure" shown="Enabled" {
              disable-tunnel: w1490 -> [w1500 _]
              disable-tunnel: w1487 -> [w1497 w1502]
              disable-tunnel: [w1496 w1502] -> w1486
              frame Disabled {
                n879 = Current VI's Path() -> (path=w1501:path)
                n880 = call "Where Am I (SubVI).vi"("TL Calling Location"=w1500, "Call VI path"=w1501) -> ("I'm here"=w1499:string)
                n881 = call "Error Check (SubVI).vi"("calling VI"=w1499, "tag #"=0, "error IN"=w1497) -> ("error OUT"=w1496:errorcluster)  [unwired: 2 in]
              }
              frame Enabled {
                # "Debug code is disabled"
              }
            }
            n882 = case shown="No Error" w1486 {
              selector: w1486 -> [w1503 _]
              tunnel: w1493 -> [w1513 _]
              tunnel: [w1513 "DEVICE NOT READY!" ("information string")] -> w1492
              tunnel: [w1504 errorcluster {"status"=FALSE, "code"=0, "source"=""} ("error out")] -> w1485
              frame No Error {
                # "assign task IDs to counters"
                n883 = call "Config Counter to Measure Two Edge Separation.vi"("error IN"=w1503, "Counter"="Impact Timer", "device"="DAQ Card") -> ("error out"=w1515:errorcluster, "task ID out"=w1509:u32)  [unwired: 1 in]
                "impact/ID" <- w1509
                n884 = local write "readyClock"(FALSE ("RANGE RESET")) -> ()
                n885 = call "Config Counter to Measure Two Edge Separation.vi"("error IN"=w1515, "Counter"="Residual  Timer", "device"="DAQ Card") -> ("error out"=w1517:errorcluster, "task ID out"=w1507:u32)  [unwired: 1 in]
                "residual/ID" <- w1507
                n886 = call "Config Counter to Measure Two Edge Separation.vi"("error IN"=w1517, "Counter"="Redundant Timer", "device"="DAQ Card") -> ("error out"=w1516:errorcluster, "task ID out"=w1508:u32)  [unwired: 1 in]
                "Red/ID" <- w1508
                n887 = Bundle("task ID out"=w1509, "task ID out"=w1508, "task ID out"=w1507) -> (w1505:T36)  [unwired: 1 out]
                n888 = call <vilib>:"Simple Error Handler.vi"("error in (no error)"=w1516) -> ("error out"=w1504:errorcluster)  [unwired: 1 in, 7 out]
                n889 = global write "BIMS_Collector Globals.vi" "Screens"(w1505) -> ()
              }
              frame Error {
                n890 = One Button Dialog(message="Error initializing Timer board.  Switching to simulation") -> ()  [unwired: 2 out]
                n891 = local write "MeasSrc"(DataSource."Simulated" ("MeasSrc")) -> ()
              }
            }
            "Device S/N" <- w1492
          }
        }
      }
      frame 9 {
        n892 = local write "processShots"(FALSE ("ProcessShots")) -> ()
        n893 = local read "Drag Corrected"() -> (w1527:bool)
        n894 = stacked-sequence {
          seq-local: [_ w1585 _ _] -> [_ _ w1614 w1664]
          seq-local: [w1549 _ _ _] -> [_ w1581 _ _]
          seq-local: [w1547 _ _ _] -> [_ w1582 _ _]
          seq-local: [w1548 _ _ _] -> [_ w1583 _ _]
          tunnel: [_ _ _ w1657] -> w1528
          tunnel: w1527 -> [w1551 w1584 _ _]
          tunnel: w1524 -> [_ w1580 _ _]
          tunnel: w1523 -> [w1546 _ _ _]
          tunnel: [w1546 _ _ _] -> w1522
          frame #0 {
            n895 = disable-structure "Diagram Disable Structure" shown="Enabled" {
              disable-tunnel: [w1568 w1575] -> w1556
              frame Disabled {
                n896 = local read "factor array"() -> (w1570:sgl[])
                n897 = local read "Threat"() -> (w1567:u16)
                n898 = To Long Integer(number=w1567) -> (32bit integer=w1569:i32)
                n899 = Index Array(array=w1570, index=w1569) -> (element=w1568:sgl)
              }
              frame Enabled {
                n900 = local read "threatDetails"() -> (w1574:T1)
                n901 = Unbundle By Name(w1574) -> ("dragCorrection"=w1572:string)
                n902 = Not Equal?(x=w1572, y="") -> (x != y?=w1573:bool)
                n903 = case shown="True" w1573 {
                  tunnel: [sgl 1.0 ("default value 1") w1578] -> w1575
                  tunnel: w1572 -> [_ w1577]
                  frame False {
                  }
                  frame True {
                    n904 = Scan From String(input string=w1577, default 1=sgl 0.0 ("default value 1")) -> (output 1=w1578:sgl)  [unwired: 3 in, 3 out]
                  }
                }
              }
            }
            "correction coefficient" <- w1556
            n905 = local read "Current/avg/speed"() -> (w1552:sgl)
            n906 = local read "mid_to_targ_dist"() -> (w1553:sgl)
            n907 = local read "lengthUnits"() -> (w1550:string)
            n908 = call "Compute Strike Velocity.vi"("drag coefficient"=w1556, "decay distance"=w1553, "raw velocity"=w1552, "distance units"=w1550) -> ("correction factor"=w1549:sgl, "strike velocity"=w1554:sgl)  [unwired: 1 out]
            "DC_ factor" <- w1549
            "Corrected Average" <- w1554
            n909 = call "Velocity Correction.vi"("raw impact"="MeasVelScrnSet1", "distance units"=w1550, "raw redundant"="MeasVelScrnSet2", "raw residual"="Current/residual/speed", "screen set midpt to target"="Set#1_to_Target", "residual screen to target"="Residual/Target Dist", "correction coefficient"=w1556) -> ("corrected impact"=w1561:sgl, "corrected redundant"=w1557:sgl, "corrected residual"=w1559:sgl, "impact factor"=w1547:sgl, "conversion factor"=→"conversion factor":sgl, "residual factor"=w1548:sgl)  [unwired: 3 out]
            "Residual factor" <- w1548
            "Impact factor" <- w1547
            "CorrectedVelScrnSet1" <- w1561
            "Corrected Residual" <- w1559
            "CorrectedVelScrnSet2" <- w1557
            n910 = Select(t=w1557, s=w1551, f="MeasVelScrnSet2") -> (s? t:f=→"Redundant/speed":sgl)
            n911 = Select(t=w1554, s=w1551, f=w1552) -> (s? t:f=→"Avg/speed":sgl)
            n912 = Select(t=w1561, s=w1551, f="MeasVelScrnSet1") -> (s? t:f=→"Impact/speed":sgl)
            n913 = Select(t=w1559, s=w1551, f="Current/residual/speed") -> (s? t:f=→"residual/speed":sgl)
            n914 = Add(x="MeasVelScrnSet2", y="MeasVelScrnSet1") -> (x+y=w1533:sgl)
            n915 = Subtract(x="MeasVelScrnSet2", y="MeasVelScrnSet1") -> (x-y=w1532:sgl)
            n916 = Divide(x=w1533, y=sgl 200.0) -> (x/y=w1534:sgl)
            n917 = Divide(x=w1532, y=w1534) -> (x/y=w1538:sgl)
            "%_Difference" <- w1538
            n918 = Absolute Value(x=w1538) -> (abs(x)=w1540:sgl)
            n919 = Less?(x=w1540, y="percent warning") -> (x < y?=w1545:bool)
            n920 = Select(t=u32 65343, s=w1545, f=u32 15668992) -> (s? t:f=w1541:u32)
            n921 = Select(t=u32 0, s=w1545, f=u32 16777226) -> (s? t:f=w1544:u32)
            n922 = property on="%_Difference" class="DigNum (strict)"("Numeric Text.Text Colors:BG Color"=w1541, "NumText.TextColor"=w1544) -> ()  [unwired: 2 in, 2 out]
          }
          frame #1 {
            # "<-- DC_factor (for Average of impact and redundant)"
            # "IF drag corrected THEN apply factors"
            # "Residual factor"
            # "Impact factor\n(also applies to\nredundant velocity)"
            n923 = for {
              tunnel: w1580 -> [w1593] mode=indexing
              tunnel: w1583 -> [w1602]
              tunnel: w1582 -> [w1597]
              tunnel: w1584 -> [w1591]
              tunnel: [w1604] -> w1585 mode=indexing
              tunnel: w1581 -> [w1586]
              n924 = Unbundle By Name(w1593) -> ("UncorrectedAvgVel_PB"=w1592:sgl)
              n925 = Unbundle By Name(w1593) -> ("Uncorrected Impact"=w1596:sgl)
              n926 = Unbundle By Name(w1593) -> ("Uncorrected Residual"=w1601:sgl)
              n927 = Unbundle By Name(w1593) -> ("UncorrectedRed_PB"=w1599:sgl)
              n928 = Multiply(x=w1586, y=w1592) -> (x*y=w1589:sgl)
              n929 = Multiply(x=w1597, y=w1599) -> (x*y=w1598:sgl)
              n930 = Multiply(x=w1597, y=w1596) -> (x*y=w1587:sgl)
              n931 = Multiply(x=w1602, y=w1601) -> (x*y=w1594:sgl)
              n932 = Select(t=w1589, s=w1591, f=w1592) -> (s? t:f=w1590:sgl)
              n933 = Select(t=w1598, s=w1591, f=w1599) -> (s? t:f=w1600:sgl)
              n934 = Select(t=w1594, s=w1591, f=w1601) -> (s? t:f=w1603:sgl)
              n935 = Select(t=w1587, s=w1591, f=w1596) -> (s? t:f=w1595:sgl)
              n936 = Subtract(x=w1590, y=w1589) -> (x-y=w1588:sgl)
              n937 = Bundle By Name(cluster=w1593, "velLoss_PB"=w1588, "strikeVel_PB"=w1589, "avgVel_PB"=w1590, "CorrectedRed_PB"=w1598, "Redundant_Velocity"=w1600, "Corrected Impact"=w1587, "IMPACT VELOCITY"=w1595, "Corrected residual"=w1594, "RESIDUAL  VELOCITY"=w1603) -> (w1604:T7)
            }
          }
          frame #2 {
            w1615 = sgl[] [] ("Partial")
            # "This section calculates the V50"
            n938 = for {
              shift-right: [w1639] -> w1617
              shift-left: w1615 -> [w1640]
              shift-right: [w1637] -> w1616
              shift-left: w1615 -> [w1638]
              tunnel: w1614 -> [w1631] mode=indexing
              n939 = Unbundle By Name(w1631) -> ("SHOT STATUS"=w1636:u16)
              n940 = Unbundle By Name(w1631) -> ("V50userExcl"=w1630:bool)
              n941 = Unbundle By Name(w1631) -> ("IMPACT VELOCITY"=w1635:sgl)
              n942 = Unbundle By Name(w1631) -> ("strikeVel_PB"=w1634:sgl)
              n943 = Select(t=w1634, s="ScreenSetAvgg", f=w1635) -> (s? t:f=w1633:sgl)
              n944 = case shown="False" w1630 {
                tunnel: w1640 -> [w1646 w1656]
                tunnel: [w1645 w1656] -> w1639
                tunnel: w1638 -> [w1644 w1655]
                tunnel: [w1643 w1655] -> w1637
                tunnel: w1636 -> [w1642 _]
                tunnel: w1633 -> [w1641 _]
                frame False {
                  n945 = case shown="1" w1642 {
                    tunnel: w1641 -> [w1647 w1651]
                    tunnel: [w1650 w1652] -> w1645
                    tunnel: w1646 -> [w1649 w1652]
                    tunnel: w1644 -> [w1648 w1654]
                    tunnel: [w1648 w1653] -> w1643
                    frame 0, Default {
                      n946 = Build Array (concatenate)(w1649, w1647) -> (w1650:sgl[])
                    }
                    frame 1 {
                      n947 = Build Array (concatenate)(w1654, w1651) -> (w1653:sgl[])
                    }
                  }
                }
                frame True {
                }
              }
            }
            n948 = Sort 1D Array(array=w1617) -> (sorted array=w1629:sgl[])
            n949 = Sort 1D Array(array=w1616) -> (sorted array=w1622:sgl[])
            "Complete" <- w1622
            n950 = Reverse 1D Array(array=w1629) -> (reversed array=w1620:sgl[])
            "Partial" <- w1620
            n951 = Array Size(array=w1622) -> (size(s)=→"#_completes":i32)
            n952 = Array Size(array=w1620) -> (size(s)=→"#_partials":i32)
            n953 = Array Max & Min(array=w1620) -> (max value=w1626:sgl)  [unwired: 3 out]
            n954 = Array Max & Min(array=w1622) -> (min value=w1624:sgl)  [unwired: 3 out]
            n955 = call "Compute V50.vi"("Partial"=w1620, "Maximum Deviation"="maxDev", "Complete"=w1622) -> ("Pairs"=→"Pairs":i16, "zmr"=w1605:sgl, "V50"=→"computed_V50":sgl)  [unwired: 2 out]
            "Z.M.R." <- w1605
            n956 = To Long Integer(number=w1626) -> (32bit integer=→"highPartial":i32)
            n957 = To Long Integer(number=w1624) -> (32bit integer=→"lowComplete":i32)
            n958 = Absolute Value(x=w1605) -> (abs(x)=→"zmr 2":sgl)
            n959 = Less Than 0?(x=w1605) -> (x < 0?=w1608:bool)
            n960 = Select(t="Low C minus High P", s=w1608, f="ZMR") -> (s? t:f=w1611:string)
            n961 = Select(t=u32 65336, s=w1608, f=u32 16755266) -> (s? t:f=w1612:u32)
            n962 = property on="zmr 2" class="DigNum (strict)"("Caption.Text"=w1611, "Numeric Text.Text Colors:BG Color"=w1612) -> ()  [unwired: 2 in, 2 out]
          }
          frame #3 {
            n963 = local read "Pairs"() -> (w1669:i16)
            n964 = Sort 1D Array(array=w1664) -> (sorted array=w1667:T7[])
            n965 = for {
              tunnel: w1667 -> [w1713] mode=indexing
              tunnel: w1669 -> [w1723]
              shift-right: [w1722] -> _
              shift-left: i16 0 -> [w1721]
              tunnel: [w1715] -> w1665 mode=indexing
              # "this section marks the lowest completes that are used in V50"
              n966 = Unbundle By Name(w1713) -> ("SHOT STATUS"=w1719:u16, "Projectile Mass"=w1717:sgl, "avgVel_PB"=w1716:sgl, "RESIDUAL  VELOCITY"=w1718:sgl)
              n967 = Unbundle By Name(w1713) -> ("V50userExcl"=w1714:bool)
              n968 = local read "conversion factor"() -> (w1725:sgl)
              n969 = case shown="True" w1714 {
                tunnel: w1723 -> [w1736 _]
                tunnel: [w1735 w1745] -> w1722
                tunnel: w1721 -> [w1734 w1745]
                tunnel: [w1733 FALSE] -> w1720
                tunnel: w1719 -> [w1732 _]
                frame False {
                  n970 = case shown="1" w1732 {
                    tunnel: w1736 -> [_ w1743]
                    tunnel: [FALSE w1742] -> w1733
                    tunnel: [w1738 w1741] -> w1735
                    tunnel: w1734 -> [w1738 w1739]
                    frame 0, Default {
                    }
                    frame 1 {
                      n971 = Less?(x=w1739, y=w1743) -> (x < y?=w1742:bool)
                      n972 = Add(x=w1739, y=i16 1 ("t")) -> (x+y=w1741:i16)
                    }
                  }
                }
                frame True {
                }
              }
              n973 = Multiply(x=w1725, y=w1718) -> (x*y=w1726:sgl)
              n974 = Multiply(x=w1716, y=w1725) -> (x*y=w1727:sgl)
              n975 = Multiply(x=w1727, y=w1727) -> (x*y=w1731:sgl)
              n976 = Multiply(x=w1726, y=w1726) -> (x*y=w1730:sgl)
              n977 = Subtract(x=w1731, y=w1730) -> (x-y=w1729:sgl)
              n978 = Compound Arithmetic op=MULTIPLY(w1717, w1729, sgl 0.0005 ("Input")) -> (w1724:sgl)
              n979 = Bundle By Name(cluster=w1713, "usedv50"=w1720, "Energy Loss (J)"=w1724) -> (w1715:T7)
            }
            n980 = Reverse 1D Array(array=w1665) -> (reversed array=w1666:T7[])
            n981 = for {
              tunnel: w1666 -> [w1689] mode=indexing
              tunnel: w1669 -> [w1696]
              shift-right: [w1694] -> _
              shift-left: i16 0 -> [w1695]
              tunnel: [w1692] -> w1657 mode=indexing
              # "chooses highest partials used in v50"
              n982 = Unbundle By Name(w1689) -> ("SHOT STATUS"=w1697:u16, "usedv50"=w1691:bool)
              n983 = Unbundle By Name(w1689) -> ("V50userExcl"=w1690:bool)
              n984 = case shown="True" w1690 {
                tunnel: w1697 -> [w1703 _]
                tunnel: w1696 -> [w1702 _]
                tunnel: w1695 -> [w1701 w1712]
                tunnel: [w1700 w1712] -> w1694
                tunnel: [w1699 FALSE ("usedv50")] -> w1693
                tunnel: w1691 -> [w1698 _]
                frame False {
                  n985 = case shown="1" w1703 {
                    tunnel: w1702 -> [w1707 _]
                    tunnel: [w1706 w1710] -> w1699
                    tunnel: w1701 -> [w1704 w1709]
                    tunnel: [w1705 w1709] -> w1700
                    tunnel: w1698 -> [_ w1710]
                    frame 0, Default {
                      n986 = Less?(x=w1704, y=w1707) -> (x < y?=w1706:bool)
                      n987 = Add(x=w1704, y=i16 1) -> (x+y=w1705:i16)
                    }
                    frame 1 {
                    }
                  }
                }
                frame True {
                }
              }
              n988 = Bundle By Name(cluster=w1689, "usedv50"=w1693) -> (w1692:T7)
            }
            n989 = for {
              shift-right: [w1675] -> w1658
              shift-left: sgl[] [] ("Partial") -> [w1672]
              tunnel: w1657 -> [w1674] mode=indexing
              n990 = local read "ScreenSetAvgg"() -> (w1679:bool)
              n991 = Unbundle By Name(w1674) -> ("V50userExcl"=w1673:bool, "usedv50"=w1671:bool)
              n992 = Unbundle By Name(w1674) -> ("IMPACT VELOCITY"=w1677:sgl)
              n993 = Unbundle By Name(w1674) -> ("strikeVel_PB"=w1678:sgl)
              n994 = Select(t=w1678, s=w1679, f=w1677) -> (s? t:f=w1676:sgl)
              n995 = case shown="False" w1673 {
                tunnel: w1676 -> [w1680 _]
                tunnel: [w1681 w1688] -> w1675
                tunnel: w1672 -> [w1682 w1688]
                tunnel: w1671 -> [w1683 _]
                frame False {
                  n996 = case shown="True" w1683 {
                    tunnel: w1682 -> [w1684 w1687]
                    tunnel: [w1684 w1686] -> w1681
                    tunnel: w1680 -> [_ w1685]
                    frame False {
                    }
                    frame True {
                      n997 = Build Array (concatenate)(w1687, w1685) -> (w1686:sgl[])
                    }
                  }
                }
                frame True {
                }
              }
            }
            n998 = Array Max & Min(array=w1658) -> (max value=w1663:sgl, min value=w1662:sgl)  [unwired: 2 out]
            n999 = Subtract(x=w1663, y=w1662) -> (x-y=w1661:sgl)
            n1000 = property on="SHOTS" class="Arr (strict)"("Val(Sgnl)"=w1657) -> ()  [unwired: 2 in, 2 out]
            n1001 = To Long Integer(number=w1661) -> (32bit integer=→"rangeOfResults":i32)
          }
        }
      }
      frame 11 {
        n1002 = local read "SafetyInterlock"() -> (w1754:cluster{"ARMED":bool})
        n1003 = Unbundle By Name(w1754) -> ("ARMED"=w1753:bool)
        n1004 = Not(x="InterlockExists") -> (.not. x?=w1749:bool)
        n1005 = Or(x=w1753, y=w1749) -> (x .or. y?=w1750:bool)
        n1006 = case shown="True" w1750 {
          tunnel: [Collector_State."POLL" ("progState") w1763] -> w1752
          tunnel: [-1 ("index of element") w1762] -> w1751
          tunnel: "InterlockExists" -> [_ w1761]
          tunnel: [w1756 w1760] -> w1747
          tunnel: w1746 -> [w1756 w1759]
          frame False {
          }
          frame True {
            n1007 = stacked-sequence {
              tunnel: [_ Collector_State."PROCESS SHOTS" ("progState")] -> w1763
              tunnel: [_ -1] -> w1762
              tunnel: w1761 -> [w1766 _]
              tunnel: [w1764 _] -> w1760
              tunnel: w1759 -> [w1765 _]
              frame #0 {
                n1008 = local read "MeasSrc"() -> (w1768:T6)
                n1009 = case shown="\"Screens\"" w1768 {
                  tunnel: [w1771 w1795 w1806] -> w1767
                  tunnel: w1766 -> [_ _ w1804]
                  tunnel: w1765 -> [w1769 w1794 w1802]
                  tunnel: [w1769 w1794 w1803] -> w1764
                  frame "Simulated", Default {
                    # "Simulated"
                    n1010 = local read "minV50"() -> (w1777:i32)
                    n1011 = local read "Powder Loading"() -> (w1793:sgl)
                    n1012 = To Single Precision Float(number=w1777) -> (single precision float=w1776:sgl)
                    n1013 = call "Get Shell Speed.vi"("loading"=w1793, "v50"=w1776) -> ("impact"=w1781:sgl, "residual"=w1788:sgl)  [unwired: 1 in, 2 out]
                    n1014 = Random Number (0-1)() -> (number: 0 to 1=w1786:dbl)
                    n1015 = To Single Precision Float(number=w1786) -> (single precision float=w1782:sgl)
                    n1016 = Multiply(x=w1782, y=sgl 0.002) -> (x*y=w1785:sgl)
                    n1017 = local read "SafetyInterlock"() -> (w1772:cluster{"ARMED":bool})
                    n1018 = Add(x=w1785, y=sgl 0.999) -> (x+y=w1783:sgl)
                    n1019 = Greater Than 0?(x=w1788) -> (x > 0?=w1790:bool)
                    n1020 = Multiply(x=w1781, y=w1783) -> (x*y=w1780:sgl)
                    n1021 = Bundle By Name(cluster=w1772, "ARMED"=FALSE) -> (w1773:cluster{"ARMED":bool})
                    n1022 = Add(x=w1781, y=w1780) -> (x+y=w1778:sgl)
                    n1023 = Select(t=u16 1, s=w1790, f=u16 0) -> (s? t:f=w1789:u16)
                    n1024 = local write "readyClock"(TRUE ("RANGE RESET")) -> ()
                    n1025 = local write "SafetyInterlock"(w1773) -> ()
                    n1026 = Divide(x=w1778, y=sgl 2.0 ("v50")) -> (x/y=w1771:sgl)
                    n1027 = local write "Current/residual/speed"(w1788) -> ()
                    n1028 = local write "SHOT STATUS"(w1789) -> ()
                    n1029 = local write "Current/sthotstatus"(w1789) -> ()
                    n1030 = local write "MeasVelScrnSet1"(w1781) -> ()
                    n1031 = local write "MeasVelScrnSet2"(w1780) -> ()
                    n1032 = Wait (ms)(milliseconds to wait=u32 500 ("number")) -> ()  [unwired: 1 out]
                  }
                  frame "Radar" {
                    # "Radar -- (future)"
                    n1033 = local read "MeasVelScrnSet1"() -> (w1797:sgl)
                    n1034 = local read "MeasVelScrnSet2"() -> (w1796:sgl)
                    n1035 = Add(x=w1797, y=w1796) -> (x+y=w1798:sgl)
                    n1036 = Divide(x=w1798, y=sgl 2.0) -> (x/y=w1795:sgl)
                  }
                  frame "Screens" {
                    # "This section checks to see if the counters have been fired.  If they have then the counter times are read"
                    n1037 = Concatenate Strings("-1|", "F0|") -> (w1807:string)
                    n1038 = case shown="True" w1804 {
                      tunnel: w1802 -> [w1814 w1815]
                      tunnel: [w1814 w1815] -> w1801
                      frame False {
                      }
                      frame True {
                      }
                    }
                    n1039 = global read "BIMS_Collector Globals.vi" "Screens"() -> (w1805)
                    n1040 = Unbundle By Name(w1805) -> ("ScrnSet1CntrID"=w1810)
                    n1041 = Concatenate Strings(w1807, "2|") -> (w1811:string)
                    n1042 = call "Check DAQ Status.vi"("errIN"=w1801, "TL Calling Location"=w1811, "Task ID"=w1810) -> ("error out"=w1813:errorcluster, "Armed?"=w1800:bool)  [unwired: 1 out]
                    n1043 = case shown="False" w1800 {
                      tunnel: w1813 -> [w1843 w1881]
                      tunnel: w1810 -> [w1826 _]
                      tunnel: w1811 -> [w1839 _]
                      tunnel: w1805 -> [w1829 _]
                      tunnel: [w1817 w1882] -> w1806
                      tunnel: [w1816 w1881] -> w1803
                      frame False {
                        n1044 = local read "Set#1 Separation"() -> (w1846:sgl)
                        n1045 = Concatenate Strings(w1839, "F|") -> (w1834:string)
                        n1046 = call "Read TIO Count.vi"("TL Calling Location"=w1834, "error In"=w1843, "task IN"=w1826) -> ("error out"=w1828:errorcluster, "time (secs)"=w1848:sgl)  [unwired: 1 in, 4 out]
                        n1047 = Divide(x=w1846, y=w1848) -> (x/y=w1822:sgl)
                        n1048 = call "Arm TIO Channel.vi"("error IN"=w1828, "task ID IN"=w1826) -> ("error out"=w1827:errorcluster)  [unwired: 1 in, 2 out]
                        n1049 = Unbundle By Name(w1829) -> ("ScrnSet2CntrID"=w1831)
                        n1050 = Concatenate Strings(w1834, "a|") -> (w1837:string)
                        n1051 = call "Check DAQ Status.vi"("errIN"=w1827, "TL Calling Location"=w1837, "Task ID"=w1831) -> ("error out"=w1842:errorcluster, "Armed?"=w1833:bool)  [unwired: 1 out]
                        n1052 = case shown="False" w1833 {
                          tunnel: [w1859 sgl 0.0] -> w1823
                          tunnel: w1842 -> [w1858 w1863]
                          tunnel: [w1853 w1863] -> w1844
                          tunnel: w1831 -> [w1852 _]
                          tunnel: w1834 -> [w1856 _]
                          frame False {
                            n1053 = local read "Set#2 Separation"() -> (w1860:sgl)
                            n1054 = Concatenate Strings(w1856, "Fa|") -> (w1855:string)
                            n1055 = call "Read TIO Count.vi"("TL Calling Location"=w1855, "error In"=w1858, "task IN"=w1852) -> ("error out"=w1854:errorcluster, "time (secs)"=w1861:sgl)  [unwired: 1 in, 4 out]
                            n1056 = Divide(x=w1860, y=w1861) -> (x/y=w1859:sgl)
                            n1057 = call "Arm TIO Channel.vi"("error IN"=w1854, "task ID IN"=w1852) -> ("error out"=w1853:errorcluster)  [unwired: 1 in, 2 out]
                          }
                          frame True {
                          }
                        }
                        n1058 = Unbundle By Name(w1829) -> ("residualCntrID"=w1830)
                        n1059 = Add(x=w1822, y=w1823) -> (x+y=w1824:sgl)
                        n1060 = Concatenate Strings(w1834, "b|") -> (w1835:string)
                        n1061 = call "Check DAQ Status.vi"("errIN"=w1844, "TL Calling Location"=w1835, "Task ID"=w1830) -> ("error out"=w1841:errorcluster, "Armed?"=w1832:bool)  [unwired: 1 out]
                        n1062 = Divide(x=w1824, y=sgl 2.0) -> (x/y=w1817:sgl)
                        n1063 = case shown="True" w1832 {
                          tunnel: w1841 -> [w1870 w1879]
                          tunnel: [w1875 w1880] -> w1847
                          tunnel: w1830 -> [w1865 _]
                          tunnel: [w1864 w1879] -> w1818
                          tunnel: [w1872 sgl 0.0] -> w1845
                          tunnel: w1834 -> [w1867 _]
                          frame False {
                            w1876 = u16 1 items=["Partial", "Complete"] ("SHOT STATUS")
                            w1877 = u16 0 items=["Partial", "Complete"] ("SHOT STATUS")
                            n1064 = local read "Residual/Separation"() -> (w1871:sgl)
                            n1065 = Concatenate Strings(w1867, "Fb|") -> (w1868:string)
                            n1066 = call "Read TIO Count.vi"("TL Calling Location"=w1868, "error In"=w1870, "task IN"=w1865) -> ("error out"=w1866:errorcluster, "timeout"=w1873:bool, "time (secs)"=w1874:sgl)  [unwired: 1 in, 3 out]
                            n1067 = Divide(x=w1871, y=w1874) -> (x/y=w1872:sgl)
                            n1068 = call "Arm TIO Channel.vi"("error IN"=w1866, "task ID IN"=w1865) -> ("error out"=w1864:errorcluster)  [unwired: 1 in, 2 out]
                            n1069 = Select(t=w1877, s=w1873, f=w1876) -> (s? t:f=w1875:u16)
                          }
                          frame True {
                            w1880 = u16 1 items=["Partial", "Complete"] ("SHOT STATUS")
                          }
                        }
                        n1070 = local write "Current/residual/speed"(w1845) -> ()
                        n1071 = local write "MeasVelScrnSet1"(w1822) -> ()
                        n1072 = local write "MeasVelScrnSet2"(w1823) -> ()
                        n1073 = local write "SHOT STATUS"(w1847) -> ()
                        n1074 = local write "Current/sthotstatus"(w1847) -> ()
                        n1075 = case shown="No Error" w1818 {
                          selector: w1818 -> [w1851 _]
                          frame No Error {
                            # "=false"
                            n1076 = Unbundle By Name(w1851) -> ("status"=w1850:bool)
                            n1077 = Not(x=w1850) -> (.not. x?=w1849:bool)
                            n1078 = local write "readyClock"(w1849) -> ()
                          }
                          frame Error {
                          }
                        }
                        n1079 = local read "SafetyInterlock"() -> (w1819:cluster{"ARMED":bool})
                        n1080 = Bundle By Name(cluster=w1819, "ARMED"=FALSE) -> (w1820:cluster{"ARMED":bool})
                        n1081 = local write "SafetyInterlock"(w1820) -> ()
                        n1082 = call <vilib>:"Simple Error Handler.vi"("error in (no error)"=w1818) -> ("error out"=w1816:errorcluster)  [unwired: 1 in, 7 out]
                      }
                      frame True {
                        # "Error -10600 occurrs in \"Read Count.vi\"\n\n  Possible reason(s): NI-DAQ LV: No setup operation has been performed for the specified resources. Or, some resources require a specific ordering of calls for proper setup.  \n\n  Solution: To avoid this error, you must call the Dig_Line_Config function to setup the direction for each digital line prior to calling the Dig_Grp_Config function."
                        n1083 = local read "MeasVelScrnSet1"() -> (w1884:sgl)
                        n1084 = local read "MeasVelScrnSet2"() -> (w1883:sgl)
                        n1085 = Add(x=w1884, y=w1883) -> (x+y=w1885:sgl)
                        n1086 = Divide(x=w1885, y=sgl 2.0) -> (x/y=w1882:sgl)
                      }
                    }
                  }
                }
                "Current/avg/speed" <- w1767
              }
              frame #1 {
              }
            }
          }
        }
      }
    }
    "SMErr" <- w13
  }
  n1087 = while "U/I Event Handler" {
    shift-right: [w1890] -> _
    shift-left: w7 -> [w1891]
    stop <- FALSE stop-if-true
    n1088 = event shown="[23] \"RefreshMetadata\": Value Change" {
      selector: _ -> [_ _ _ _ _ _ _ _ _ _ _ _ _ _ _ _ _ _ _ _ _ _ _ _ _ _]
      dyn-events: _ -> [_ _ _ _ _ _ _ _ _ _ _ _ _ _ _ _ _ _ _ _ _ _ _ _ _ _]
      timeout: 100 -> [_ _ _ _ _ _ _ _ _ _ _ _ _ _ _ _ _ _ _ _ _ _ _ _ _ _]
      tunnel: w1891 -> [w1895 _ w1912 w1922 w1931 w1941 w1978 w2004 w2011 w2037 w2076 w2119 w2158 w2161 w2198 w2235 w2239 w2249 w2277 w2284 w2310 w2329 w2332 w2361 w2393 _]
      tunnel: [w1895 w1899 w1912 w1919 w1930 w1940 w1977 w2003 w2009 w2046 w2075 w2116 w2158 w2161 w2198 w2235 w2238 w2245 w2277 w2281 w2307 w2329 w2332 w2363 w2393 w2401] -> w1890
      tunnel: [FALSE ("UpdateMetadata") "EXIT" "diagPageVisible" "runtimeMenusVisible" "ARM" "QueryLoad" FALSE ("UpdateMetadata") FALSE ("UpdateMetadata") FALSE ("UpdateMetadata") FALSE ("UpdateMetadata") FALSE ("UpdateMetadata") FALSE ("UpdateMetadata") FALSE ("UpdateMetadata") FALSE ("UpdateMetadata") FALSE ("UpdateMetadata") FALSE ("UpdateMetadata") FALSE ("UpdateMetadata") FALSE ("UpdateMetadata") "Drag Corrected" FALSE ("UpdateMetadata") "PublishNewRecords" FALSE ("UpdateMetadata") FALSE ("UpdateMetadata") "RefreshMetadata" FALSE ("UpdateMetadata") FALSE ("UpdateMetadata")] -> w1889
      event Timeout {
        n1089 = event-data() -> ()  [unwired: 2 out]
        n1090 = Get Date/Time In Seconds() -> (seconds since 1Jan1904=w1897:timestamp)
        n1091 = Format Date/Time String(seconds (now)=w1897) -> (date/time string=→"TimeNow":string)  [unwired: 2 out]
      }
      event "EXIT": Value Change {
        n1092 = event-data() -> ()  [unwired: 2 out]
        n1093 = property on="Property Node" class="Application"(error in=errorcluster {"status"=FALSE, "code"=0, "source"=""} ("error in (no error)")) -> (error out=w1899:errorcluster, "Application:Kind"=w1904:T37)  [unwired: 1 in, 1 out]
        n1094 = Two Button Dialog(message="Exit BIMS Collector?\nAll Unsaved data will be lost.", 1:"NO" ("F button name (\"Cancel\")"), 2:"YES" ("T button name (\"OK\")")) -> (T button?=w1905:bool)
        n1095 = case shown="\"Development System\"" w1904 {
          tunnel: w1905 -> [w1906 w1907 w1908]
          frame Default {
            n1096 = Stop(stop? (T)=w1906) -> ()
          }
          frame "Development System" {
            n1097 = Stop(stop? (T)=w1907) -> ()
          }
          frame "Run Time System" {
            n1098 = Quit LabVIEW(quit? (T)=w1908) -> ()
          }
        }
      }
      event "diagPageVisible": Value Change {
        # "Toggles display of \"Internal Use\" tab for diagnostics purposes"
        # "Key navigation ONLY: Cntrl-Shift-F11"
        n1099 = event-data() -> ("NewVal"=w1915:bool)  [unwired: 1 out]
        n1100 = property on="aboutTabCntrl" class="TabCtl (strict)"(error in=errorcluster {"status"=FALSE, "code"=0, "source"=""} ("error in (no error)")) -> (error out=w1914:errorcluster, "Pages"=w1918:refnum<vi>[])  [unwired: 1 in, 1 out]
        n1101 = Index Array(array=w1918, index=1) -> (element=w1916:refnum<vi>)
        n1102 = property on="Property Node" class="Page"(reference=w1916, error in=w1914, "PageVis"=w1915) -> (error out=w1913:errorcluster)  [unwired: 1 out]
        n1103 = property on="diagPageVisible" class="Bool (strict)"(error in=w1913, "Value"=w1915) -> (error out=w1910:errorcluster)  [unwired: 1 in, 1 out]
        n1104 = call <vilib>:"General Error Handler.vi"("error in (no error)"=w1910) -> ()  [unwired: 2 in, 13 out]
      }
      event "runtimeMenusVisible": Value Change {
        # "Key navigation ONLY: Cntrl-Shift-F10"
        n1105 = event-data() -> ("NewVal"=w1924:bool)  [unwired: 1 out]
        n1106 = control-ref of="This VI"() -> (w1923:refnum<vi>)
        n1107 = property class="VI"(reference=w1923, error in=w1922, "Front Panel.ShowMenuBar"=w1924) -> (reference out=w1921:refnum<vi>, error out=w1920:errorcluster)
        n1108 = Close Reference(reference=w1921, error in (no error)=w1920) -> (error out=w1919:errorcluster)
      }
      event "ARM": Value Change {
        # "This section will arm the system"
        n1109 = event-data() -> ()  [unwired: 2 out]
        n1110 = disable-structure shown="Disabled" {
          frame Disabled {
            "DIO" <- u32 21 ("DIO")
          }
          frame Enabled {
          }
        }
        n1111 = Bundle By Name(cluster=cluster{"ARMED":bool} {"ARMED"=FALSE} ("Safety_Interlock"), "ARMED"=TRUE) -> (→"SafetyInterlock":cluster{"ARMED":bool})
        n1112 = local write "SUBMIT DATE/TIME"("" ("Empty String Constant")) -> ()
        n1113 = local read "MeasSrc"() -> (w1932:T6)
        n1114 = case shown="\"Screens\"" w1932 {
          tunnel: w1931 -> [w1935 w1936 w1938]
          tunnel: [w1935 w1936 w1938] -> w1930
          frame "Simulated", Default {
          }
          frame "Radar" {
          }
          frame "Screens" {
            n1115 = local write "readyClock"(TRUE ("readyClock")) -> ()
          }
        }
      }
      event "QueryLoad": Value Change {
        w1946 = "%x" ("time format string (%c)")
        w1962 = "" ("replace string (\"\")")
        # "This section plots  Impact velocity vs. loadingdata"
        n1116 = event-data() -> ()  [unwired: 2 out]
        n1117 = Format Date/Time String(time format string (%c)=w1946, seconds (now)="lkupStartDate") -> (date/time string=w1945:string)  [unwired: 1 out]
        n1118 = Format Date/Time String(time format string (%c)=w1946, seconds (now)="lkupEndDate") -> (date/time string=w1944:string)  [unwired: 1 out]
        n1119 = call "Trim String.vi"("inStr"="Powder.freeTxt") -> ("outStr"=w1960:string)
        n1120 = call "Trim String.vi"("inStr"="Threat.freeTxt") -> ("outStr"=w1961:string)
        n1121 = invoke on="v50_table" class="Tbl" method="Reinit To Default"(error in=w1941) -> (error out=w1953:errorcluster)  [unwired: 2 in, 2 out]
        n1122 = invoke on="Vel.vs.Loading" class="WFGraph (strict)" method="Reinit To Default"(error in=w1953) -> (error out=w1948:errorcluster)  [unwired: 2 in, 2 out]
        n1123 = Format Into String(format string="SELECT TOP %d dbsrc.experiment.threat, dbsrc.shots.loading, dbsrc.shots.impact, dbsrc.experiment.powder, dbsrc.shots.date from dbsrc.shots, dbsrc.experiment where dbsrc.shots.expt = dbsrc.experiment.expt and dbsrc.shots.loading > 0 and dbsrc.shots.date between '%s' and '%s' and dbsrc.shots.impact between 10 and 5000 and dbsrc.experiment.powder like '%%%s%%' and dbsrc.experiment.threat like '%%%s%%' and experiment.threat<>'' order by dbsrc.experiment.threat, dbsrc.shots.loading, dbsrc.shots.impact;" ("Format String"), error in=w1948, "maxRecs", w1945, w1944, w1960, w1961) -> (resulting string=w1966:string, error out=w1951:errorcluster)  [unwired: 1 in]
        n1124 = Search and Replace String(input string=w1966, search string=" and experiment.powder like '%%'", replace string=w1962, error in=w1951) -> (result string=w1964:string, error out=w1952:errorcluster)  [unwired: 6 out]
        n1125 = Search and Replace String(input string=w1964, search string="and experiment.threat like '%%'", replace string=w1962, error in=w1952) -> (result string=w1955:string, error out=w1950:errorcluster)  [unwired: 6 out]
        n1126 = call "Fetch Data (SubVI).vi"("error IN"=w1950, "query string"=w1955) -> ("error OUT"=w1940:errorcluster, "recordset data"=w1956:string[][])  [unwired: 4 out]
        "v50_table" <- w1956
        n1127 = Fract/Exp String To Number(string=w1956) -> (number=w1970:dbl[][])  [unwired: 4 out]
        n1128 = Array Size(array=w1956) -> (size(s)=w1958:i32[])
        n1129 = Index Array(array=w1958) -> (element=→"ActualNumRecs":i32)  [unwired: 1 in]
        n1130 = Index Array(array=w1970, index (col)=2 ("Disabled Index (col)")) -> (element=w1969:dbl[])  [unwired: 1 in]
        n1131 = Index Array(array=w1970, index (col)=1 ("Disabled Index (col)")) -> (element=w1968:dbl[])  [unwired: 1 in]
        n1132 = Bundle(w1968, w1969) -> (→"Vel.vs.Loading":cluster{dbl[], dbl[]})  [unwired: 1 out]
      }
      event "ThreatGroups": Value Change {
        n1133 = event-data() -> ()  [unwired: 2 out]
        n1134 = control-ref of="ThreatGroups"() -> (w1979:refnum<vi>)
        n1135 = property on="Property Node" class="Ring (strict)"(reference=w1979, error in=w1978) -> (error out=w1976:errorcluster, "RingText.Text"=w1974:string)  [unwired: 1 out]
        n1136 = Not Equal?(x=w1974, y="") -> (x != y?=w1973:bool)
        n1137 = case shown="True" w1973 {
          tunnel: w1974 -> [_ w1989]
          tunnel: [w1981 w1987] -> w1977
          tunnel: w1976 -> [w1984 w1986]
          frame False {
            n1138 = property on="ThreatDetails" class="Ring (strict)"(error in=w1984, "Strings []"=string[] [], "Value"=u16 0 ("Value (Signaling)")) -> (error out=w1982:errorcluster)  [unwired: 1 in, 1 out]
            n1139 = invoke on="threatDetails" class="Clust (strict)" method="Reinit To Default"(error in=w1982) -> (error out=w1981:errorcluster)  [unwired: 2 in, 2 out]
          }
          frame True {
            n1140 = call "Select Threat Details.vi"("threatGroup"=w1989) -> ("threatDetails"=w1988:string[])  [unwired: 1 out]
            n1141 = property on="ThreatDetails" class="Ring (strict)"(error in=w1986, "Strings []"=w1988, "Val(Sgnl)"=u16 0 ("Value (Signaling)")) -> (error out=w1987:errorcluster)  [unwired: 1 in, 1 out]
          }
        }
      }
      event "panelSearch": Value Change {
        # "This section returns past panels"
        n1142 = event-data() -> ()  [unwired: 2 out]
        n1143 = control-ref of="pastPanels"() -> (w2006:refnum<vi>)
        n1144 = control-ref of="Mfr_0"() -> (w2000:refnum<vi>)
        n1145 = control-ref of="SampleStyle_0"() -> (w2001:refnum<vi>)
        n1146 = control-ref of="Requestors_0"() -> (w1999:refnum<vi>)
        n1147 = control-ref of="ThreatSize_0"() -> (w1998:refnum<vi>)
        n1148 = call "queryPanels (SubVI).vi"("ThreatSize_0"=w1998, "Mfr_0"=w2000, "Requestors_0"=w1999, "Style_0"=w2001, "error in"=w2004, "srchParams"="srchParams", "pastPanels"=w2006) -> ("error out"=w2003:errorcluster, "recordset data"=w1997:string[][], "actualNumPanels"=→"actualNumPanels":i32)  [unwired: 2 in]
        "pastPanels" <- w1997
        n1149 = Index Array(array=w1997) -> (element=w1991:string[])  [unwired: 2 in]
        n1150 = Array Size(array=w1991) -> (size(s)=w1996:i32)
        n1151 = Greater Than 0?(x=w1996) -> (x > 0?=w1995:bool)
        n1152 = Select(t=T14."Enabled" ("Disabled"), s=w1995, f=T14."Disabled and Grayed Out" ("Disabled")) -> (s? t:f=w1994:T14)
        n1153 = property on="reportV50_History" class="Bool"("DisabledEnum"=w1994) -> ()  [unwired: 2 in, 2 out]
      }
      event "pastPanels": Mouse Up {
        n1154 = event-data() -> ("CtlRef"=w2019:refnum<vi>)  [unwired: 1 out]
        n1155 = property on="Property Node" class="Tbl (strict)"(reference=w2019, error in=w2011) -> (error out=w2010:errorcluster, "Value"=w2018:string[][], "EditPos"=w2017:T38)  [unwired: 1 out]
        n1156 = Unbundle By Name(w2017) -> ("Row"=w2016:i32)
        n1157 = Index Array(array=w2018, index (row)=w2016, index (col)=0 ("disabled index (col)")) -> (element=w2015:string)
        n1158 = Scan From String(input string=w2015, error in=w2010, default 1=1 ("Record #")) -> (error out=w2009:errorcluster, output 1=w2013:i32)  [unwired: 2 in, 2 out]
        n1159 = local write "Record #"(w2013) -> ()
      }
      event "ThreatDetails", "SampleID": Value Change {
        # "A Sample ID is entered"
        # "A range is selected"
        # "A measurement requires the selection of a threat,\nso delay enabling the \"Measure\" tab until a grain wt\nis chosen."
        n1160 = event-data() -> ()  [unwired: 2 out]
        n1161 = control-ref of="ThreatGroups"() -> (w2038:refnum<vi>)
        n1162 = control-ref of="ThreatDetails"() -> (w2035:refnum<vi>)
        n1163 = call "Get Projectile Atributes from ThreatGroupDetail.vi"("error IN"=w2037, "ThreatDetail"=w2035, "ThreatGroup"=w2038) -> ("error out"=w2036:errorcluster, "projectileAttribs"=w2034:T39)  [unwired: 1 out]
        "threatDetails" <- w2034
        n1164 = Unbundle By Name(w2034) -> ("grainSize"=w2027:string)
        n1165 = Equal?(x=w2027, y="") -> (x = y?=w2028:bool)
        n1166 = case shown="False" w2028 {
          tunnel: w2027 -> [w2056 _]
          tunnel: [w2055 u16 0 ("GrainSize")] -> w2033
          frame False {
            # "A grain size is selected"
            n1167 = Scan From String(input string=w2056) -> (output 1=w2055:u16)  [unwired: 3 in, 4 out]
            "GrainSize" <- w2055
          }
          frame True {
            # "A grain size not selected"
          }
        }
        n1168 = Equal?(x=w2027, y="") -> (x = y?=w2053:bool)
        n1169 = local read "rangeSetup"() -> (w2050:u16)
        n1170 = case shown="False" w2053 {
          tunnel: [w2060 sgl 0.0] -> w2049
          tunnel: w2027 -> [w2058 _]
          frame False {
            w2062 = sgl 0.0  # sgl
            n1171 = Scan From String(format string="%f " ("Format String"), input string=w2058, default 1=w2062) -> (output 1=w2061:sgl)  [unwired: 2 in, 3 out]
            n1172 = disable-structure shown="Enabled" {
              disable-tunnel: w2061 -> [w2065 w2066]
              disable-tunnel: [w2064 w2066] -> w2060
              frame Disabled {
                n1173 = Multiply(x=sgl 0.06479891, y=w2065) -> (x*y=w2064:sgl)
              }
              frame Enabled {
              }
            }
          }
          frame True {
          }
        }
        "Projectile Mass" <- w2049
        n1174 = local read "SampleID"() -> (w2032:string)
        n1175 = Greater Than 0?(x=w2050) -> (x > 0?=w2051:bool)
        n1176 = Greater Than 0?(x=w2033) -> (x > 0?=w2052:bool)
        n1177 = Not Equal?(x=w2032, y="") -> (x != y?=w2030:bool)
        n1178 = Compound Arithmetic op=AND(w2052, w2051, w2030) -> (w2025:bool)
        n1179 = property on="mainTabCntrl" class="TabCtl (strict)"(error in=w2036) -> (error out=w2042:errorcluster, "Pages"=w2045:refnum<vi>[])  [unwired: 1 in, 1 out]
        n1180 = Not(x=w2025) -> (.not. x?=w2041:bool)
        n1181 = Index Array(array=w2045, index=1) -> (element=w2043:refnum<vi>)
        n1182 = Select(t=T15."Page Enabled" ("Page Enabled State"), s=w2025, f=T15."Page Disabled & Grayed" ("Page Enabled State")) -> (s? t:f=w2024:T15)
        n1183 = property on="Property Node" class="Page"(reference=w2043, error in=w2042, "PageEnb"=w2024) -> (error out=w2040:errorcluster)  [unwired: 1 out]
        n1184 = Select(t=T14."Enabled" ("Disabled"), s=w2025, f=T14."Disabled and Grayed Out" ("Disabled")) -> (s? t:f=w2022:T14)
        n1185 = property on="ARM" class="Bool"(error in=w2040, "Disabled"=w2022) -> (error out=w2048:errorcluster)  [unwired: 1 in, 1 out]
        n1186 = property on="addShot" class="Bool"(error in=w2048, "Disabled"=w2022) -> (error out=w2047:errorcluster)  [unwired: 1 in, 1 out]
        n1187 = property on="instruct_addShot" class="Str"(error in=w2047, "Visible"=w2041) -> (error out=w2046:errorcluster)  [unwired: 1 in, 1 out]
      }
      event "Mfr_1", "Mfr_2", "Mfr_3", "Mfr_4", "Mfr_5", "Mfr_6", "Mfr_0": Value Change {
        n1188 = event-data() -> ("CtlRef"=w2084:refnum<vi>)  [unwired: 1 out]
        n1189 = property on="Property Node" class="Ring (strict)"(reference=w2084, error in=w2076) -> (error out=w2074:errorcluster, "Label.Text"=w2080:string, "RingText.Text"=w2081:string)  [unwired: 1 out]
        n1190 = flat-sequence {
          tunnel: ["Mfr_1"] -> _
          tunnel: ["Mfr_2"] -> _
          tunnel: ["Mfr_3"] -> _
          tunnel: ["Mfr_4"] -> _
          tunnel: ["Mfr_5"] -> _
          tunnel: ["Mfr_6"] -> _
          frame #0 {
          }
        }
        n1191 = call "Select Sample Style.vi"("error IN"=w2074, "Mfr"=w2081) -> ("error Out"=w2073:errorcluster, "SampleStyles"=w2069:string[])  [unwired: 4 out]
        n1192 = Scan From String(format string="Mfr_%d", input string=w2080, error in=w2073, default 1=0 ("Mfr#")) -> (error out=w2070:errorcluster, output 1=w2079:i32)  [unwired: 1 in, 2 out]
        n1193 = case shown="1" w2079 {
          tunnel: [w2096 w2099 w2102 w2105 w2108 w2111 w2114] -> w2078
          tunnel: [w2095 w2098 w2101 w2104 w2107 w2110 w2113] -> w2071
          tunnel: w2070 -> [w2095 w2098 w2101 w2104 w2107 w2110 w2113]
          tunnel: w2069 -> [w2094 w2097 w2100 w2103 w2106 w2109 w2112]
          tunnel: [w2093 w2097 w2100 w2103 w2106 w2109 w2112] -> w2068
          frame 0, Default {
            n1194 = Delete From Array(array=w2094, length=1, index=0) -> (array with subset deleted=w2093:string[])  [unwired: 1 out]
            n1195 = control-ref of="SampleStyle_0"() -> (w2096:refnum<vi>)
          }
          frame 1 {
            n1196 = control-ref of="SampleStyle_1"() -> (w2099:refnum<vi>)
          }
          frame 2 {
            n1197 = control-ref of="SampleStyle_2"() -> (w2102:refnum<vi>)
          }
          frame 3 {
            n1198 = control-ref of="SampleStyle_3"() -> (w2105:refnum<vi>)
          }
          frame 4 {
            n1199 = control-ref of="SampleStyle_4"() -> (w2108:refnum<vi>)
          }
          frame 5 {
            n1200 = control-ref of="SampleStyle_5"() -> (w2111:refnum<vi>)
          }
          frame 6 {
            n1201 = control-ref of="SampleStyle_6"() -> (w2114:refnum<vi>)
          }
        }
        n1202 = property on="Property Node" class="Ring (strict)"(reference=w2078, error in=w2071, "Strings []"=w2068, "Val(Sgnl)"=u16 0 ("Value (Signaling)")) -> (error out=w2075:errorcluster)  [unwired: 1 out]
      }
      event "SampleStyle_1", "SampleStyle_2", "SampleStyle_3", "SampleStyle_4", "SampleStyle_5", "SampleStyle_6", "SampleStyle_0": Value Change {
        n1203 = event-data() -> ("CtlRef"=w2125:refnum<vi>)  [unwired: 1 out]
        n1204 = call "Get Sample Style Atributes.vi"("StyleNumRef"=w2125) -> ("SampleSpecs"=w2120:T40)  [unwired: 1 in]
        n1205 = flat-sequence {
          tunnel: ["SampleStyle_1"] -> _
          tunnel: ["SampleStyle_2"] -> _
          tunnel: ["SampleStyle_3"] -> _
          tunnel: ["SampleStyle_4"] -> _
          tunnel: ["SampleStyle_5"] -> _
          tunnel: ["SampleStyle_6"] -> _
          frame #0 {
          }
        }
        n1206 = property on="Property Node" class="Ring (strict)"(reference=w2125, error in=w2119) -> (error out=w2118:errorcluster, "Label.Text"=w2124:string)  [unwired: 1 out]
        n1207 = Scan From String(format string="SampleStyle_%d", input string=w2124, error in=w2118, default 1=0 ("default value 1")) -> (error out=w2117:errorcluster, output 1=w2122:i32)  [unwired: 1 in, 2 out]
        n1208 = case shown="0, Default" w2122 {
          tunnel: w2120 -> [w2134 w2137 w2140 w2143 w2146 w2149 w2152]
          tunnel: w2117 -> [w2133 w2136 w2139 w2142 w2145 w2148 w2151]
          tunnel: [w2132 w2135 w2138 w2141 w2144 w2147 w2150] -> w2116
          frame 0, Default {
            n1209 = property on="SampleAttribs_0" class="Clust (strict)"(error in=w2133, "Val(Sgnl)"=w2134) -> (error out=w2132:errorcluster)  [unwired: 1 in, 1 out]
            "SampleAttribs_0" <- w2134
          }
          frame 1 {
            n1210 = property on="SampleAttribs_1" class="Clust (strict)"(error in=w2136, "Val(Sgnl)"=w2137) -> (error out=w2135:errorcluster)  [unwired: 1 in, 1 out]
            "SampleAttribs_1" <- w2137
          }
          frame 2 {
            n1211 = property on="SampleAttribs_2" class="Clust (strict)"(error in=w2139, "Val(Sgnl)"=w2140) -> (error out=w2138:errorcluster)  [unwired: 1 in, 1 out]
            "SampleAttribs_2" <- w2140
          }
          frame 3 {
            n1212 = property on="SampleAttribs_3" class="Clust (strict)"(error in=w2142, "Val(Sgnl)"=w2143) -> (error out=w2141:errorcluster)  [unwired: 1 in, 1 out]
            "SampleAttribs_3" <- w2143
          }
          frame 4 {
            n1213 = property on="SampleAttribs_4" class="Clust (strict)"(error in=w2145, "Val(Sgnl)"=w2146) -> (error out=w2144:errorcluster)  [unwired: 1 in, 1 out]
            "SampleAttribs_4" <- w2146
          }
          frame 5 {
            n1214 = property on="SampleAttribs_5" class="Clust (strict)"(error in=w2148, "Val(Sgnl)"=w2149) -> (error out=w2147:errorcluster)  [unwired: 1 in, 1 out]
            "SampleAttribs_5" <- w2149
          }
          frame 6 {
            n1215 = property on="SampleAttribs_6" class="Clust (strict)"(error in=w2151, "Val(Sgnl)"=w2152) -> (error out=w2150:errorcluster)  [unwired: 1 in, 1 out]
            "SampleAttribs_6" <- w2152
          }
        }
      }
      event "SHOTS", "Sort by AVG": Value Change {
        n1216 = event-data() -> ()  [unwired: 2 out]
        n1217 = local read "Site"() -> (w2153:string)
        n1218 = local read "SHOTS"() -> (w2155:T7[])
        n1219 = call "Update Shot Table (DKC).vi"("Sort by AVG"="Sort by AVG", "Site"=w2153, "shot array"=w2155) -> ("shotTable OUT"=→"Table of Shots":string[][])
      }
      event "Layer_1.plyNum", "Layer_2.plyNum", "Layer_3.plyNum", "Layer_4.plyNum", "Layer_5.plyNum", "Layer_6.plyNum", "SampleAttribs_1.ozPerYd2", "SampleAttribs_2.ozPerYd2", "SampleAttribs_3.ozPerYd2", "SampleAttribs_4.ozPerYd2", "SampleAttribs_5.ozPerYd2", "SampleAttribs_6.ozPerYd2": Value Change {
        n1220 = event-data() -> ()  [unwired: 2 out]
        n1221 = global read "BIMS_Collector Globals.vi" "SampleAttribs"() -> (w2159:T23)
        n1222 = Build Array("Layer_1", "Layer_2", "Layer_3", "Layer_4", "Layer_5", "Layer_6") -> (w2162:T41)
        n1223 = global write "BIMS_Collector Globals.vi" "LayerSpecs"(w2162) -> ()
        n1224 = for {
          tunnel: w2162 -> [w2189] mode=indexing
          shift-right: [w2191] -> w2170
          shift-left: 0 -> [w2190]
          tunnel: [w2188] -> w2180 mode=indexing
          tunnel: w2159 -> [w2186] mode=indexing
          n1225 = Unbundle By Name(w2186) -> ("ozPerYd2"=w2182:string)
          n1226 = Equal?(x=w2182, y="" ("Empty String Constant")) -> (x = y?=w2181:bool)
          n1227 = case shown="False" w2181 {
            tunnel: [w2195 sgl 0.0 ("default value 1")] -> w2185
            tunnel: w2182 -> [w2192 _]
            frame False {
              n1228 = Scan From String(format string="%f", input string=w2192, default 1=sgl 0.0 ("default value 1")) -> (output 1=w2195:sgl)  [unwired: 2 in, 3 out]
            }
            frame True {
            }
          }
          n1229 = Unbundle By Name(w2189) -> ("plyNum"=w2187:i32)
          n1230 = Add(x=w2190, y=w2187) -> (x+y=w2191:i32)
          n1231 = To Single Precision Float(number=w2187) -> (single precision float=w2184:sgl)
          n1232 = Multiply(x=w2184, y=w2185) -> (x*y=w2188:sgl)
        }
        "totalNumLayers" <- w2170
        n1233 = Divide(x=w2180, y=sgl 144.0) -> (x/y=w2178:sgl[])
        n1234 = Index Array(array=w2178) -> (element #1=→"fab1_totalWt":sgl, element #2=→"fab2_totalWt":sgl, element #3=→"fab3_totalWt":sgl, element #4=→"fab4_totalWt":sgl, element #5=→"fab5_totalWt":sgl, element #6=→"fab6_totalWt":sgl)  [unwired: 6 in]
        n1235 = Add Array Elements(numeric array=w2178) -> (sum=→"totalBAW":sgl)
      }
      event "clayCalArray": Value Change {
        n1236 = event-data() -> ()  [unwired: 2 out]
        n1237 = for {
          tunnel: "clayCalArray" -> [w2224] mode=indexing
          shift-right: [w2223] -> w2206
          shift-left: "" ("Empty String Constant") -> [w2221]
          shift-right: [w2218] -> w2202
          shift-left: i16[] [] -> [w2217]
          n1238 = Greater Than 0?(x=w2224) -> (x > 0?=w2225:bool)
          n1239 = case shown="False" w2225 {
            tunnel: w2224 -> [_ w2231]
            tunnel: ["##" ("clayCalib") w2233] -> w2222
            tunnel: w2221 -> [w2228 w2232]
            tunnel: [w2228 w2232] -> w2220
            tunnel: [w2226 w2230] -> w2218
            tunnel: w2217 -> [w2226 w2229]
            frame False {
            }
            frame True {
              n1240 = Format Into String(w2231) -> (resulting string=w2233:string)  [unwired: 3 in, 1 out]
              n1241 = Build Array (concatenate)(w2229, w2231) -> (w2230:i16[])
            }
          }
          n1242 = Concatenate Strings(w2220, w2222, "-" ("string")) -> (w2223:string)
        }
        n1243 = String Length(string=w2206) -> (length=w2207:i32)
        n1244 = Add Array Elements(numeric array=w2202) -> (sum=w2211:i16)
        n1245 = Array Size(array=w2202) -> (size(s)=w2212:i32)
        n1246 = Decrement(x=w2207) -> (x-1=w2204:i32)
        n1247 = To Single Precision Float(number=w2211) -> (single precision float=w2210:sgl)
        n1248 = To Single Precision Float(number=w2212) -> (single precision float=w2200:sgl)
        n1249 = String Subset(string=w2206, length (rest)=w2204) -> (substring=w2205:string)  [unwired: 1 out]
        n1250 = Equal To 0?(x=w2200) -> (x = 0?=w2199:bool)
        n1251 = local write "clayCalib"(w2205) -> ()
        n1252 = case shown="True" w2199 {
          tunnel: w2210 -> [w2215 w2216]
          tunnel: w2200 -> [w2214 _]
          tunnel: [w2213 w2216] -> w2209
          frame False {
            n1253 = Divide(x=w2215, y=w2214) -> (x/y=w2213:sgl)
          }
          frame True {
          }
        }
        "clayAverage" <- w2209
      }
      event "reportV50_History": Value Change {
        n1254 = event-data() -> ()  [unwired: 2 out]
        n1255 = local write "lookupRec"(TRUE ("lookupRec")) -> ()
      }
      event "Methods": Value Change {
        n1256 = event-data() -> ("CtlRef"=w2243:refnum<vi>)  [unwired: 1 out]
        n1257 = call "Dropdown Selection (SubVI).vi"("reference"=w2243) -> ("element"=w2242:string)
        n1258 = Equal?(x=w2242, y="V50") -> (x = y?=w2240:bool)
        n1259 = property on="minV50" class="DigNum (strict)"(error in=w2239, "Visible"=w2240) -> (error out=w2238:errorcluster)  [unwired: 1 in, 1 out]
      }
      event "rangeSetup": Value Change {
        n1260 = event-data() -> ("NewVal"=w2253:u16)  [unwired: 1 out]
        n1261 = case shown="2" w2253 {
          tunnel: ["0" ("section") "5.0" ("section") "7.5" ("section") "45.0" ("section")] -> w2259
          frame 0, Default {
          }
          frame 1 {
          }
          frame 2 {
          }
          frame 3 {
          }
        }
        n1262 = local read "configPath"() -> (w2261:path)
        n1263 = local read "GrainSize"() -> (w2252:u16)
        n1264 = Greater Than 0?(x=w2253) -> (x > 0?=w2256:bool)
        n1265 = Greater Than 0?(x=w2252) -> (x > 0?=w2254:bool)
        n1266 = call <vilib>:"Open Config Data (compatibility).vi"("error in (no error)"=w2249, "configuration file path"=w2261) -> ("error out"=w2269:errorcluster, "refnum"=w2271:T35)  [unwired: 7 in, 1 out]
        n1267 = And(x=w2256, y=w2254) -> (x .and. y?=w2255:bool)
        n1268 = call-poly <vilib>:"Write Key.vi"("write raw string? (F)"=TRUE, "section"="Ballistic Parameters", "error in (no error)"=w2269, "value"=w2259, "key"="MidPoint To Target Distance", "refnum"=w2271) -> ("error out"=w2268:errorcluster, "refnum out"=w2267:T35)  [unwired: 4 out]
        n1269 = call <vilib>:"Close Config Data.vi"("error in (no error)"=w2268, "refnum"=w2267) -> ("error out"=w2260:errorcluster)  [unwired: 1 in, 8 out]
        n1270 = Not(x=w2255) -> (.not. x?=w2265:bool)
        n1271 = Select(t=u8 0 ("y"), s=w2255, f=u8 2 ("y")) -> (s? t:f=w2251:u8)
        n1272 = Scan From String(input string=w2259, error in=w2260, default 1=sgl 0.0 ("default value 1")) -> (error out=w2248:errorcluster, output 1=w2258:sgl)  [unwired: 2 in, 2 out]
        n1273 = local write "mid_to_targ_dist"(w2258) -> ()
        n1274 = property on="ARM" class="Bool"(error in=w2248, "Disabled"=w2251) -> (error out=w2247:errorcluster)  [unwired: 1 in, 1 out]
        n1275 = property on="addShot" class="Bool"(error in=w2247, "Disabled"=w2251) -> (error out=w2246:errorcluster)  [unwired: 1 in, 1 out]
        n1276 = property on="instruct_addShot" class="Str"(error in=w2246, "Visible"=w2265) -> (error out=w2245:errorcluster)  [unwired: 1 in, 1 out]
        "instruct_addShot" <- "RANGE SETUP and THREAT must be selected before shots can be added." ("instruct_addShot")
      }
      event "Drag Corrected", "maxDev": Value Change {
        n1277 = event-data() -> ()  [unwired: 2 out]
        n1278 = local write "processShots"(TRUE ("ProcessShots")) -> ()
      }
      event "MC Listbox of Shots": Mouse Up {
        n1279 = event-data() -> ()  [unwired: 2 out]
        n1280 = flat-sequence {
          tunnel: w2284 -> [w2288]
          tunnel: [w2286] -> w2283
          tunnel: ["MC Listbox of Shots"] -> w2280
          tunnel: w2283 -> [w2292]
          tunnel: [w2291] -> w2282
          tunnel: w2280 -> [_]
          tunnel: w2282 -> [w2297]
          tunnel: [w2295] -> w2281
          frame #0 {
            n1281 = property on="Table of Shots" class="Tbl (strict)"(error in=w2288) -> (error out=w2287:errorcluster, "Value"=w2289:string[][])  [unwired: 1 in, 1 out]
            n1282 = local write "STOP (Shots MC LB)"(FALSE ("STOP (Shots MC LB)")) -> ()
            n1283 = property on="MC Listbox of Shots" class="MCListbox (strict)"(error in=w2287, "ItemNames"=w2289) -> (error out=w2286:errorcluster)  [unwired: 1 in, 1 out]
          }
          frame #1 {
            n1284 = control-ref of="MC Listbox of Shots"() -> (w2294:refnum<vi>)
            n1285 = control-ref of="STOP (Shots MC LB)"() -> (w2293:refnum<vi>)
            n1286 = call "multicolumn listbox sort.vi"("error IN"=w2292, "Bool Refnum"=w2293, "MCListbox Refnum"=w2294) -> ("error out"=w2291:errorcluster)  [unwired: 4 in]
          }
          frame #2 {
            n1287 = property on="MC Listbox of Shots" class="MCListbox (strict)"(error in=w2297) -> (error out=w2296:errorcluster, "ItemNames"=w2298:string[][])  [unwired: 1 in, 1 out]
            n1288 = property on="Table of Shots" class="Tbl (strict)"(error in=w2296, "Val(Sgnl)"=w2298) -> (error out=w2295:errorcluster)  [unwired: 1 in, 1 out]
          }
        }
      }
      event "PublishNewRecords": Value Change {
        w2304 = "\\" ("string")
        w2315 = TRUE  # overwrite (F)
        # "2. INSERT new records to Experiments and  \n      Shots tables in local Export.mdb file."
        # "1. SELECT new records from local MDB \n     by comparing against last record numbers \n     found in IMPORT table on BIMS server."
        # "Pushes latest ballistics performance data up to BIMS Server\n\n - Attempts connection with server (reports connection success in msgbox)\n - If successful:\n   - Exports all experiment/shot records since last table marker to [site].mdb file\n   - Sends export.mdb file to drop location on BIMS File Server\n   - Executes SSIS package to import records from export.mdb file\n - Otherwise provides option to try again or cancel"
        # "3. Copy Export.mdb file to [sitename].mdb in [sitename] \n      FileDrop folder on BIMS server."
        n1289 = event-data() -> ()  [unwired: 2 out]
        n1290 = property on="Loading" class="Ring (strict)"(error in=w2310, "Visible"=TRUE) -> (error out=w2309:errorcluster)  [unwired: 1 in, 1 out]
        n1291 = local read "Site"() -> (w2299:string)
        n1292 = call "Export New Records.vi"("error IN"=w2309, "Site"=w2299) -> ("error out"=w2317:errorcluster)  [unwired: 3 in, 6 out]
        n1293 = Concatenate Strings("\\\\" ("string"), "Server", w2304, "Folder", w2304, w2299, ".mdb" ("string")) -> (w2300:string)
        n1294 = String To Path(string=w2300) -> (path=w2313:path)
        n1295 = Copy(8:w2317, 9:w2315, 10:w2313, 11:path "C:/Ballistics/Export.mdb" ("source path")) -> (0:w2314:errorcluster)  [unwired: 3 out]
        n1296 = case shown="No Error" w2314 {
          selector: w2314 -> [w2319 w2321]
          tunnel: [w2319 w2320] -> w2308
          frame No Error {
            n1297 = One Button Dialog(message="New sample performance records submitted \nto BIMS Warehouse successfully.\n\nPublishing will occur in under five minutes.") -> ()  [unwired: 2 out]
          }
          frame Error {
            n1298 = call <vilib>:"General Error Handler.vi"("error in (no error)"=w2321) -> ("error out"=w2320:errorcluster)  [unwired: 2 in, 12 out]
          }
        }
        n1299 = property on="Loading" class="Ring (strict)"(error in=w2308, "Visible"=FALSE) -> (error out=w2307:errorcluster)  [unwired: 1 in, 1 out]
      }
      event "arrIDC": Mouse Up {
        n1300 = event-data() -> ()  [unwired: 2 out]
        "velProfile" <- cluster{dbl, dbl}[] [] ("velProfile")
        "arrIDC" <- dbl[] [] ("arrIDC")
        "relativeTime" <- cluster{"ts2":dbl, "ts3":dbl, "ts1":dbl} {"ts2"=0.0, "ts3"=0.0, "ts1"=0.0} ("relativeTime")
        "velMeasProf" <- T8 {"v2"=0.0, "vB"=0.0, "vOuter"=0.0, "v1"=0.0, "vA"=0.0, "vInner"=0.0} ("velMeasProf")
        "velCompProf" <- cluster{"vStrike":dbl, "vA":dbl} {"vStrike"=0.0, "vA"=0.0} ("velCompProf")
        "displacement" <- T9 {"ds_v2"=6.75, "ds2"=5.0833, "ds_vB"=4.9167, "ds3"=4.75, "ds_vAvg"=6.9167, "ds_v1"=7.0833, "ds1"=8.75, "ds_vA"=8.9167, "ds0"=9.0833} ("displacement")
      }
      event "SampleBackings": Value Change {
        # "Clay is the default sample backing material.\n\n  If another selection is made, then grey out and disable all controls relating to clay."
        n1301 = event-data() -> ()  [unwired: 2 out]
        n1302 = case shown="0, Default" "SampleBackings" {
          tunnel: [T14."Disabled and Grayed Out" ("Disabled") T14."Enabled" ("Disabled") T14."Disabled and Grayed Out" ("Disabled")] -> w2330
          frame 0, Default {
          }
          frame 1 {
          }
          frame 2.. {
          }
        }
        n1303 = property on="clayCalArray" class="Arr (strict)"("DisabledEnum"=w2330) -> ()  [unwired: 2 in, 2 out]
        n1304 = property on="clayAverage" class="DigNum (strict)"("DisabledEnum"=w2330) -> ()  [unwired: 2 in, 2 out]
        n1305 = property on="clayTemp" class="DigNum (strict)"("DisabledEnum"=w2330) -> ()  [unwired: 2 in, 2 out]
      }
      event "RefreshMetadata": Value Change {
        # "Pulls latest metadata down from BIMS Database Server\n - Attempts connection with server \n        (reports failure if connection is unsuccessful)\n - If successful:\n   - Updates local database records from server\n   - Updates dropdown listboxes from local database"
        n1306 = event-data() -> ()  [unwired: 2 out]
        n1307 = property on="Loading" class="Ring (strict)"(error in=w2361, "Visible"=TRUE) -> (error out=w2360:errorcluster)  [unwired: 1 in, 1 out]
        n1308 = control-ref of="LayerStitchTypes"() -> (w2345:refnum<vi>)
        n1309 = control-ref of="BackLayer"() -> (w2356:refnum<vi>)
        n1310 = control-ref of="FrontLayer"() -> (w2357:refnum<vi>)
        n1311 = control-ref of="ThreatGroups"() -> (w2358:refnum<vi>)
        n1312 = control-ref of="SampleClamping"() -> (w2366:refnum<vi>)
        n1313 = control-ref of="SampleTypes"() -> (w2383:refnum<vi>)
        n1314 = control-ref of="SampleDimensions"() -> (w2382:refnum<vi>)
        n1315 = control-ref of="ModelMfrs"() -> (w2381:refnum<vi>)
        n1316 = control-ref of="Assemblers"() -> (w2380:refnum<vi>)
        n1317 = control-ref of="Submitters"() -> (w2379:refnum<vi>)
        n1318 = control-ref of="SampleCoverings"() -> (w2337:refnum<vi>)
        n1319 = control-ref of="PowderTypes"() -> (w2378:refnum<vi>)
        n1320 = control-ref of="Methods"() -> (w2375:refnum<vi>)
        n1321 = control-ref of="TestConditions"() -> (w2374:refnum<vi>)
        n1322 = control-ref of="SampleBackings"() -> (w2373:refnum<vi>)
        n1323 = control-ref of="Ballisticians"() -> (w2372:refnum<vi>)
        n1324 = control-ref of="Shooters"() -> (w2371:refnum<vi>)
        n1325 = control-ref of="Recorders"() -> (w2370:refnum<vi>)
        n1326 = Build Array(w2345, w2356, w2357, w2358, w2366, w2383, w2382, w2381, w2380, w2379, w2337, w2378, w2375, w2374, w2373, w2372, w2371, w2370) -> (w2377:refnum<vi>[])
        n1327 = call "Update Metadata using listbox names.vi"("error in"=w2360, "Site"="Site", "RefNumArrIn"=w2377) -> ("error out"=w2384:errorcluster, "RefNumArrOut"=w2376:refnum<vi>[])  [unwired: 1 in, 6 out]
        n1328 = call "Fill Lists from DB (1st Pass).vi"("error in"=w2384, "RefNumArray"=w2376) -> ("error out"=w2346:errorcluster)  [unwired: 1 in, 4 out]
        n1329 = call "Fill Stitch Lists.vi"("error IN"=w2346) -> ("error OUT"=w2341:errorcluster)  [unwired: 6 in]
        n1330 = control-ref of="ThreatSize_0"() -> (w2339:refnum<vi>)
        n1331 = control-ref of="Requestors_0"() -> (w2344:refnum<vi>)
        n1332 = Build Array(w2339, w2344) -> (w2343:refnum<vi>[])
        n1333 = call "Fill Lists from DB (2nd Pass).vi"("errorIN"=w2341, "colNames"=string[] ["GrainSize", "requestor"] ("lkupTableNames"), "lkupTableNames"=string[] ["ThreatDetails", "Submitters"], "RefNumArray"=w2343) -> ("error OUT"=w2340:errorcluster)  [unwired: 3 in]
        n1334 = flat-sequence {
          frame #0 {
            n1335 = local write "RefreshMetadata"(FALSE ("UpdateMetadata")) -> ()
            n1336 = local write "TimeNow"("Connecting to BIMS Server . . ." ("TimeNow")) -> ()
          }
        }
        n1337 = call "Create local tables from Server DB.vi"("error in"=w2340, "Site"="Site", "tableNames"=string[] ["Threats", "ThreatDetails", "ThreatCalibers", "Mfrs", "SampleStyles", "SampleSpecs", "FiberTypes"]) -> ("error out"=w2368:errorcluster)  [unwired: 1 in, 7 out]
        n1338 = call "Fill Lists From DB (3rd Pass).vi"("error IN"=w2368) -> ("error OUT"=w2348:errorcluster)  [unwired: 3 in, 3 out]
        n1339 = control-ref of="ModelMfrs"() -> (w2355:refnum<vi>)
        n1340 = property class="Ring (strict)"(reference=w2355, error in=w2348) -> (reference out=w2354:refnum<vi>, error out=w2353:errorcluster, "Strings []"=w2352:string[])
        n1341 = Delete From Array(array=w2352, length=1, index=0) -> (array with subset deleted=w2351:string[])  [unwired: 1 out]
        n1342 = property class="Ring (strict)"(reference=w2354, error in=w2353, "Strings []"=w2351) -> (error out=w2347:errorcluster)  [unwired: 1 out]
        n1343 = case shown="No Error" w2347 {
          selector: w2347 -> [w2385 w2388]
          tunnel: [w2385 w2388] -> w2364
          frame No Error {
            n1344 = local write "TimeNow"("Collector Metadata is READY!" ("TimeNow")) -> ()
            n1345 = Wait (ms)(milliseconds to wait=u32 2000) -> ()  [unwired: 1 out]
          }
          frame Error {
            n1346 = call <vilib>:"General Error Handler.vi"("error in (no error)"=w2388) -> ()  [unwired: 2 in, 13 out]
          }
        }
        n1347 = property on="Loading" class="Ring (strict)"(error in=w2364, "Visible"=FALSE) -> (error out=w2363:errorcluster)  [unwired: 1 in, 1 out]
      }
      event "loadingUnits": Value Change {
        n1348 = local read "Powder Loading"() -> (w2392:sgl)
        n1349 = event-data() -> ("NewVal"=w2391:enum32{"grams", "grains"})  [unwired: 6 out]
        n1350 = case shown="\"grams\", Default" w2391 {
          tunnel: w2392 -> [w2397 w2398]
          frame "grams", Default {
            n1351 = Multiply(x=w2397, y=sgl 0.06479891) -> (x*y=w2395:sgl)
            n1352 = local write "Powder Loading"(w2395) -> ()
          }
          frame "grains" {
            n1353 = Multiply(x=w2398, y=sgl 15.432359) -> (x*y=w2399:sgl)
            n1354 = local write "Powder Loading"(w2399) -> ()
          }
        }
      }
      event "clearErrors": Value Change {
        w2401 = errorcluster {"status"=FALSE, "code"=0, "source"=""} ("error in")
        n1355 = event-data() -> ()  [unwired: 7 out]
        n1356 = local write "SMErr"(w2401) -> ()
      }
    }
    "U/I EvErr" <- w1890
    "booleanDump" <- w1889
  }
